vi "rio_veloster9.vi"() -> ()   [LabVIEW 2015]
uses:
  <vilib>/rvi/interface/nirviOpenFPGA/nirviOpenFPGA.xnode
  <vilib>/rvi/interface/nirviMethod/nirviMethod.xnode
  G_rio.vi
  <vilib>/rvi/interface/nirviReadWriteControl/nirviReadWriteControl.xnode
  <vilib>/Utility/error.llb/Error Cluster From Error Code.vi
  <vilib>/rvi/interface/Simulation/niFpgaSimulationCallBeginRW.vi
  <vilib>/rvi/errors/niLvFpgaAdjustHostInterfaceError.vi
  <vilib>/xnet/xnet.llb/XNET Frame Type CAN.ctl
  <vilib>/xnet/xnet.llb/XNET Frame CAN.ctl
  <vilib>/rvi/errors/niLvFpgaMergeErrorWithErrorCode.vi
  <resource>/objmgr/xnet.rc
  NiFpgaLv.dll
  <vilib>/FPGAPlugInAG/Dynamic/niLvFpga_ReadFifo_Dynamic.vi
  <vilib>/Instr/_visa.llb/VISA Configure Serial Port (Instr).vi
  <vilib>/Analysis/Matrix/NI_Matrix.lvlib
  <vilib>/Analysis/Matrix/Numeric/Multiply/Multiply - RM,RM.vi
  <vilib>/Analysis/Matrix/Numeric/Add/Add - RM,RM.vi
  <vilib>/Analysis/NI_AALBase.lvlib
  <vilib>/Analysis/Matrix/Numeric/Subtract/Subtract - RM,RM.vi
  <vilib>/Analysis/Matrix/Numeric/Conversions/Array To Matrix - RA.vi
  <vilib>/xnet/xnet.llb/XNET Create Session (Frame Input Stream).vi
  <vilib>/xnet/xnet.llb/XNET Create Session (Frame Output Stream).vi
  <vilib>/Analysis/Matrix/Numeric/Conversions/Array To Matrix - RA2.vi
  <vilib>/Analysis/baseanly.llb/Real Inverse Matrix.vi
  <vilib>/Analysis/Matrix/Numeric/Multiply/Multiply - R,RM.vi
  <vilib>/Analysis/Matrix/Numeric/Conversions/Matrix To Array - RM.vi
  <vilib>/xnet/xnet.llb/XNET Write (Frame CAN).vi
  <vilib>/xnet/xnet.llb/XNET Read (Frame CAN).vi
  <vilib>/FPGAPlugInAG/Dynamic/niLvFpga_Abort_Dynamic.vi
  <vilib>/FPGAPlugInAG/Dynamic/niLvFpga_Run_Dynamic.vi
  FPGA Bitfiles/autonomous_FPGATarget2_fpga4_FZHAM7r+pqE.lvbitx
  fpga/fpga4.vi
  <vilib>/FPGAPlugInAG/cRIO-9113/niLvFpga_Open_cRIO-9113.vi
  <vilib>/rvi/interface/common/dynamic/niFpgaDynamicAddResources.vi
panel:
  out "battery voltage 2":dbl
  out "FPGA VI Reference Out":refnum<k20>
  in  "Ref steer manual 2":dbl(knob) min=-20.48 max=20.46 step=0.01 scale=-20.48..20.46
  in  "steer2":bool
  in  "steer limit":dbl=100.0
  in  "buzz":bool
  out "hcount":u64=1
  out "hbias":dbl
  out "vcount":u64=1
  out "vgain":dbl=1.0
  in  "heading gain":dbl=1.414
  in  "pos gain":dbl=4.0
  out "dy":dbl
  out "dx":dbl
  out "initP":dbl
  out "dy_hat":dbl
  out "dx_hat":dbl
  out "dh":dbl
  out "initH":dbl
  out "dh_hat":dbl
  out "Pos_time 10":i32
  out "T PWM":u16
  out "B PWM":u16
  out "solenoid":bool
  out "brk enc":u8
  out "shift lever":dbl
  in  "LCM":bool=TRUE
  out "mobileye":u8[](array[numeric])
  out "timer":u32
  out "Mobileye_time 100":u32
  out "H_GPS":dbl
  out "pos":dbl[](array[numeric])
  out "pos error":dbl
  in  "GPS init":bool=TRUE
  in  "Gear Manual":i32(slide)=1 scale=-1.0..1.0
  out "map":i32=2
  out "P, R, D":i32
  out "heading error":dbl
  out "POS init":bool
  out "VS_CAN":dbl
  in  "brake":bool
  in  "Slide":dbl(slide) min=-50.0 max=50.0 step=50.0 scale=-50.0..50.0
  out "novatel":refnum<visa-resource-name>
  in  "ublox":bool=TRUE
  out "rest":u8[](array[numeric])
  out "GPS_novatel_time":u32
  out "GPS_Ublox_time 100":u32
  out "Con_time 10":i32
  out "CAN_time 10":u32
  out "gps2":refnum<visa-resource-name>
  out "gps1":refnum<visa-resource-name>
  out "Heading":dbl
  out "ecef ref":dbl[](array[numeric])
  out "h_gps":dbl
  out "pos_gps":dbl[](array[numeric]) format="%#_19f"
  out "get heading":bool
  out "get position":bool
  out "dt":dbl
  out "rt":dbl
  out "CAN Comm Enabled":bool
  in  "SPAS Enable":bool=TRUE
  in  "file write":bool
  out "data write":refnum<file>
  out "file rw error":errorcluster
  out "car can error":errorcluster
  out "CAN write":refnum<k21>
  out "CAN read":refnum<k21>
  out "Ref steer":dbl=1.0
  in  "Steer input":bool=TRUE
  in  "Ref steer manual":dbl(knob) scale=-550.0..550.0
  out "Ref vel":dbl=1.0
  in  "Ref vel manual":dbl
  in  "Velocity input":bool
  out "Auto":bool
  out "Run":bool
  out "E - STOP":bool
  out "Throttle Enable":bool=TRUE
  # "P"
  # "R"
  # "D"
  # "Ref steer manual"
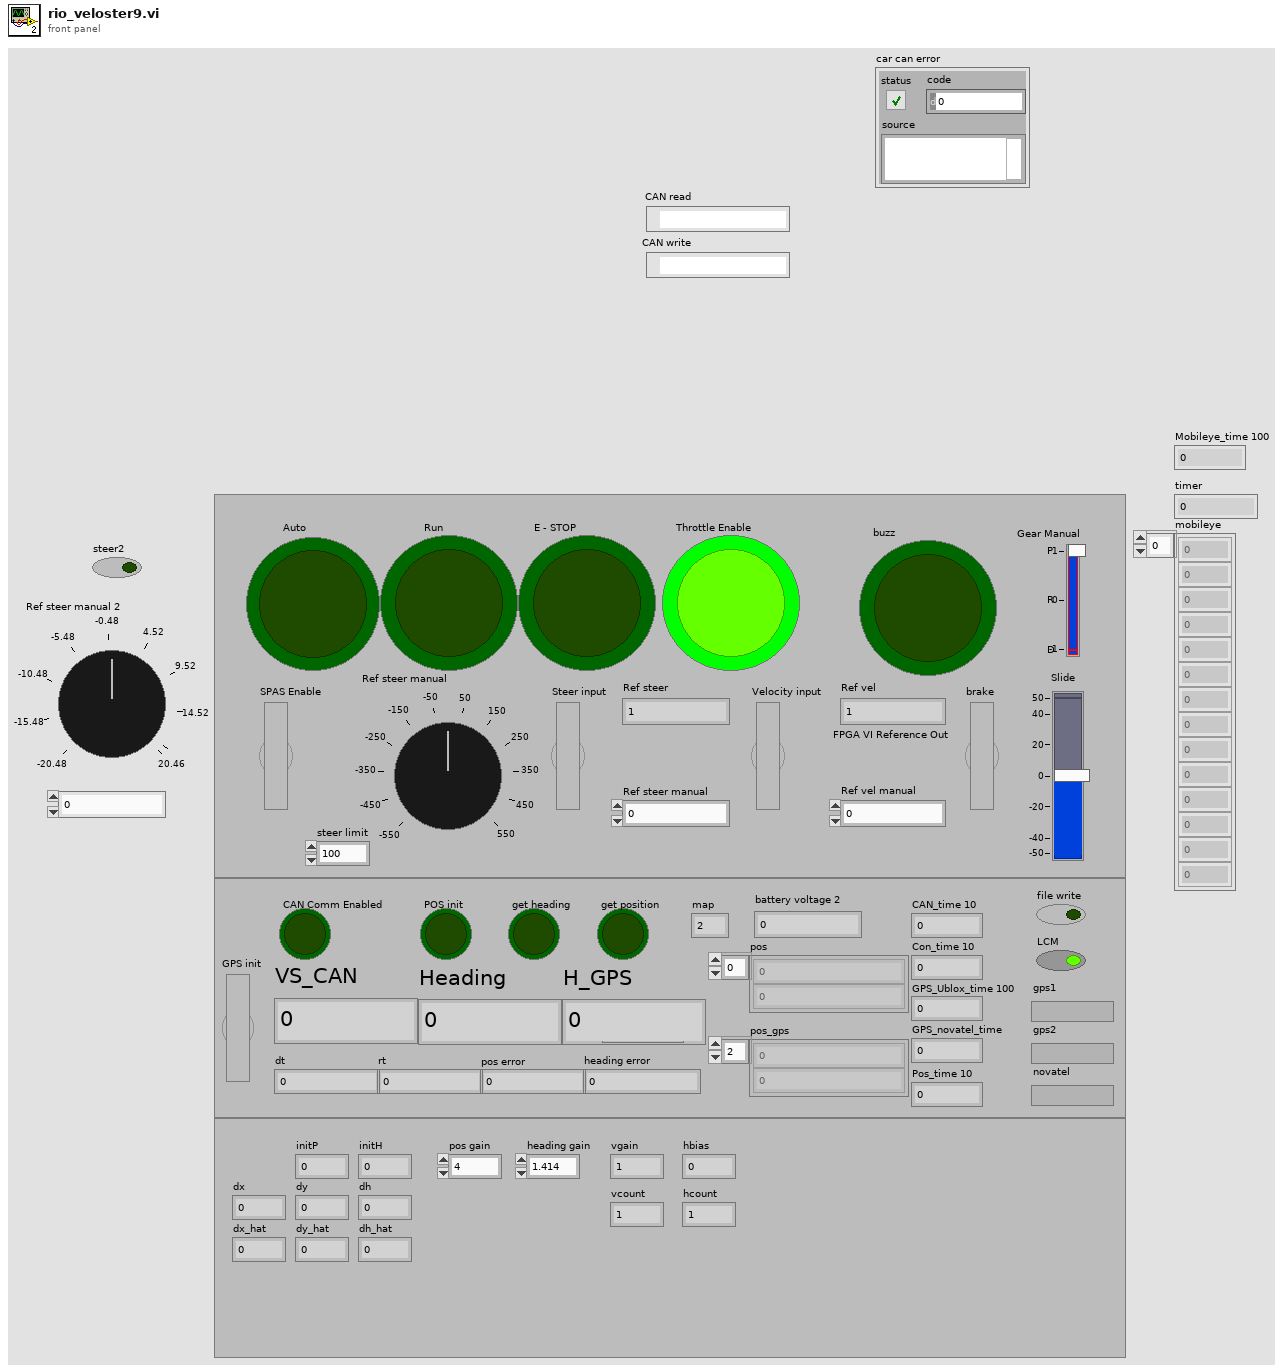
[diagram p1: front panel]
types:
  T1 = enum16{"open", "replace", "create", "open or create", "replace or create", "replace or create with confirmation"}
  T2 = typedef "XNET Frame CAN.ctl" = cluster{"timestamp":timestamp, "payload":u8[], "identifier":u32, "type":T3, "extended?":bool, "echo?":bool}
  T3 = typedef "XNET Frame Type CAN.ctl" = u8
  T4 = cluster{"connection ID":refnum<k16>, "net address":u32, "port":u16}
  T5 = cluster{"hash":i64, "sys time":i64, "mobileye":u8[]}
  T6 = cluster{"hash":i64, "sys time":i64, "time":dbl, "x":dbl, "y":dbl, "h":dbl, "numSV":i32, "postype":i32, "lag":i32, "hordev":dbl, "lat":dbl, "lon":dbl, "hgt":dbl, "map_idx":i32}
  T7 = cluster{"LCC[0]":dbl, "LCC[1]":dbl, "LCC[2]":dbl, "LCC[3]":dbl, "LCC[4]":dbl, "LCC[5]":dbl, "LCC[6]":dbl, "LCC[7]":dbl, "LCC[8]":dbl, "LCC[9]":dbl, "LCC[10]":dbl, "LCC[11]":dbl, "LCC[12]":dbl, "LCC[13]":dbl, "LCC[14]":dbl}
  T8 = cluster{"hash":i64, "sys time":i64, "time":dbl, "speed":dbl, "heading":dbl, "lat":dbl, "lon":dbl}
  T9 = cluster{"vel[0]":dbl, "vel[1]":dbl, "vel[2]":dbl, "vel[3]":dbl, "vel[4]":dbl, "vel[5]":dbl, "vel[6]":dbl}
  T10 = cluster{"output[0]":dbl, "output[1]":dbl, "output[2]":dbl, "output[3]":dbl, "output[4]":dbl, "output[5]":dbl, "output[6]":dbl, "output[7]":dbl, "output[8]":dbl, "output[9]":dbl, "output[10]":dbl, "output[11]":dbl, "output[12]":dbl, "output[13]":dbl, "output[14]":dbl}
  T11 = cluster{"output[0]":dbl, "output[1]":dbl, "output[2]":dbl, "output[3]":dbl, "output[4]":dbl, "output[5]":dbl, "output[6]":dbl}
  T12 = cluster{"hash":i64, "sys time":i64, "time":dbl, "yaw_rate":dbl, "mdps torque":dbl, "mdps str_ang":dbl, "VS_CAN":dbl, "lat_accel":dbl, "mcp":dbl, "accel pedal value":dbl, "tps":dbl, "odometer":dbl, "battery voltage":dbl, "WHL_SPD_RR":dbl, "WHL_SPD_RL":dbl, "WHL_SPD_FR":dbl, "WHL_SPD_FL":dbl}
  T13 = cluster{"hash":i64, "sys time":i64, "ref_vel":dbl, "ref_steer":dbl}
  T14 = cluster{"hash":i64, "sys time":i64, "Auto":bool, "Run":bool, "Solenoid":bool, "T lim":bool, "brk_enc":u8, "B PWM":u16, "T PWM":u16, "ref_vel":dbl, "ref_bkr_enc":dbl, "ref_apv":dbl, "ref_steer":dbl}
  T15 = typedef "NI_Matrix.lvlib/RealMatrix.ctl" = dbl[][]
  T16 = cluster{"hash":i64, "sys time":i64, "dt":dbl, "x":dbl, "y":dbl, "speed":dbl, "heading":dbl, "yaw_rate":dbl}
  T17 = cluster{"Real 2D Array[0]":dbl, "Real 2D Array[1]":dbl, "Real 2D Array[2]":dbl, "Real 2D Array[3]":dbl, "Real 2D Array[4]":dbl}
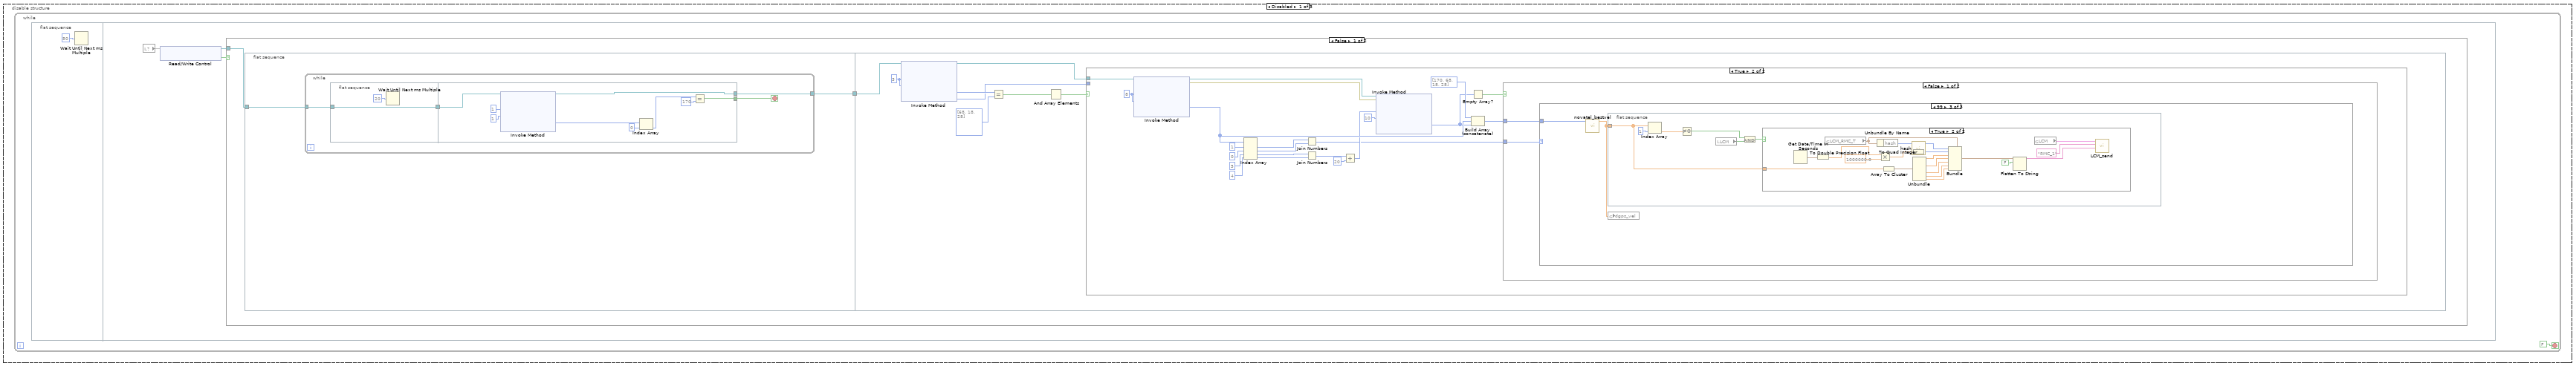
[diagram p5: hidden frame]
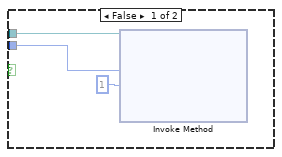
[diagram p6: hidden frame]
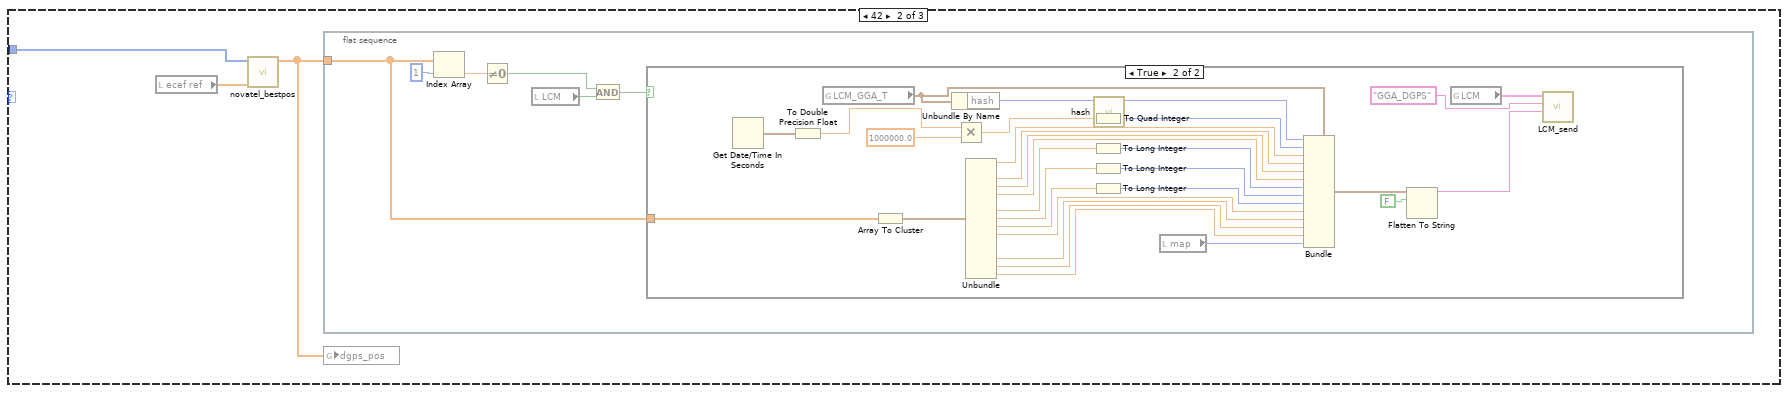
[diagram p8: hidden frame]
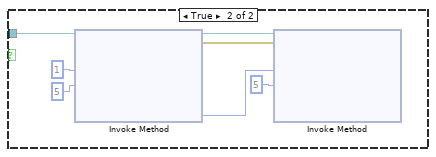
[diagram p12: hidden frame]
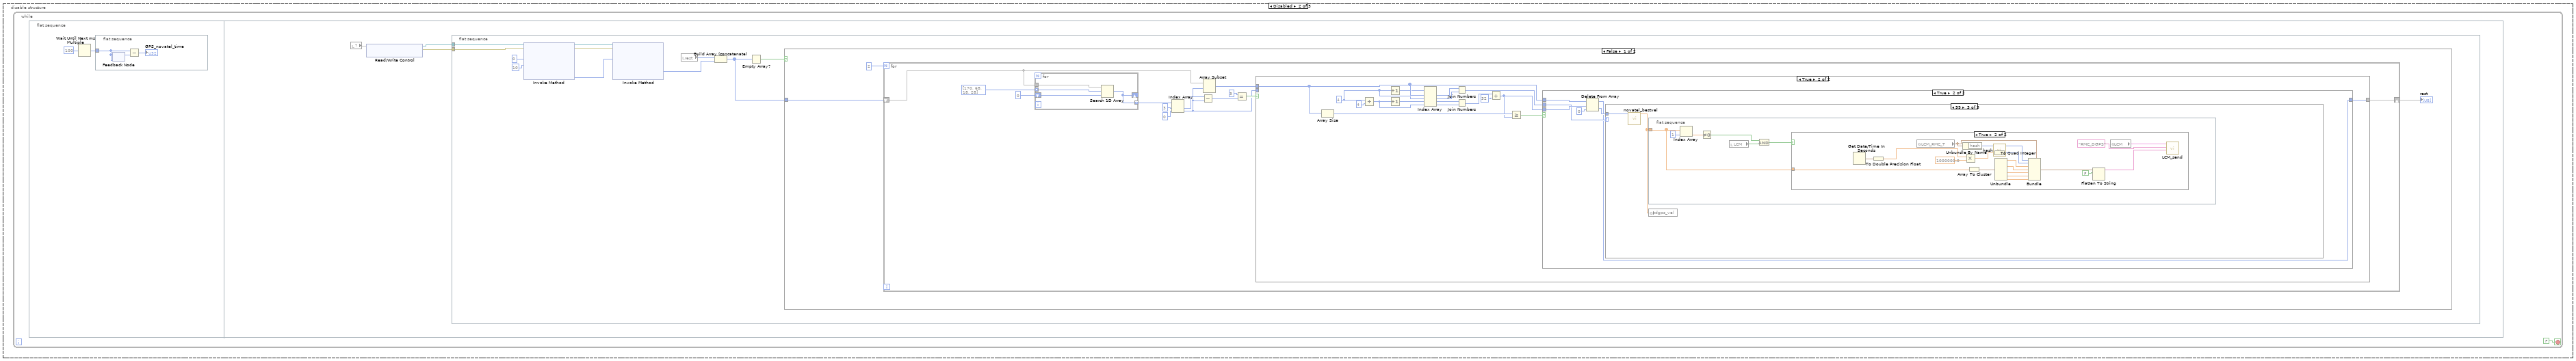
[diagram p13: hidden frame]
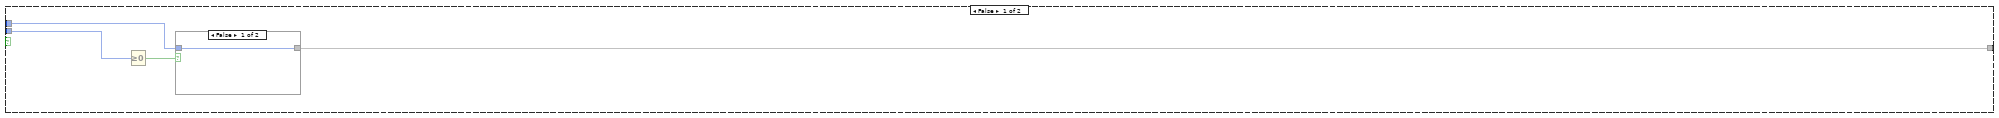
[diagram p14: hidden frame]
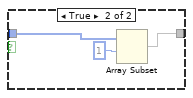
[diagram p15: hidden frame]
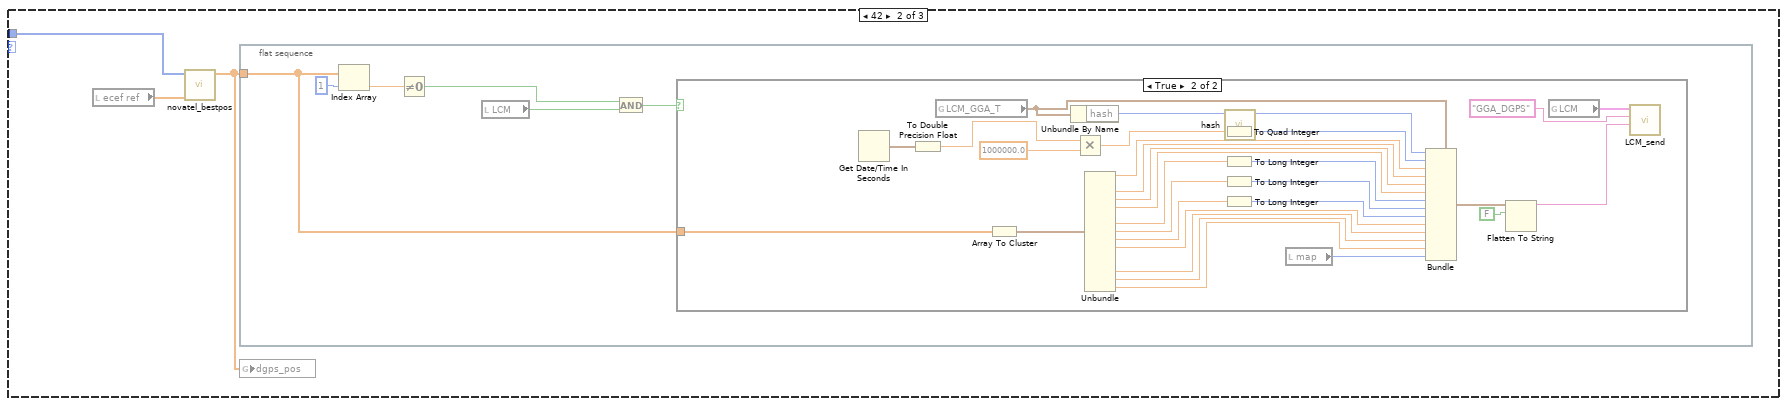
[diagram p18: hidden frame]
diagram:
  n1 = flat-sequence {
    frame #0 {
      n2 = xnode "Open FPGA VI Reference"() -> ("FPGA VI Reference Out"=w6:refnum<k20>, "error out"=w5:errorcluster)  [unwired: 2 in]
      n3 = xnode "Invoke Method"("FPGA VI Reference In"=w6, "error in"=w5) -> ("FPGA VI Reference Out"=w4:refnum<k20>, "error out"=w3:errorcluster)
      n4 = xnode "Invoke Method"("FPGA VI Reference In"=w4, "error in"=w3, "Wait Until Done (F)"=FALSE) -> ("FPGA VI Reference Out"=→"FPGA VI Reference Out":refnum<k20>)  [unwired: 1 out]
    }
    frame #1 {
      n5 = disable-structure shown="Enabled" {
        frame Enabled {
          n6 = call-poly "VISA Configure Serial Port"("VISA resource name"=refnum<visa-resource-name> "ASRL1::INSTR", "timeout (10sec)"=u32 10, "baud rate (9600)"=u32 9600) -> ("VISA resource name out"=→"novatel":refnum<visa-resource-name>)  [unwired: 11 in, 1 out]
          n7 = call-poly "VISA Configure Serial Port"("VISA resource name"=refnum<visa-resource-name> "USB0::0x1546::0x01A6::NI-VISA-1::1::RAW", "timeout (10sec)"=u32 1, "baud rate (9600)"=u32 115200) -> ("VISA resource name out"=→"gps1":refnum<visa-resource-name>)  [unwired: 11 in, 1 out]
          n8 = call-poly "VISA Configure Serial Port"("VISA resource name"=refnum<visa-resource-name> "USB0::0x1546::0x01A6::NI-VISA-0::1::RAW", "timeout (10sec)"=u32 1, "baud rate (9600)"=u32 115200) -> ("VISA resource name out"=→"gps2":refnum<visa-resource-name>)  [unwired: 11 in, 1 out]
        }
        frame Disabled {
        }
      }
      n9 = flat-sequence {
        frame #0 {
          w51 = 2 ("map")
          n10 = call "getecefdcmref.vi"("map"=w51) -> ("XYZ"=→"ecef ref":dbl[])  [unwired: 10 in, 4 out]
          "map" <- w51
        }
        frame #1 {
          w53 = FALSE ("GPS init")
          w54 = 0.0 ("Ref_vel_planner")
          n11 = global write "G_rio.vi" "T lim counter 2"(u16 300 ("T lim counter 2")) -> ()
          n12 = global write "G_rio.vi" "Ref_steer_planner"(w54) -> ()
          n13 = global write "G_rio.vi" "Ref_vel_planner"(w54) -> ()
          n14 = local write "brake"(w53) -> ()
          n15 = local write "rest"(u8[] [] ("rest")) -> ()
          n16 = local write "rest"(u8[] [] ("rest")) -> ()
          n17 = local write "Velocity input"(w53) -> ()
          n18 = local write "GPS init"(w53) -> ()
          "POS init" <- TRUE ("pos linit")
        }
      }
      n19 = flat-sequence {
        frame #0 {
          n20 = property class="XNET System"() -> (error out=w22:errorcluster, "Devices"=w35:refnum<k21>[])  [unwired: 2 in, 1 out]
          n21 = Index Array(array=w35, index=0) -> (element=w20:refnum<k21>)
          n22 = property class="XNET Device"(reference=w20, error in=w22) -> (error out=→"car can error":errorcluster, "Intfs"=w33:refnum<k21>[])  [unwired: 1 out]
          n23 = Index Array(array=w33, index=0) -> (element=w24:refnum<k21>)
          n24 = call-poly <vilib>:"XNET Create Session.vi"("cluster (:memory:)"=refnum<k21> "nixnet_example.CAN_Cluster", "interface"=w24) -> ("session out"=w25:refnum<k21>)  [unwired: 1 in, 12 out]
          n25 = call-poly <vilib>:"XNET Create Session.vi"("cluster (:memory:)"=refnum<k21> "nixnet_example.CAN_Cluster", "interface"=w24) -> ("session out"=w31:refnum<k21>)  [unwired: 1 in, 12 out]
          n26 = property class="XNET Session"(reference=w25, "Intf.BaudRate"=u32 500000 ("Interface:Baud Rate")) -> (reference out=w27:refnum<k21>)  [unwired: 1 in, 1 out]
          n27 = property class="XNET Session"(reference=w31, "Intf.BaudRate"=u32 500000 ("Interface:Baud Rate")) -> (reference out=w29:refnum<k21>)  [unwired: 1 in, 1 out]
          n28 = call <vilib>:"XNET Start.vi"("session in"=w27) -> ("session out"=→"CAN read":refnum<k21>)  [unwired: 1 in, 13 out]
          n29 = call <vilib>:"XNET Start.vi"("session in"=w29) -> ("session out"=→"CAN write":refnum<k21>)  [unwired: 1 in, 13 out]
        }
      }
      n30 = case shown="True" "file write" {
        frame False {
        }
        frame True {
          n31 = Open/Create/Replace File(file path (use dialog)=path "c:/datasave", operation (0:open)=T1."replace or create", access (0:read/write)=enum16{"read/write", "read-only", "write-only"}."write-only") -> (refnum out=→"data write":refnum<file>, cancelled=w61:bool, error out=→"file rw error":errorcluster)  [unwired: 3 in]
          n32 = Not(x=w61) -> (.not. x?=w60:bool)
          n33 = local write "file write"(w60) -> ()
        }
      }
      n34 = case shown="True" "LCM" {
        frame False {
        }
        frame True {
          n35 = flat-sequence {
            frame #0 {
              w15 = u16 7667 ("port")
              n36 = Decrement(x=w15) -> (x-1=w14:u16)
              n37 = UDP Open(11:w14) -> (port=w17:refnum<k16>)  [unwired: 4 in, 2 out]
              n38 = global read "G_rio.vi" "LCM"() -> (w19:T4)
              n39 = Bundle By Name(cluster=w19, "port"=w15, "connection ID"=w17, "net address"=u32 4294967295) -> (w18:T4)
              n40 = global write "G_rio.vi" "LCM"(w18) -> ()
            }
          }
          n41 = flat-sequence {
            frame #0 {
              w9 = u16 7668 ("port")
              n42 = global read "G_rio.vi" "LCM PC"() -> (w13:T4)
              n43 = UDP Open(11:w9) -> (port=w11:refnum<k16>)  [unwired: 4 in, 2 out]
              n44 = Bundle By Name(cluster=w13, "port"=w9, "connection ID"=w11, "net address"=u32 0) -> (w12:T4)
              n45 = global write "G_rio.vi" "LCM PC"(w12) -> ()
            }
          }
        }
      }
    }
    frame #2 {
      (unwired) FALSE
      n46 = disable-structure shown="Enabled" {
        frame Enabled {
          n47 = while {
            stop <- FALSE stop-if-true
            n48 = flat-sequence {
              frame #0 {
                n49 = Wait Until Next ms Multiple(millisecond multiple=u32 100) -> (millisecond timer value=w1290:u32)
                n50 = flat-sequence {
                  tunnel: w1290 -> [w1292]
                  frame #0 {
                    n51 = feedback #1(w1292) -> (w1293:u32)
                    n52 = feedback-in #1(w1292) -> ()
                    n53 = Subtract(x=w1292, y=w1293) -> (x-y=→"Mobileye_time 100":u32)
                  }
                }
              }
              frame #1 {
                n54 = local read "FPGA VI Reference Out"() -> (w1339:refnum<k20>)
                n55 = xnode "Read/Write Control"("FPGA VI Reference In"=w1339) -> ("m 700"=w1299:u8[], "m 760"=w1335:u8[], "m 710"=w1324:u8[], "m 711"=w1320:u8[], "m 720"=w1318:u8[], "m 721"=w1317:u8[], "m 722"=w1316:u8[], "m 723"=w1315:u8[], "m 724"=w1314:u8[], "m 725"=w1313:u8[], "m 726"=w1312:u8[], "m 727"=w1311:u8[], "m 728"=w1310:u8[], "m 729"=w1309:u8[])  [unwired: 1 in, 2 out]
                n56 = Build Array(w1318, w1317, w1316, w1315, w1314, w1313, w1312, w1311, w1310, w1309) -> (w1308:u8[][])
                n57 = Index Array(array=w1299, index #1=4 ("index"), index #4=8 ("index"), index #5=11 ("index")) -> (element #1=w1332:u8, element #2=w1331:u8, element #3=w1330:u8, element #4=w1329:u8, element #5=w1328:u8)  [unwired: 2 in]
                n58 = Array Subset(array=w1320, index=6, length=6) -> (w1319:u8[])
                n59 = Array Subset(array=w1299, index=0, length=4) -> (w1296:u8[])
                n60 = Array Subset(array=w1335, index=4, length=3) -> (w1327:u8[])
                n61 = Array Subset(array=w1324, index=5, length=7) -> (w1323:u8[])
                n62 = Index Array(array=w1296, index #1=0 ("index")) -> (element #1=w1305:u8, element #2=w1304:u8, element #3=w1303:u8, element #4=w1302:u8)  [unwired: 3 in]
                n63 = Build Array (concatenate)(w1296, w1332, w1331, w1330, w1329, w1328, w1327, w1323, w1319) -> (w1307:u8[])
                n64 = Join Numbers(hi=w1305, lo=w1304) -> ((hi.lo)=w1301:u16)
                n65 = Join Numbers(hi=w1303, lo=w1302) -> ((hi.lo)=w1300:u16)
                n66 = for {
                  tunnel: w1308 -> [w1341] mode=indexing
                  shift-right: [w1344] -> w1294
                  shift-left: w1307 -> [w1345]
                  n67 = Array Subset(array=w1341, index=4, length=8) -> (w1340:u8[])
                  n68 = disable-structure shown="Enabled" {
                    disable-tunnel: [w1348 TRUE ("lsb carry out")] -> w1346
                    disable-tunnel: w1340 -> [w1347 _]
                    frame Disabled {
                      n69 = Index Array(array=w1347, index=0) -> (element=w1350:u8)
                      n70 = Rotate Right With Carry(2:w1350, 3:FALSE ("carry")) -> (1:w1348:bool)  [unwired: 1 out]
                    }
                    frame Enabled {
                    }
                  }
                  n71 = case shown="True" w1346 {
                    tunnel: w1345 -> [w1353 w1356]
                    tunnel: [w1353 w1355] -> w1344
                    tunnel: w1340 -> [_ w1354]
                    frame False {
                    }
                    frame True {
                      n72 = Build Array (concatenate)(w1356, w1354) -> (w1355:u8[])
                    }
                  }
                }
                "mobileye" <- w1294
                n73 = Join Numbers(hi=w1301, lo=w1300) -> ((hi.lo)=→"timer":u32)
              }
              frame #2 {
                n74 = local read "LCM"() -> (w1357:bool)
                n75 = case shown="True" w1357 {
                  frame False {
                    n76 = local read "mobileye"() -> (w1358:u8[])
                    n77 = shared-variable "veloster\\sharedvari.lvlib\\mobileye"(w1358) -> ()  [unwired: 1 in, 1 out]
                  }
                  frame True {
                    n78 = Get Date/Time In Seconds() -> (seconds since 1Jan1904=w1363:timestamp)
                    n79 = To Double Precision Float(number=w1363) -> (double precision float=w1362:dbl)
                    n80 = global read "G_rio.vi" "LCM_EYE_RAW_T"() -> (w1372:T5)
                    n81 = Unbundle By Name(w1372) -> ("hash"=w1371:i64)
                    n82 = Multiply(x=w1362, y=1000000.0) -> (x*y=w1360:dbl)
                    n83 = local read "mobileye"() -> (w1364:u8[])
                    n84 = call "hash.vi"("input"=w1371) -> ("output"=w1370:i64)  [unwired: 10 in]
                    n85 = To Quad Integer(1:w1360) -> (0:w1359:i64)
                    n86 = Bundle By Name(cluster=w1372, "hash"=w1370, "sys time"=w1359, "mobileye"=w1364) -> (w1369:T5)
                    n87 = Flatten To String(anything=w1369, prepend array or string size? (T)=FALSE) -> (data string=w1367:string)  [unwired: 2 in, 2 out]
                    n88 = global read "G_rio.vi" "LCM"() -> (w1368:T4)
                    n89 = call "LCM_send.vi"("DATA"=w1367, "ID"="EYE_RAW_T", "LCM"=w1368) -> ()  [unwired: 6 in, 3 out]
                  }
                }
              }
            }
          }
        }
        frame Disabled {
        }
      }
      n90 = disable-structure shown="Enabled" {
        frame Disabled {
          n91 = while {
            stop <- FALSE stop-if-true
            n92 = flat-sequence {
              frame #0 {
                n93 = Wait Until Next ms Multiple(millisecond multiple=u32 50) -> ()  [unwired: 1 out]
              }
              frame #1 {
                n94 = local read item#-1() -> (w79)
                n95 = xnode "Read/Write Control"("FPGA VI Reference In"=w79) -> ("FPGA VI Reference Out"=w77:refnum<k20>, "Connection error GPS 1"=w78:bool)  [unwired: 1 in, 1 out]
                n96 = case shown="False" w78 {
                  tunnel: w77 -> [w81 w201]
                  frame False {
                    n97 = flat-sequence {
                      tunnel: w81 -> [w83]
                      tunnel: [w82] -> w80
                      tunnel: w80 -> [w102]
                      frame #0 {
                        n98 = while {
                          tunnel: w83 -> [w87]
                          tunnel: [w85] -> w82
                          stop <- w86 stop-if-true
                          n99 = flat-sequence {
                            tunnel: w87 -> [w89]
                            tunnel: [w89] -> w84
                            tunnel: [w92] -> w86
                            tunnel: [w91] -> w85
                            tunnel: w84 -> [w98]
                            frame #0 {
                              n100 = Wait Until Next ms Multiple(millisecond multiple=u32 20) -> ()  [unwired: 1 out]
                            }
                            frame #1 {
                              n101 = xnode "Invoke Method"("FPGA VI Reference In"=w98, "Number of Elements"=u32 1, "Timeout (ms)"=1) -> ("FPGA VI Reference Out"=w91:refnum<k20>, "Data"=w93:u8[])  [unwired: 1 in, 2 out]
                              n102 = Index Array(array=w93, index=0) -> (element=w95:u8)
                              n103 = Equal?(x=w95, y=u8 170) -> (x = y?=w92:bool)
                            }
                          }
                        }
                      }
                      frame #1 {
                        w103 = u32 3 ("Number of Elements")
                        n104 = xnode "Invoke Method"("FPGA VI Reference In"=w102, "Number of Elements"=w103, "Timeout (ms)"=w103) -> ("FPGA VI Reference Out"=w101:refnum<k20>, "Data"=w105:u8[], "Elements Remaining"=w99:u32)  [unwired: 1 in, 1 out]
                        n105 = Equal?(x=w105, y=u8[] [68, 18, 28]) -> (x = y?=w106:bool[])
                        n106 = And Array Elements(Boolean array=w106) -> (logical AND=w100:bool)
                        n107 = case shown="True" w100 {
                          tunnel: w101 -> [w109 w114]
                          tunnel: w99 -> [w108 _]
                          frame False {
                            n108 = xnode "Invoke Method"("FPGA VI Reference In"=w109, "Number of Elements"=w108, "Timeout (ms)"=1) -> ()  [unwired: 1 in, 4 out]
                          }
                          frame True {
                            w110 = u32 8 ("Number of Elements")
                            n109 = xnode "Invoke Method"("FPGA VI Reference In"=w114, "Number of Elements"=w110, "Timeout (ms)"=w110) -> ("FPGA VI Reference Out"=w127:refnum<k20>, "error out"=w128:errorcluster, "Data"=w130:u8[])  [unwired: 1 in, 1 out]
                            n110 = Index Array(array=w130, index #1=1 ("index"), index #2=0 ("index"), index #3=5 ("index"), index #4=4 ("index")) -> (element #1=w117:u8, element #2=w118:u8, element #3=w122:u8, element #4=w123:u8)
                            n111 = Join Numbers(hi=w117, lo=w118) -> ((hi.lo)=w119:u16)
                            n112 = Join Numbers(hi=w122, lo=w123) -> ((hi.lo)=w124:u16)
                            n113 = Add(x=w124, y=u16 20) -> (x+y=w126:u16)
                            n114 = xnode "Invoke Method"("FPGA VI Reference In"=w127, "error in"=w128, "Number of Elements"=w126, "Timeout (ms)"=10) -> ("Data"=w112:u8[])  [unwired: 3 out]
                            n115 = Empty Array?(array=w112) -> (empty?=w111:bool)
                            n116 = Build Array (concatenate)(u8[] [170, 68, 18, 28], w130, w112) -> (w131:u8[])
                            n117 = case shown="False" w111 {
                              tunnel: w131 -> [w133 _]
                              tunnel: w119 -> [w132 _]
                              frame False {
                                n118 = case shown="99" w132 {
                                tunnel: w133 -> [_ w136 w174]
                                frame 0, Default {
                                }
                                frame 42 {
                                n119 = local read "ecef ref"() -> (w135:dbl[])
                                n120 = call "novatel_bestpos.vi"("ecef ref"=w135, "gps_data"=w136) -> ("LCC"=w134:dbl[])  [unwired: 9 in]
                                n121 = flat-sequence {
                                tunnel: w134 -> [w139]
                                frame #0 {
                                n122 = Index Array(array=w139, index=1) -> (element=w142:dbl)
                                n123 = Not Equal To 0?(x=w142) -> (x != 0?=w138:bool)
                                n124 = local read "LCM"() -> (w141:bool)
                                n125 = And(x=w138, y=w141) -> (x .and. y?=w137:bool)
                                n126 = case shown="True" w137 {
                                tunnel: w139 -> [_ w162]
                                frame False {
                                }
                                frame True {
                                n127 = Get Date/Time In Seconds() -> (seconds since 1Jan1904=w147:timestamp)
                                n128 = To Double Precision Float(number=w147) -> (double precision float=w146:dbl)
                                n129 = global read "G_rio.vi" "LCM_GGA_T"() -> (w171:T6)
                                n130 = Array To Cluster(array=w162) -> (cluster=w170:T7)
                                n131 = Unbundle By Name(w171) -> ("hash"=w167:i64)
                                n132 = Multiply(x=w146, y=1000000.0) -> (x*y=w144:dbl)
                                n133 = Unbundle(w170) -> ("LCC[0]"=w172:dbl, "LCC[2]"=w161:dbl, "LCC[3]"=w160:dbl, "LCC[4]"=w159:dbl, "LCC[6]"=w158:dbl, "LCC[7]"=w156:dbl, "LCC[8]"=w154:dbl, "LCC[9]"=w152:dbl, "LCC[12]"=w151:dbl, "LCC[13]"=w150:dbl, "LCC[14]"=w149:dbl)  [unwired: 4 out]
                                n134 = To Quad Integer(1:w144) -> (0:w143:i64)
                                n135 = To Long Integer(number=w158) -> (32bit integer=w157:i32)
                                n136 = To Long Integer(number=w156) -> (32bit integer=w155:i32)
                                n137 = To Long Integer(number=w154) -> (32bit integer=w153:i32)
                                n138 = call "hash.vi"("input"=w167) -> ("output"=w166:i64)  [unwired: 10 in]
                                n139 = local read "map"() -> (w148:i32)
                                n140 = Bundle(cluster=w171, "hash"=w166, "sys time"=w143, "time"=w172, "x"=w161, "y"=w160, "h"=w159, "numSV"=w157, "postype"=w155, "lag"=w153, "hordev"=w152, "lat"=w151, "lon"=w150, "hgt"=w149, "map_idx"=w148) -> (w168:T6)
                                n141 = Flatten To String(anything=w168, prepend array or string size? (T)=FALSE) -> (data string=w164:string)  [unwired: 2 in, 2 out]
                                n142 = global read "G_rio.vi" "LCM"() -> (w163:T4)
                                n143 = call "LCM_send.vi"("DATA"=w164, "ID"="GGA_DGPS", "LCM"=w163) -> ()  [unwired: 6 in, 3 out]
                                }
                                }
                                }
                                }
                                n144 = global write "G_rio.vi" "dgps_pos"(w134) -> ()
                                }
                                frame 99 {
                                n145 = call "novatel_bestvel.vi"("gps_data"=w174) -> ("vel"=w173:dbl[])  [unwired: 10 in]
                                n146 = flat-sequence {
                                tunnel: w173 -> [w176]
                                frame #0 {
                                n147 = Index Array(array=w176, index=1) -> (element=w179:dbl)
                                n148 = Not Equal To 0?(x=w179) -> (x != 0?=w180:bool)
                                n149 = local read "LCM"() -> (w178:bool)
                                n150 = And(x=w180, y=w178) -> (x .and. y?=w175:bool)
                                n151 = case shown="True" w175 {
                                tunnel: w176 -> [_ w199]
                                frame False {
                                }
                                frame True {
                                n152 = Get Date/Time In Seconds() -> (seconds since 1Jan1904=w185:timestamp)
                                n153 = To Double Precision Float(number=w185) -> (double precision float=w184:dbl)
                                n154 = global read "G_rio.vi" "LCM_RMC_T"() -> (w200:T8)
                                n155 = Unbundle By Name(w200) -> ("hash"=w196:i64)
                                n156 = Multiply(x=w184, y=1000000.0) -> (x*y=w182:dbl)
                                n157 = Array To Cluster(array=w199) -> (cluster=w198:T9)
                                n158 = call "hash.vi"("input"=w196) -> ("output"=w195:i64)  [unwired: 10 in]
                                n159 = To Quad Integer(1:w182) -> (0:w181:i64)
                                n160 = Unbundle(w198) -> ("vel[0]"=w190:dbl, "vel[2]"=w189:dbl, "vel[4]"=w188:dbl, "vel[5]"=w187:dbl, "vel[6]"=w186:dbl)  [unwired: 2 out]
                                n161 = Bundle(cluster=w200, "hash"=w195, "sys time"=w181, "time"=w190, "speed"=w189, "heading"=w188, "lat"=w187, "lon"=w186) -> (w191:T8)
                                n162 = Flatten To String(anything=w191, prepend array or string size? (T)=FALSE) -> (data string=w193:string)  [unwired: 2 in, 2 out]
                                n163 = global read "G_rio.vi" "LCM"() -> (w192:T4)
                                n164 = call "LCM_send.vi"("DATA"=w193, "ID"="RMC_1", "LCM"=w192) -> ()  [unwired: 6 in, 3 out]
                                }
                                }
                                }
                                }
                                n165 = global write "G_rio.vi" "dgps_vel"(w173) -> ()
                                }
                                }
                              }
                              frame True {
                              }
                            }
                          }
                        }
                      }
                    }
                  }
                  frame True {
                    n166 = xnode "Invoke Method"("FPGA VI Reference In"=w201, "Number of Elements"=u32 1, "Timeout (ms)"=5) -> ("FPGA VI Reference Out"=w205:refnum<k20>, "error out"=w206:errorcluster, "Elements Remaining"=w207:u32)  [unwired: 1 in, 1 out]
                    n167 = xnode "Invoke Method"("FPGA VI Reference In"=w205, "error in"=w206, "Number of Elements"=w207, "Timeout (ms)"=5) -> ()  [unwired: 4 out]
                  }
                }
              }
            }
          }
        }
        frame Disabled {
          n168 = while {
            stop <- FALSE stop-if-true
            n169 = flat-sequence {
              frame #0 {
                n170 = Wait Until Next ms Multiple(millisecond multiple=u32 100) -> (millisecond timer value=w209:u32)
                n171 = flat-sequence {
                  tunnel: w209 -> [w212]
                  frame #0 {
                    n172 = feedback #2(w212) -> (w213:u32)
                    n173 = feedback-in #2(w212) -> ()
                    n174 = Subtract(x=w212, y=w213) -> (x-y=→"GPS_novatel_time":u32)
                  }
                }
              }
              frame #1 {
                n175 = local read item#-1() -> (w216)
                n176 = xnode "Read/Write Control"("FPGA VI Reference In"=w216) -> ("FPGA VI Reference Out"=w215:refnum<k20>, "error out"=w214:errorcluster)  [unwired: 1 in, 1 out]
                n177 = flat-sequence {
                  tunnel: w215 -> [w227]
                  tunnel: w214 -> [w226]
                  frame #0 {
                    n178 = xnode "Invoke Method"("FPGA VI Reference In"=w227, "error in"=w226, "Number of Elements"=u32 0, "Timeout (ms)"=10) -> ("FPGA VI Reference Out"=w225:refnum<k20>, "error out"=w224:errorcluster, "Elements Remaining"=w223:u32)  [unwired: 1 out]
                    n179 = xnode "Invoke Method"("FPGA VI Reference In"=w225, "error in"=w224, "Number of Elements"=w223) -> ("Data"=w217:u8[])  [unwired: 1 in, 3 out]
                    n180 = local read "rest"() -> (w219:u8[])
                    n181 = Build Array (concatenate)(w219, w217) -> (w218:u8[])
                    n182 = Empty Array?(array=w218) -> (empty?=w220:bool)
                    n183 = case shown="False" w220 {
                      tunnel: w218 -> [w230 _]
                      frame False {
                        n184 = for {
                          N: 2 -> [_]
                          shift-right: [w234] -> w228
                          shift-left: w230 -> [w232]
                          n185 = for {
                            tunnel: w232 -> [w345]
                            tunnel: u8[] [170, 68, 18, 28] -> [w343] mode=indexing
                            shift-right: [w342] -> _
                            shift-left: 0 ("start index (0)") -> [w344]
                            tunnel: [w342] -> w241 mode=indexing
                            n186 = Search 1D Array(1D array=w345, element=w343, start index (0)=w344) -> (index of element=w342:i32)
                          }
                          n187 = Index Array(array=w241, index #1=3 ("index"), index #2=0 ("index")) -> (element #1=w238:i32, element #2=w231:i32)
                          n188 = Subtract(x=w238, y=w231) -> (x-y=w237:i32)
                          n189 = Array Subset(array=w232, index=w231) -> (w233:u8[])  [unwired: 1 in]
                          n190 = Equal?(x=3, y=w237) -> (x = y?=w235:bool)
                          n191 = case shown="True" w235 {
                            tunnel: w233 -> [w247 w256]
                            tunnel: [w246 w253] -> w234
                            tunnel: w231 -> [w245 _]
                            frame False {
                              n192 = Greater Or Equal To 0?(x=w245) -> (x >= 0?=w244:bool)
                              n193 = case shown="False" w244 {
                                tunnel: w247 -> [w248 w251]
                                tunnel: [w248 w249] -> w246
                                frame False {
                                }
                                frame True {
                                n194 = Array Subset(array=w251, index=1 ("length")) -> (w249:u8[])  [unwired: 1 in]
                                }
                              }
                            }
                            frame True {
                              w252 = 4 ("index")
                              n195 = Array Size(array=w256) -> (size(s)=w258:i32)
                              n196 = Add(x=w252, y=4) -> (x+y=w265:i32)
                              n197 = Increment(x=w252) -> (x+1=w268:i32)
                              n198 = Increment(x=w265) -> (x+1=w266:i32)
                              n199 = Index Array(array=w256, index #1=w268, index #2=w252, index #3=w266, index #4=w265) -> (element #1=w264:u8, element #2=w263:u8, element #3=w262:u8, element #4=w261:u8)
                              n200 = Join Numbers(hi=w264, lo=w263) -> ((hi.lo)=w254:u16)
                              n201 = Join Numbers(hi=w262, lo=w261) -> ((hi.lo)=w260:u16)
                              n202 = Add(x=w260, y=u16 32) -> (x+y=w255:u16)
                              n203 = Greater Or Equal?(x=w258, y=w255) -> (x >= y?=w257:bool)
                              n204 = case shown="True" w257 {
                                tunnel: w256 -> [_ w274]
                                tunnel: w255 -> [_ w273]
                                tunnel: w254 -> [_ w270]
                                tunnel: [_ w269] -> w253
                                frame False {
                                }
                                frame True {
                                n205 = Delete From Array(array=w274, length=w273, index=0) -> (deleted portion=w271:u8[], array with subset deleted=w269:u8[])
                                n206 = case shown="99" w270 {
                                tunnel: w271 -> [_ w277 w315]
                                frame 0, Default {
                                }
                                frame 42 {
                                n207 = local read "ecef ref"() -> (w276:dbl[])
                                n208 = call "novatel_bestpos.vi"("ecef ref"=w276, "gps_data"=w277) -> ("LCC"=w275:dbl[])  [unwired: 9 in]
                                n209 = flat-sequence {
                                tunnel: w275 -> [w280]
                                frame #0 {
                                n210 = Index Array(array=w280, index=1) -> (element=w283:dbl)
                                n211 = Not Equal To 0?(x=w283) -> (x != 0?=w279:bool)
                                n212 = local read "LCM"() -> (w282:bool)
                                n213 = And(x=w279, y=w282) -> (x .and. y?=w278:bool)
                                n214 = case shown="True" w278 {
                                tunnel: w280 -> [_ w303]
                                frame False {
                                }
                                frame True {
                                n215 = Get Date/Time In Seconds() -> (seconds since 1Jan1904=w288:timestamp)
                                n216 = To Double Precision Float(number=w288) -> (double precision float=w287:dbl)
                                n217 = global read "G_rio.vi" "LCM_GGA_T"() -> (w312:T6)
                                n218 = Array To Cluster(array=w303) -> (cluster=w311:T7)
                                n219 = Unbundle By Name(w312) -> ("hash"=w308:i64)
                                n220 = Multiply(x=w287, y=1000000.0) -> (x*y=w285:dbl)
                                n221 = Unbundle(w311) -> ("LCC[0]"=w313:dbl, "LCC[2]"=w302:dbl, "LCC[3]"=w301:dbl, "LCC[4]"=w300:dbl, "LCC[6]"=w299:dbl, "LCC[7]"=w297:dbl, "LCC[8]"=w295:dbl, "LCC[9]"=w293:dbl, "LCC[12]"=w292:dbl, "LCC[13]"=w291:dbl, "LCC[14]"=w290:dbl)  [unwired: 4 out]
                                n222 = To Quad Integer(1:w285) -> (0:w284:i64)
                                n223 = To Long Integer(number=w299) -> (32bit integer=w298:i32)
                                n224 = To Long Integer(number=w297) -> (32bit integer=w296:i32)
                                n225 = To Long Integer(number=w295) -> (32bit integer=w294:i32)
                                n226 = call "hash.vi"("input"=w308) -> ("output"=w307:i64)  [unwired: 10 in]
                                n227 = local read "map"() -> (w289:i32)
                                n228 = Bundle(cluster=w312, "hash"=w307, "sys time"=w284, "time"=w313, "x"=w302, "y"=w301, "h"=w300, "numSV"=w298, "postype"=w296, "lag"=w294, "hordev"=w293, "lat"=w292, "lon"=w291, "hgt"=w290, "map_idx"=w289) -> (w309:T6)
                                n229 = Flatten To String(anything=w309, prepend array or string size? (T)=FALSE) -> (data string=w305:string)  [unwired: 2 in, 2 out]
                                n230 = global read "G_rio.vi" "LCM"() -> (w304:T4)
                                n231 = call "LCM_send.vi"("DATA"=w305, "ID"="GGA_DGPS", "LCM"=w304) -> ()  [unwired: 6 in, 3 out]
                                }
                                }
                                }
                                }
                                n232 = global write "G_rio.vi" "dgps_pos"(w275) -> ()
                                }
                                frame 99 {
                                n233 = call "novatel_bestvel.vi"("gps_data"=w315) -> ("vel"=w314:dbl[])  [unwired: 10 in]
                                n234 = flat-sequence {
                                tunnel: w314 -> [w318]
                                frame #0 {
                                n235 = Index Array(array=w318, index=1) -> (element=w320:dbl)
                                n236 = Not Equal To 0?(x=w320) -> (x != 0?=w321:bool)
                                n237 = local read "LCM"() -> (w316:bool)
                                n238 = And(x=w321, y=w316) -> (x .and. y?=w317:bool)
                                n239 = case shown="True" w317 {
                                tunnel: w318 -> [_ w340]
                                frame False {
                                }
                                frame True {
                                n240 = Get Date/Time In Seconds() -> (seconds since 1Jan1904=w326:timestamp)
                                n241 = To Double Precision Float(number=w326) -> (double precision float=w325:dbl)
                                n242 = global read "G_rio.vi" "LCM_RMC_T"() -> (w341:T8)
                                n243 = Unbundle By Name(w341) -> ("hash"=w337:i64)
                                n244 = Multiply(x=w325, y=1000000.0) -> (x*y=w323:dbl)
                                n245 = Array To Cluster(array=w340) -> (cluster=w339:T9)
                                n246 = To Quad Integer(1:w323) -> (0:w322:i64)
                                n247 = call "hash.vi"("input"=w337) -> ("output"=w336:i64)  [unwired: 10 in]
                                n248 = Unbundle(w339) -> ("vel[0]"=w331:dbl, "vel[2]"=w330:dbl, "vel[4]"=w329:dbl, "vel[5]"=w328:dbl, "vel[6]"=w327:dbl)  [unwired: 2 out]
                                n249 = Bundle(cluster=w341, "hash"=w336, "sys time"=w322, "time"=w331, "speed"=w330, "heading"=w329, "lat"=w328, "lon"=w327) -> (w332:T8)
                                n250 = Flatten To String(anything=w332, prepend array or string size? (T)=FALSE) -> (data string=w334:string)  [unwired: 2 in, 2 out]
                                n251 = global read "G_rio.vi" "LCM"() -> (w333:T4)
                                n252 = call "LCM_send.vi"("DATA"=w334, "ID"="RMC_DGPS", "LCM"=w333) -> ()  [unwired: 6 in, 3 out]
                                }
                                }
                                }
                                }
                                n253 = global write "G_rio.vi" "dgps_vel"(w314) -> ()
                                }
                                }
                                }
                              }
                            }
                          }
                        }
                        "rest" <- w228
                      }
                      frame True {
                      }
                    }
                  }
                }
              }
            }
          }
        }
        frame Enabled {
          n254 = while {
            stop <- FALSE stop-if-true
            n255 = flat-sequence {
              frame #0 {
                n256 = Wait Until Next ms Multiple(millisecond multiple=u32 50) -> (millisecond timer value=w347:u32)
                n257 = flat-sequence {
                  tunnel: w347 -> [w350]
                  frame #0 {
                    n258 = feedback #3(w350) -> (w351:u32)
                    n259 = feedback-in #3(w350) -> ()
                    n260 = Subtract(x=w350, y=w351) -> (x-y=→"GPS_Ublox_time 100":u32)
                  }
                }
              }
              frame #1 {
                n261 = for {
                  N: 5 -> [_]
                  stop <- w426 stop-if-true
                  n262 = local read "gps2"() -> (w425:refnum<visa-resource-name>)
                  n263 = VISA Read(VISA resource name=w425, byte count=u32 100) -> (read buffer=w432:string, error out=w427:errorcluster)  [unwired: 1 in, 2 out]
                  n264 = local read "ecef ref"() -> (w431:dbl[])
                  n265 = Unbundle By Name(w427) -> ("status"=w426:bool)
                  n266 = call "nmea.vi"("ecef ref"=w431, "NMEA"=w432) -> ("output"=w429:dbl[], "type"=w430:u32)  [unwired: 8 in]
                  n267 = case shown="1" w430 {
                    tunnel: w429 -> [_ w433 w474]
                    frame 0, Default {
                    }
                    frame 1 {
                      n268 = global write "G_rio.vi" "gps_pos 2"(w433) -> ()
                      n269 = Index Array(array=w433, index=1) -> (element=w435:dbl)
                      n270 = Not Equal To 0?(x=w435) -> (x != 0?=w434:bool)
                      n271 = local read "LCM"() -> (w436:bool)
                      n272 = And(x=w434, y=w436) -> (x .and. y?=w438:bool)
                      n273 = case shown="True" w438 {
                        tunnel: w433 -> [_ w458]
                        frame False {
                        }
                        frame True {
                          n274 = Get Date/Time In Seconds() -> (seconds since 1Jan1904=w443:timestamp)
                          n275 = To Double Precision Float(number=w443) -> (double precision float=w442:dbl)
                          n276 = global read "G_rio.vi" "LCM_GGA_T"() -> (w467:T6)
                          n277 = Array To Cluster(array=w458) -> (cluster=w466:T10)
                          n278 = Unbundle By Name(w467) -> ("hash"=w463:i64)
                          n279 = Multiply(x=w442, y=1000000.0) -> (x*y=w440:dbl)
                          n280 = Unbundle(w466) -> ("output[0]"=w468:dbl, "output[2]"=w457:dbl, "output[3]"=w456:dbl, "output[4]"=w455:dbl, "output[6]"=w454:dbl, "output[7]"=w452:dbl, "output[8]"=w450:dbl, "output[9]"=w448:dbl, "output[12]"=w447:dbl, "output[13]"=w446:dbl, "output[14]"=w445:dbl)  [unwired: 4 out]
                          n281 = call "hash.vi"("input"=w463) -> ("output"=w462:i64)  [unwired: 10 in]
                          n282 = To Quad Integer(1:w440) -> (0:w439:i64)
                          n283 = To Long Integer(number=w454) -> (32bit integer=w453:i32)
                          n284 = To Long Integer(number=w452) -> (32bit integer=w451:i32)
                          n285 = To Long Integer(number=w450) -> (32bit integer=w449:i32)
                          n286 = local read "map"() -> (w444:i32)
                          n287 = Bundle(cluster=w467, "hash"=w462, "sys time"=w439, "time"=w468, "x"=w457, "y"=w456, "h"=w455, "numSV"=w453, "postype"=w451, "lag"=w449, "hordev"=w448, "lat"=w447, "lon"=w446, "hgt"=w445, "map_idx"=w444) -> (w464:T6)
                          n288 = Flatten To String(anything=w464, prepend array or string size? (T)=FALSE) -> (data string=w460:string)  [unwired: 2 in, 2 out]
                          n289 = global read "G_rio.vi" "LCM"() -> (w459:T4)
                          n290 = call "LCM_send.vi"("DATA"=w460, "ID"="GGA_2", "LCM"=w459) -> ()  [unwired: 6 in, 3 out]
                        }
                      }
                    }
                    frame 2 {
                      n291 = global write "G_rio.vi" "gps_vel 2"(w474) -> ()
                      n292 = Index Array(array=w474, index=1) -> (element=w471:dbl)
                      n293 = Not Equal To 0?(x=w471) -> (x != 0?=w470:bool)
                      n294 = local read "LCM"() -> (w472:bool)
                      n295 = And(x=w470, y=w472) -> (x .and. y?=w469:bool)
                      n296 = case shown="True" w469 {
                        tunnel: w474 -> [_ w485]
                        frame False {
                        }
                        frame True {
                          n297 = Get Date/Time In Seconds() -> (seconds since 1Jan1904=w479:timestamp)
                          n298 = To Double Precision Float(number=w479) -> (double precision float=w478:dbl)
                          n299 = global read "G_rio.vi" "LCM_RMC_T"() -> (w486:T8)
                          n300 = Unbundle By Name(w486) -> ("hash"=w490:i64)
                          n301 = Multiply(x=w478, y=1000000.0) -> (x*y=w476:dbl)
                          n302 = Array To Cluster(array=w485) -> (cluster=w487:T11)
                          n303 = call "hash.vi"("input"=w490) -> ("output"=w491:i64)  [unwired: 10 in]
                          n304 = To Quad Integer(1:w476) -> (0:w475:i64)
                          n305 = Unbundle(w487) -> ("output[0]"=w484:dbl, "output[2]"=w483:dbl, "output[4]"=w482:dbl, "output[5]"=w481:dbl, "output[6]"=w480:dbl)  [unwired: 2 out]
                          n306 = Bundle(cluster=w486, "hash"=w491, "sys time"=w475, "time"=w484, "speed"=w483, "heading"=w482, "lat"=w481, "lon"=w480) -> (w489:T8)
                          n307 = Flatten To String(anything=w489, prepend array or string size? (T)=FALSE) -> (data string=w493:string)  [unwired: 2 in, 2 out]
                          n308 = global read "G_rio.vi" "LCM"() -> (w494:T4)
                          n309 = call "LCM_send.vi"("DATA"=w493, "ID"="RMC_2", "LCM"=w494) -> ()  [unwired: 6 in, 3 out]
                        }
                      }
                    }
                  }
                }
                n310 = for {
                  N: 5 -> [_]
                  stop <- w355 stop-if-true
                  n311 = local read "gps1"() -> (w354:refnum<visa-resource-name>)
                  n312 = VISA Read(VISA resource name=w354, byte count=u32 100) -> (read buffer=w358:string, error out=w356:errorcluster)  [unwired: 1 in, 2 out]
                  n313 = local read "ecef ref"() -> (w359:dbl[])
                  n314 = Unbundle By Name(w356) -> ("status"=w355:bool)
                  n315 = call "nmea.vi"("ecef ref"=w359, "NMEA"=w358) -> ("output"=w361:dbl[], "type"=w360:u32)  [unwired: 8 in]
                  n316 = case shown="2" w360 {
                    tunnel: w361 -> [_ w363 w398]
                    frame 0, Default {
                    }
                    frame 1 {
                      n317 = global write "G_rio.vi" "gps_pos 1"(w363) -> ()
                      n318 = Index Array(array=w363, index=1) -> (element=w366:dbl)
                      n319 = Not Equal To 0?(x=w366) -> (x != 0?=w367:bool)
                      n320 = local read "LCM"() -> (w365:bool)
                      n321 = And(x=w367, y=w365) -> (x .and. y?=w362:bool)
                      n322 = case shown="True" w362 {
                        tunnel: w363 -> [_ w387]
                        frame False {
                        }
                        frame True {
                          n323 = Get Date/Time In Seconds() -> (seconds since 1Jan1904=w372:timestamp)
                          n324 = To Double Precision Float(number=w372) -> (double precision float=w371:dbl)
                          n325 = global read "G_rio.vi" "LCM_GGA_T"() -> (w396:T6)
                          n326 = Array To Cluster(array=w387) -> (cluster=w395:T10)
                          n327 = Unbundle By Name(w396) -> ("hash"=w392:i64)
                          n328 = Multiply(x=w371, y=1000000.0) -> (x*y=w369:dbl)
                          n329 = Unbundle(w395) -> ("output[0]"=w397:dbl, "output[2]"=w386:dbl, "output[3]"=w385:dbl, "output[4]"=w384:dbl, "output[6]"=w383:dbl, "output[7]"=w381:dbl, "output[8]"=w379:dbl, "output[9]"=w377:dbl, "output[12]"=w376:dbl, "output[13]"=w375:dbl, "output[14]"=w374:dbl)  [unwired: 4 out]
                          n330 = call "hash.vi"("input"=w392) -> ("output"=w391:i64)  [unwired: 10 in]
                          n331 = To Quad Integer(1:w369) -> (0:w368:i64)
                          n332 = To Long Integer(number=w383) -> (32bit integer=w382:i32)
                          n333 = To Long Integer(number=w381) -> (32bit integer=w380:i32)
                          n334 = To Long Integer(number=w379) -> (32bit integer=w378:i32)
                          n335 = local read "map"() -> (w373:i32)
                          n336 = Bundle(cluster=w396, "hash"=w391, "sys time"=w368, "time"=w397, "x"=w386, "y"=w385, "h"=w384, "numSV"=w382, "postype"=w380, "lag"=w378, "hordev"=w377, "lat"=w376, "lon"=w375, "hgt"=w374, "map_idx"=w373) -> (w393:T6)
                          n337 = Flatten To String(anything=w393, prepend array or string size? (T)=FALSE) -> (data string=w389:string)  [unwired: 2 in, 2 out]
                          n338 = global read "G_rio.vi" "LCM"() -> (w388:T4)
                          n339 = call "LCM_send.vi"("DATA"=w389, "ID"="GGA_1", "LCM"=w388) -> ()  [unwired: 6 in, 3 out]
                        }
                      }
                    }
                    frame 2 {
                      n340 = flat-sequence {
                        tunnel: w398 -> [w400]
                        frame #0 {
                          n341 = Index Array(array=w400, index=1) -> (element=w403:dbl)
                          n342 = Not Equal To 0?(x=w403) -> (x != 0?=w404:bool)
                          n343 = local read "LCM"() -> (w402:bool)
                          n344 = And(x=w404, y=w402) -> (x .and. y?=w399:bool)
                          n345 = case shown="True" w399 {
                            tunnel: w400 -> [_ w423]
                            frame False {
                            }
                            frame True {
                              n346 = Get Date/Time In Seconds() -> (seconds since 1Jan1904=w409:timestamp)
                              n347 = To Double Precision Float(number=w409) -> (double precision float=w408:dbl)
                              n348 = global read "G_rio.vi" "LCM_RMC_T"() -> (w424:T8)
                              n349 = Unbundle By Name(w424) -> ("hash"=w420:i64)
                              n350 = Multiply(x=w408, y=1000000.0) -> (x*y=w406:dbl)
                              n351 = Array To Cluster(array=w423) -> (cluster=w422:T11)
                              n352 = call "hash.vi"("input"=w420) -> ("output"=w419:i64)  [unwired: 10 in]
                              n353 = To Quad Integer(1:w406) -> (0:w405:i64)
                              n354 = Unbundle(w422) -> ("output[0]"=w414:dbl, "output[2]"=w413:dbl, "output[4]"=w412:dbl, "output[5]"=w411:dbl, "output[6]"=w410:dbl)  [unwired: 2 out]
                              n355 = Bundle(cluster=w424, "hash"=w419, "sys time"=w405, "time"=w414, "speed"=w413, "heading"=w412, "lat"=w411, "lon"=w410) -> (w415:T8)
                              n356 = Flatten To String(anything=w415, prepend array or string size? (T)=FALSE) -> (data string=w417:string)  [unwired: 2 in, 2 out]
                              n357 = global read "G_rio.vi" "LCM"() -> (w416:T4)
                              n358 = call "LCM_send.vi"("DATA"=w417, "ID"="RMC_1", "LCM"=w416) -> ()  [unwired: 6 in, 3 out]
                            }
                          }
                        }
                      }
                      n359 = global write "G_rio.vi" "gps_vel 1"(w398) -> ()
                    }
                  }
                }
              }
            }
          }
        }
      }
      n360 = while {
        stop <- FALSE stop-if-true
        n361 = flat-sequence {
          frame #0 {
            n362 = Wait Until Next ms Multiple(millisecond multiple=u32 10) -> (millisecond timer value=w1808:u32)
            n363 = flat-sequence {
              tunnel: w1808 -> [w1811]
              frame #0 {
                n364 = feedback #4(w1811) -> (w1812:u32)
                n365 = feedback-in #4(w1811) -> ()
                n366 = Subtract(x=w1811, y=w1812) -> (x-y=→"CAN_time 10":u32)
              }
            }
          }
          frame #1 {
            n367 = disable-structure shown="Enabled" {
              disable-tunnel: [w1814 w2075 _] -> w1813
              frame Disabled {
                n368 = local read "CAN read"() -> (w1817:refnum<k21>)
                n369 = call-poly <vilib>:"XNET Read.vi"("session in"=w1817) -> ("data"=w1816:T2[])  [unwired: 3 in, 11 out]
                n370 = for {
                  tunnel: w1816 -> [w1818] mode=indexing
                  n371 = Unbundle By Name(w1818) -> ("timestamp"=w1819:timestamp, "identifier"=w1821:u32, "payload"=w1820:u8[])
                  n372 = case shown="4F0" w1821 {
                    selector: w1821 -> [w1825 _ _ _ _ _ _ _ _]
                    tunnel: w1820 -> [_ w1829 w1903 w1938 w1957 w1998 w2029 w2061 w2068]
                    tunnel: w1819 -> [_ _ w1898 _ _ _ _ _ _]
                    tunnel: w1818 -> [_ w1827 _ _ _ _ _ _ _]
                    frame 0, Default {
                      n373 = local read item#-1() -> (w1826)
                      n374 = Build Array (concatenate)(w1825, w1826) -> (w1824:u32[])
                      n375 = Array Subset(array=w1824, length=20) -> (w1822:u32[])  [unwired: 1 in]
                      n376 = local write item#-1(w1822) -> ()
                    }
                    frame 356 {
                      n377 = case shown="False" "steer2" {
                        tunnel: w1829 -> [_ w1857]
                        tunnel: w1827 -> [_ w1834]
                        frame False {
                        }
                        frame True {
                          w1848 = u16 28672  # 5, 3
                          n378 = Array Subset(array=w1857, index=2, length=5) -> (w1861:u8[])
                          n379 = Index Array(array=w1861, index=4) -> (element=w1864:u8)
                          n380 = Increment(x=w1864) -> (x+1=w1862:u8)
                          n381 = And(x=w1862, y=u8 15) -> (x .and. y?=w1860:u8)
                          n382 = Multiply(x="Ref steer manual 2", y=100.0) -> (x*y=w1853:dbl)
                          n383 = Add(x=w1853, y=2048.0) -> (x+y=w1833:dbl)
                          n384 = Replace Array Subset(array=w1861, new element=w1860, index=4) -> (w1849:u8[])
                          n385 = In Range and Coerce(upper limit=4094.0, x=w1833, lower limit=0.0) -> (coerced(x)=w1830:dbl)  [unwired: 1 out]
                          n386 = To Unsigned Word Integer(number=w1830) -> (unsigned 16bit integer=w1850:u16)
                          n387 = And(x=w1850, y=u16 4095) -> (x .and. y?=w1847:u16)
                          n388 = Add(x=w1848, y=w1847) -> (x+y=w1846:u16)
                          n389 = Split Number(x=w1846) -> (hi(x)=w1844:u8, lo(x)=w1845:u8)
                          n390 = Build Array (concatenate)(w1845, w1844, w1849) -> (w1843:u8[])
                          n391 = for {
                            tunnel: w1843 -> [w1866] mode=indexing
                            shift-right: [w1868] -> w1840
                            shift-left: u8 0 -> [w1867]
                            tunnel: [w1866] -> w1841 mode=indexing
                            n392 = Exclusive Or(1:w1867, 2:w1866) -> (0:w1868:u8)
                          }
                          n393 = Build Array (concatenate)(w1841, w1840) -> (w1837:u8[])
                          n394 = Bundle By Name(cluster=w1834, "payload"=w1837) -> (w1838:T2)
                          n395 = local read "CAN write"() -> (w1835:refnum<k21>)
                          n396 = Build Array(w1838) -> (w1839:T2[])
                          n397 = call-poly <vilib>:"XNET Write.vi"("session in"=w1835, "data"=w1839, "timeout (10)"=0.01) -> ()  [unwired: 11 in, 2 out]
                        }
                      }
                    }
                    frame 544 {
                      w1872 = u16 8191
                      w1879 = u16 2047
                      n398 = global write "G_rio.vi" "timestamp"(w1898) -> ()
                      n399 = Index Array(array=w1903, index #1=5 ("index"), index #2=4 ("index"), index #3=1 ("index"), index #4=0 ("index"), index #5=7 ("index"), index #6=6 ("index")) -> (element #1=w1895:u8, element #2=w1894:u8, element #3=w1893:u8, element #4=w1892:u8, element #5=w1891:u8, element #6=w1890:u8)
                      n400 = Join Numbers(hi=w1893, lo=w1892) -> ((hi.lo)=w1880:u16)
                      n401 = Join Numbers(hi=w1891, lo=w1890) -> ((hi.lo)=w1871:u16)
                      n402 = And(x=w1895, y=u8 15) -> (x .and. y?=w1888:u8)
                      n403 = Logical Shift(y=i16 -6, x=w1893) -> (x << y=w1882:u8)
                      n404 = Logical Shift(y=i16 -6, x=w1891) -> (x << y=w1875:u8)
                      n405 = Join Numbers(hi=w1888, lo=w1894) -> ((hi.lo)=w1885:u16)
                      n406 = Equal To 0?(x=w1882) -> (x = 0?=w1883:bool)
                      n407 = And(x=w1879, y=w1880) -> (x .and. y?=w1878:u16)
                      n408 = And(x=w1872, y=w1871) -> (x .and. y?=w1870:u16)
                      n409 = Not Equal?(x=w1879, y=w1878) -> (x != y?=w1884:bool)
                      n410 = Not Equal?(x=w1872, y=w1870) -> (x != y?=w1873:bool)
                      n411 = Equal To 0?(x=w1875) -> (x = 0?=w1874:bool)
                      n412 = Not Equal?(x=u16 4095, y=w1885) -> (x != y?=w1886:bool)
                      n413 = case shown="True" w1886 {
                        tunnel: w1885 -> [_ w1926]
                        frame False {
                        }
                        frame True {
                          n414 = global write "G_rio.vi" "mcp"(w1926) -> ()
                          n415 = To Double Precision Float(number=w1926) -> (double precision float=w1928:dbl)
                          n416 = Greater?(x=w1926, y=u16 10) -> (0:w1925:bool)
                          n417 = global write "G_rio.vi" "brake_act_can"(w1925) -> ()
                          n418 = Multiply(x=w1928, y=10.0) -> (x*y=w1923:dbl)
                          n419 = Square Root(x=w1923) -> (sqrt(x)=w1922:dbl)
                          n420 = global write "G_rio.vi" "Brake Encoder mcp"(w1922) -> ()
                        }
                      }
                      n421 = And(x=w1883, y=w1884) -> (x .and. y?=w1877:bool)
                      n422 = And(x=w1874, y=w1873) -> (x .and. y?=w1869:bool)
                      n423 = case shown="True" w1877 {
                        tunnel: w1878 -> [_ w1921]
                        frame False {
                        }
                        frame True {
                          n424 = To Double Precision Float(number=w1921) -> (double precision float=w1920:dbl)
                          n425 = Multiply(x=w1920, y=0.01) -> (x*y=w1918:dbl)
                          n426 = Subtract(x=w1918, y=10.23) -> (x-y=w1916:dbl)
                          n427 = global write "G_rio.vi" "lat_accel"(w1916) -> ()
                        }
                      }
                      n428 = case shown="True" w1869 {
                        tunnel: w1870 -> [_ w1915]
                        frame False {
                        }
                        frame True {
                          n429 = To Double Precision Float(number=w1915) -> (double precision float=w1914:dbl)
                          n430 = Multiply(x=w1914, y=0.01) -> (x*y=w1912:dbl)
                          n431 = Subtract(x=w1912, y=40.95) -> (x-y=w1905:dbl)
                          n432 = Add(x=w1905, y=-0.034) -> (x+y=w1904:dbl)
                          n433 = Multiply(x=w1904, y=1.045) -> (x*y=w1908:dbl)
                          n434 = Add(x=w1908, y=0.0) -> (x+y=w1907:dbl)
                          n435 = global write "G_rio.vi" "yaw_rate"(w1907) -> ()
                        }
                      }
                    }
                    frame 809 {
                      # "10ms"
                      n436 = Index Array(array=w1938, index #1=5 ("index"), index #2=6 ("index"), index #3=4 ("index")) -> (element #1=w1935:u8, element #2=w1932:u8)  [unwired: 1 out]
                      n437 = Not Equal?(x=w1935, y=u8 255 ("x")) -> (x != y?=w1931:bool)
                      n438 = Not Equal?(x=w1932, y=u8 255 ("x")) -> (x != y?=w1930:bool)
                      n439 = case shown="True" w1931 {
                        tunnel: w1935 -> [_ w1950]
                        frame False {
                        }
                        frame True {
                          n440 = Subtract(x=w1950, y=u8 32) -> (x-y=w1948:u8)
                          n441 = To Double Precision Float(number=w1948) -> (double precision float=w1947:dbl)
                          n442 = Multiply(x=w1947, y=100.0) -> (x*y=w1945:dbl)
                          n443 = Divide(x=w1945, y=213.0) -> (x/y=w1943:dbl)
                          n444 = global write "G_rio.vi" "tps"(w1943) -> ()
                        }
                      }
                      n445 = case shown="True" w1930 {
                        tunnel: w1932 -> [_ w1942]
                        frame False {
                        }
                        frame True {
                          n446 = To Double Precision Float(number=w1942) -> (double precision float=w1941:dbl)
                          n447 = Multiply(x=w1941, y=0.3906) -> (x*y=w1940:dbl)
                          n448 = global write "G_rio.vi" "accel pedal value"(w1940) -> ()
                        }
                      }
                    }
                    frame 914 {
                      # "20ms"
                      n449 = Index Array(array=w1957, index #1=7 ("index"), index #2=2 ("index"), index #3=1 ("index"), index #4=4 ("index"), index #5=3 ("index")) -> (element #1=w1951:u8, element #2=w1963:u8, element #3=w1962:u8, element #4=w1959:u8, element #5=w1958:u8)
                      n450 = Array Subset(array=w1957, index=0, length=7) -> (w1954:u8[])
                      n451 = Add Array Elements(numeric array=w1954) -> (sum=w1952:u8)
                      n452 = Equal?(x=w1952, y=w1951) -> (x = y?=w1953:bool)
                      n453 = case shown="True" w1953 {
                        tunnel: w1963 -> [_ w1977]
                        tunnel: w1962 -> [_ w1976]
                        tunnel: w1959 -> [_ w1973]
                        tunnel: w1958 -> [_ w1972]
                        frame False {
                        }
                        frame True {
                          w1968 = u16 4095 ("y")
                          n454 = Join Numbers(hi=w1977, lo=w1976) -> ((hi.lo)=w1969:u16)
                          n455 = Join Numbers(hi=w1973, lo=w1972) -> ((hi.lo)=w1974:u16)
                          n456 = And(x=w1968, y=w1969) -> (x .and. y?=w1967:u16)
                          n457 = Not Equal?(x=w1974, y=u16 32767 ("x")) -> (x != y?=w1970:bool)
                          n458 = Not Equal?(x=w1968, y=w1967) -> (x != y?=w1971:bool)
                          n459 = case shown="True" w1971 {
                            tunnel: w1967 -> [_ w1989]
                            frame False {
                            }
                            frame True {
                              n460 = To Double Precision Float(number=w1989) -> (double precision float=w1988:dbl)
                              n461 = Subtract(x=w1988, y=2048.0) -> (x-y=w1987:dbl)
                              n462 = Multiply(x=w1987, y=0.01) -> (x*y=w1990:dbl)
                              n463 = global write "G_rio.vi" "mdps torque"(w1990) -> ()
                            }
                          }
                          n464 = case shown="True" w1970 {
                            tunnel: w1974 -> [_ w1984]
                            frame False {
                            }
                            frame True {
                              n465 = To Double Precision Float(number=w1984) -> (double precision float=w1981:dbl)
                              n466 = Subtract(x=w1981, y=65536.0) -> (x-y=w1982:dbl)
                              n467 = Greater?(x=w1981, y=32767.0 ("x")) -> (0:w1985:bool)
                              n468 = Select(t=w1982, s=w1985, f=w1981) -> (s? t:f=w1980:dbl)
                              n469 = Multiply(x=w1980, y=0.1) -> (x*y=w1978:dbl)
                              n470 = global write "G_rio.vi" "mdps str_ang"(w1978) -> ()
                            }
                          }
                        }
                      }
                    }
                    frame 1087 {
                      w1995 = u8 15 ("y")
                      # "10ms"
                      n471 = Index Array(array=w1998, index=1) -> (element=w1996:u8)
                      n472 = And(x=w1996, y=w1995) -> (x .and. y?=w1994:u8)
                      n473 = Not Equal?(x=w1994, y=w1995) -> (x != y?=w1993:bool)
                      n474 = case shown="True" w1993 {
                        tunnel: w1994 -> [_ w1999]
                        frame False {
                        }
                        frame True {
                          n475 = global write "G_rio.vi" "gear selector disp"(w1999) -> ()
                        }
                      }
                    }
                    frame 1200 {
                      w2003 = u16 16383 ("x")
                      w2016 = u16 16383 ("x")
                      # "20ms"
                      n476 = Index Array(array=w2029, index #1=1 ("index"), index #2=0 ("index"), index #3=3 ("index"), index #4=2 ("index"), index #5=5 ("index"), index #6=4 ("index"), index #7=7 ("index"), index #8=6 ("index")) -> (element #1=w2008:u8, element #2=w2007:u8, element #3=w2006:u8, element #4=w2005:u8, element #5=w2026:u8, element #6=w2025:u8, element #7=w2021:u8, element #8=w2020:u8)
                      n477 = Join Numbers(hi=w2008, lo=w2007) -> ((hi.lo)=w2004:u16)
                      n478 = Join Numbers(hi=w2006, lo=w2005) -> ((hi.lo)=w2002:u16)
                      n479 = Join Numbers(hi=w2026, lo=w2025) -> ((hi.lo)=w2024:u16)
                      n480 = Join Numbers(hi=w2021, lo=w2020) -> ((hi.lo)=w2017:u16)
                      n481 = And(x=w2004, y=w2003) -> (x .and. y?=w2001:u16)
                      n482 = And(x=w2003, y=w2002) -> (x .and. y?=w2000:u16)
                      n483 = And(x=w2024, y=w2016) -> (x .and. y?=w2015:u16)
                      n484 = And(x=w2016, y=w2017) -> (x .and. y?=w2014:u16)
                      n485 = Not Equal?(x=w2015, y=w2016) -> (x != y?=w2019:bool)
                      n486 = Not Equal?(x=w2016, y=w2014) -> (x != y?=w2018:bool)
                      n487 = And(x=w2019, y=w2018) -> (x .and. y?=w2013:bool)
                      n488 = case shown="True" w2013 {
                        tunnel: w2015 -> [_ w2048]
                        tunnel: w2014 -> [_ w2047]
                        tunnel: w2001 -> [_ w2040]
                        tunnel: w2000 -> [_ w2039]
                        frame False {
                        }
                        frame True {
                          w2035 = 0.03125 ("y")
                          w2046 = 0.03125 ("y")
                          n489 = To Double Precision Float(number=w2040) -> (double precision float=w2037:dbl)
                          n490 = To Double Precision Float(number=w2039) -> (double precision float=w2034:dbl)
                          n491 = To Double Precision Float(number=w2048) -> (double precision float=w2038:dbl)
                          n492 = To Double Precision Float(number=w2047) -> (double precision float=w2031:dbl)
                          n493 = Multiply(x=w2037, y=w2035) -> (x*y=w2036:dbl)
                          n494 = Multiply(x=w2035, y=w2034) -> (x*y=w2033:dbl)
                          n495 = Multiply(x=w2038, y=w2046) -> (x*y=w2032:dbl)
                          n496 = Multiply(x=w2046, y=w2031) -> (x*y=w2030:dbl)
                          n497 = global write "G_rio.vi" "WHL_SPD_FL"(w2036) -> ()
                          n498 = global write "G_rio.vi" "WHL_SPD_FR"(w2033) -> ()
                          n499 = global write "G_rio.vi" "WHL_SPD_RL"(w2032) -> ()
                          n500 = global write "G_rio.vi" "WHL_SPD_RR"(w2030) -> ()
                          n501 = Add(x=w2032, y=w2030) -> (x+y=w2045:dbl)
                          n502 = Multiply(x=w2045, y=0.5) -> (x*y=w2042:dbl)
                          n503 = Multiply(x=w2042, y=1.028) -> (x*y=w2041:dbl)
                          n504 = global write "G_rio.vi" "vs_esc"(w2041) -> ()
                        }
                      }
                    }
                    frame 1264 {
                      # "20 ms"
                      n505 = Index Array(array=w2061, index #1=7 ("index"), index #2=6 ("index"), index #3=5 ("index")) -> (element #1=w2055:u8, element #2=w2057:u8, element #3=w2056:u8)
                      n506 = Join Numbers(hi=w2057, lo=w2056) -> ((hi.lo)=w2052:u16)
                      n507 = Join Numbers(hi=u8 0, lo=w2055) -> ((hi.lo)=w2053:u16)
                      n508 = Join Numbers(hi=w2053, lo=w2052) -> ((hi.lo)=w2050:u32)
                      n509 = Not Equal?(x=u32 16777215, y=w2050) -> (x != y?=w2049:bool)
                      n510 = case shown="True" w2049 {
                        tunnel: w2050 -> [_ w2063]
                        frame False {
                        }
                        frame True {
                          n511 = To Double Precision Float(number=w2063) -> (double precision float=w2062:dbl)
                          n512 = global write "G_rio.vi" "odometer"(w2062) -> ()
                        }
                      }
                    }
                    frame 1349 {
                      # "10 ms"
                      n513 = Index Array(array=w2068, index=3) -> (element=w2066:u8)
                      n514 = Not Equal?(x=w2066, y=u8 255 ("x")) -> (x != y?=w2064:bool)
                      n515 = case shown="True" w2064 {
                        tunnel: w2066 -> [_ w2074]
                        frame False {
                        }
                        frame True {
                          n516 = To Double Precision Float(number=w2074) -> (double precision float=w2073:dbl)
                          n517 = Multiply(x=26.0, y=w2073) -> (x*y=w2071:dbl)
                          n518 = Divide(x=w2071, y=256.0) -> (x/y=w2069:dbl)
                          n519 = global write "G_rio.vi" "battery voltage"(w2069) -> ()
                        }
                      }
                    }
                  }
                }
                n520 = Empty Array?(array=w1816) -> (empty?=w1815:bool)
                n521 = Not(x=w1815) -> (.not. x?=w1814:bool)
              }
              frame Enabled {
                n522 = for {
                  tunnel: u32[] [356, 544, 809, 914, 1087, 1200, 1264, 1349] -> [w2079] mode=indexing
                  tunnel: [w2078] -> w2076 mode=indexing
                  n523 = case shown="220" w2079 {
                    tunnel: [_ w2080 w2156 w2195 w2254 w2278 w2344 w2376] -> w2078
                    frame 0, Default {
                    }
                    frame 544 {
                      n524 = flat-sequence {
                        tunnel: [w2084] -> w2080
                        tunnel: [w2083] -> w2081
                        frame #0 {
                          n525 = local read "FPGA VI Reference Out"() -> (w2089:refnum<k20>)
                          n526 = xnode "Read/Write Control"("FPGA VI Reference In"=w2089) -> ("can 220"=w2088:u8[])  [unwired: 1 in, 2 out]
                          n527 = Index Array(array=w2088, index #1=0 ("index")) -> (element #1=w2095:u8, element #2=w2094:u8, element #3=w2093:u8, element #4=w2092:u8)  [unwired: 3 in]
                          n528 = Join Numbers(hi=w2095, lo=w2094) -> ((hi.lo)=w2091:u16)
                          n529 = Join Numbers(hi=w2093, lo=w2092) -> ((hi.lo)=w2090:u16)
                          n530 = Join Numbers(hi=w2091, lo=w2090) -> ((hi.lo)=w2082:u32)
                          n531 = Array Subset(array=w2088, index=4) -> (w2083:u8[])  [unwired: 1 in]
                          n532 = global write "G_rio.vi" "time"(w2082) -> ()
                          n533 = feedback #5(u32 0) -> (w2085:u32)
                          n534 = feedback-in #5(w2082) -> ()
                          n535 = Not Equal?(x=w2082, y=w2085) -> (x != y?=w2084:bool)
                        }
                      }
                      n536 = case shown="True" w2080 {
                        tunnel: w2081 -> [_ w2130]
                        frame False {
                        }
                        frame True {
                          w2100 = u16 8191
                          w2107 = u16 2047
                          n537 = Index Array(array=w2130, index #1=5 ("index"), index #2=4 ("index"), index #3=1 ("index"), index #4=0 ("index"), index #5=7 ("index"), index #6=6 ("index")) -> (element #1=w2123:u8, element #2=w2122:u8, element #3=w2121:u8, element #4=w2120:u8, element #5=w2119:u8, element #6=w2118:u8)
                          n538 = Join Numbers(hi=w2121, lo=w2120) -> ((hi.lo)=w2108:u16)
                          n539 = Join Numbers(hi=w2119, lo=w2118) -> ((hi.lo)=w2099:u16)
                          n540 = And(x=w2123, y=u8 15) -> (x .and. y?=w2116:u8)
                          n541 = Logical Shift(y=i16 -6, x=w2121) -> (x << y=w2110:u8)
                          n542 = Logical Shift(y=i16 -6, x=w2119) -> (x << y=w2103:u8)
                          n543 = Equal To 0?(x=w2110) -> (x = 0?=w2111:bool)
                          n544 = Join Numbers(hi=w2116, lo=w2122) -> ((hi.lo)=w2113:u16)
                          n545 = And(x=w2107, y=w2108) -> (x .and. y?=w2106:u16)
                          n546 = And(x=w2100, y=w2099) -> (x .and. y?=w2098:u16)
                          n547 = Not Equal?(x=w2107, y=w2106) -> (x != y?=w2112:bool)
                          n548 = Not Equal?(x=w2100, y=w2098) -> (x != y?=w2101:bool)
                          n549 = Equal To 0?(x=w2103) -> (x = 0?=w2102:bool)
                          n550 = Not Equal?(x=u16 4095, y=w2113) -> (x != y?=w2114:bool)
                          n551 = case shown="True" w2114 {
                            tunnel: w2113 -> [_ w2153]
                            frame False {
                            }
                            frame True {
                              n552 = global write "G_rio.vi" "mcp"(w2153) -> ()
                              n553 = To Double Precision Float(number=w2153) -> (double precision float=w2155:dbl)
                              n554 = Greater?(x=w2153, y=u16 10) -> (0:w2152:bool)
                              n555 = global write "G_rio.vi" "brake_act_can"(w2152) -> ()
                              n556 = Multiply(x=w2155, y=10.0) -> (x*y=w2150:dbl)
                              n557 = Square Root(x=w2150) -> (sqrt(x)=w2149:dbl)
                              n558 = global write "G_rio.vi" "Brake Encoder mcp"(w2149) -> ()
                            }
                          }
                          n559 = And(x=w2111, y=w2112) -> (x .and. y?=w2105:bool)
                          n560 = And(x=w2102, y=w2101) -> (x .and. y?=w2097:bool)
                          n561 = case shown="True" w2105 {
                            tunnel: w2106 -> [_ w2148]
                            frame False {
                            }
                            frame True {
                              n562 = To Double Precision Float(number=w2148) -> (double precision float=w2147:dbl)
                              n563 = Multiply(x=w2147, y=0.01) -> (x*y=w2145:dbl)
                              n564 = Subtract(x=w2145, y=10.23) -> (x-y=w2143:dbl)
                              n565 = global write "G_rio.vi" "lat_accel"(w2143) -> ()
                            }
                          }
                          n566 = case shown="True" w2097 {
                            tunnel: w2098 -> [_ w2142]
                            frame False {
                            }
                            frame True {
                              n567 = To Double Precision Float(number=w2142) -> (double precision float=w2141:dbl)
                              n568 = Multiply(x=w2141, y=0.01) -> (x*y=w2139:dbl)
                              n569 = Subtract(x=w2139, y=40.95) -> (x-y=w2132:dbl)
                              n570 = Add(x=w2132, y=-0.034) -> (x+y=w2131:dbl)
                              n571 = Multiply(x=w2131, y=1.045) -> (x*y=w2135:dbl)
                              n572 = Add(x=w2135, y=0.0) -> (x+y=w2134:dbl)
                              n573 = global write "G_rio.vi" "yaw_rate"(w2134) -> ()
                            }
                          }
                        }
                      }
                    }
                    frame 809 {
                      n574 = flat-sequence {
                        tunnel: [w2159] -> w2156
                        tunnel: [w2158] -> w2157
                        frame #0 {
                          n575 = local read "FPGA VI Reference Out"() -> (w2165:refnum<k20>)
                          n576 = xnode "Read/Write Control"("FPGA VI Reference In"=w2165) -> ("can 329"=w2164:u8[])  [unwired: 1 in, 2 out]
                          n577 = Index Array(array=w2164, index #1=0 ("index")) -> (element #1=w2171:u8, element #2=w2170:u8, element #3=w2169:u8, element #4=w2168:u8)  [unwired: 3 in]
                          n578 = Join Numbers(hi=w2171, lo=w2170) -> ((hi.lo)=w2167:u16)
                          n579 = Join Numbers(hi=w2169, lo=w2168) -> ((hi.lo)=w2166:u16)
                          n580 = Join Numbers(hi=w2167, lo=w2166) -> ((hi.lo)=w2160:u32)
                          n581 = Array Subset(array=w2164, index=4) -> (w2158:u8[])  [unwired: 1 in]
                          n582 = feedback #6(u32 0) -> (w2161:u32)
                          n583 = feedback-in #6(w2160) -> ()
                          n584 = Not Equal?(x=w2160, y=w2161) -> (x != y?=w2159:bool)
                        }
                      }
                      n585 = case shown="True" w2156 {
                        tunnel: w2157 -> [_ w2182]
                        frame False {
                        }
                        frame True {
                          # "10ms"
                          n586 = Index Array(array=w2182, index #1=5 ("index"), index #2=6 ("index"), index #3=4 ("index")) -> (element #1=w2179:u8, element #2=w2176:u8)  [unwired: 1 out]
                          n587 = Not Equal?(x=w2179, y=u8 255 ("x")) -> (x != y?=w2175:bool)
                          n588 = Not Equal?(x=w2176, y=u8 255 ("x")) -> (x != y?=w2174:bool)
                          n589 = case shown="True" w2175 {
                            tunnel: w2179 -> [_ w2194]
                            frame False {
                            }
                            frame True {
                              n590 = Subtract(x=w2194, y=u8 32) -> (x-y=w2192:u8)
                              n591 = To Double Precision Float(number=w2192) -> (double precision float=w2191:dbl)
                              n592 = Multiply(x=w2191, y=100.0) -> (x*y=w2189:dbl)
                              n593 = Divide(x=w2189, y=213.0) -> (x/y=w2187:dbl)
                              n594 = global write "G_rio.vi" "tps"(w2187) -> ()
                            }
                          }
                          n595 = case shown="True" w2174 {
                            tunnel: w2176 -> [_ w2186]
                            frame False {
                            }
                            frame True {
                              n596 = To Double Precision Float(number=w2186) -> (double precision float=w2185:dbl)
                              n597 = Multiply(x=w2185, y=0.3906) -> (x*y=w2184:dbl)
                              n598 = global write "G_rio.vi" "accel pedal value"(w2184) -> ()
                            }
                          }
                        }
                      }
                    }
                    frame 914 {
                      n599 = flat-sequence {
                        tunnel: [w2198] -> w2195
                        tunnel: [w2197] -> w2196
                        frame #0 {
                          n600 = local read "FPGA VI Reference Out"() -> (w2204:refnum<k20>)
                          n601 = xnode "Read/Write Control"("FPGA VI Reference In"=w2204) -> ("can 392"=w2203:u8[])  [unwired: 1 in, 2 out]
                          n602 = Index Array(array=w2203, index #1=0 ("index")) -> (element #1=w2210:u8, element #2=w2209:u8, element #3=w2208:u8, element #4=w2207:u8)  [unwired: 3 in]
                          n603 = Join Numbers(hi=w2210, lo=w2209) -> ((hi.lo)=w2206:u16)
                          n604 = Join Numbers(hi=w2208, lo=w2207) -> ((hi.lo)=w2205:u16)
                          n605 = Join Numbers(hi=w2206, lo=w2205) -> ((hi.lo)=w2199:u32)
                          n606 = Array Subset(array=w2203, index=4) -> (w2197:u8[])  [unwired: 1 in]
                          n607 = feedback #7(u32 0) -> (w2200:u32)
                          n608 = feedback-in #7(w2199) -> ()
                          n609 = Not Equal?(x=w2199, y=w2200) -> (x != y?=w2198:bool)
                        }
                      }
                      n610 = case shown="True" w2195 {
                        tunnel: w2196 -> [_ w2218]
                        frame False {
                        }
                        frame True {
                          # "20ms"
                          n611 = Array Subset(array=w2218, index=0, length=7) -> (w2215:u8[])
                          n612 = Index Array(array=w2218, index #1=7 ("index"), index #2=2 ("index"), index #3=1 ("index"), index #4=4 ("index"), index #5=3 ("index")) -> (element #1=w2212:u8, element #2=w2224:u8, element #3=w2223:u8, element #4=w2220:u8, element #5=w2219:u8)
                          n613 = Add Array Elements(numeric array=w2215) -> (sum=w2213:u8)
                          n614 = Equal?(x=w2213, y=w2212) -> (x = y?=w2214:bool)
                          n615 = case shown="True" w2214 {
                            tunnel: w2224 -> [_ w2238]
                            tunnel: w2223 -> [_ w2237]
                            tunnel: w2220 -> [_ w2234]
                            tunnel: w2219 -> [_ w2233]
                            frame False {
                            }
                            frame True {
                              w2229 = u16 4095 ("y")
                              n616 = Join Numbers(hi=w2238, lo=w2237) -> ((hi.lo)=w2230:u16)
                              n617 = Join Numbers(hi=w2234, lo=w2233) -> ((hi.lo)=w2235:u16)
                              n618 = And(x=w2229, y=w2230) -> (x .and. y?=w2228:u16)
                              n619 = Not Equal?(x=w2235, y=u16 32767 ("x")) -> (x != y?=w2231:bool)
                              n620 = Not Equal?(x=w2229, y=w2228) -> (x != y?=w2232:bool)
                              n621 = case shown="True" w2232 {
                                tunnel: w2228 -> [_ w2250]
                                frame False {
                                }
                                frame True {
                                n622 = To Double Precision Float(number=w2250) -> (double precision float=w2249:dbl)
                                n623 = Subtract(x=w2249, y=2048.0) -> (x-y=w2248:dbl)
                                n624 = Multiply(x=w2248, y=0.01) -> (x*y=w2251:dbl)
                                n625 = global write "G_rio.vi" "mdps torque"(w2251) -> ()
                                }
                              }
                              n626 = case shown="True" w2231 {
                                tunnel: w2235 -> [_ w2245]
                                frame False {
                                }
                                frame True {
                                n627 = To Double Precision Float(number=w2245) -> (double precision float=w2242:dbl)
                                n628 = Subtract(x=w2242, y=65536.0) -> (x-y=w2243:dbl)
                                n629 = Greater?(x=w2242, y=32767.0 ("x")) -> (0:w2246:bool)
                                n630 = Select(t=w2243, s=w2246, f=w2242) -> (s? t:f=w2241:dbl)
                                n631 = Multiply(x=w2241, y=0.1) -> (x*y=w2239:dbl)
                                n632 = global write "G_rio.vi" "mdps str_ang"(w2239) -> ()
                                }
                              }
                            }
                          }
                        }
                      }
                    }
                    frame 1087 {
                      n633 = flat-sequence {
                        tunnel: [w2257] -> w2254
                        tunnel: [w2256] -> w2255
                        frame #0 {
                          n634 = local read "FPGA VI Reference Out"() -> (w2263:refnum<k20>)
                          n635 = xnode "Read/Write Control"("FPGA VI Reference In"=w2263) -> ("can 43F"=w2262:u8[])  [unwired: 1 in, 2 out]
                          n636 = Index Array(array=w2262, index #1=0 ("index")) -> (element #1=w2269:u8, element #2=w2268:u8, element #3=w2267:u8, element #4=w2266:u8)  [unwired: 3 in]
                          n637 = Join Numbers(hi=w2269, lo=w2268) -> ((hi.lo)=w2265:u16)
                          n638 = Join Numbers(hi=w2267, lo=w2266) -> ((hi.lo)=w2264:u16)
                          n639 = Join Numbers(hi=w2265, lo=w2264) -> ((hi.lo)=w2258:u32)
                          n640 = Array Subset(array=w2262, index=4) -> (w2256:u8[])  [unwired: 1 in]
                          n641 = feedback #8(u32 0) -> (w2259:u32)
                          n642 = feedback-in #8(w2258) -> ()
                          n643 = Not Equal?(x=w2258, y=w2259) -> (x != y?=w2257:bool)
                        }
                      }
                      n644 = case shown="True" w2254 {
                        tunnel: w2255 -> [_ w2276]
                        frame False {
                        }
                        frame True {
                          w2273 = u8 15 ("y")
                          # "10ms"
                          n645 = Index Array(array=w2276, index=1) -> (element=w2274:u8)
                          n646 = And(x=w2274, y=w2273) -> (x .and. y?=w2272:u8)
                          n647 = Not Equal?(x=w2272, y=w2273) -> (x != y?=w2271:bool)
                          n648 = case shown="True" w2271 {
                            tunnel: w2272 -> [_ w2277]
                            frame False {
                            }
                            frame True {
                              n649 = global write "G_rio.vi" "gear selector disp"(w2277) -> ()
                            }
                          }
                        }
                      }
                    }
                    frame 1200 {
                      n650 = flat-sequence {
                        tunnel: [w2281] -> w2278
                        tunnel: [w2280] -> w2279
                        frame #0 {
                          n651 = local read "FPGA VI Reference Out"() -> (w2287:refnum<k20>)
                          n652 = xnode "Read/Write Control"("FPGA VI Reference In"=w2287) -> ("can 4B0"=w2286:u8[])  [unwired: 1 in, 2 out]
                          n653 = Index Array(array=w2286, index #1=0 ("index")) -> (element #1=w2293:u8, element #2=w2292:u8, element #3=w2291:u8, element #4=w2290:u8)  [unwired: 3 in]
                          n654 = Join Numbers(hi=w2293, lo=w2292) -> ((hi.lo)=w2289:u16)
                          n655 = Join Numbers(hi=w2291, lo=w2290) -> ((hi.lo)=w2288:u16)
                          n656 = Join Numbers(hi=w2289, lo=w2288) -> ((hi.lo)=w2282:u32)
                          n657 = Array Subset(array=w2286, index=4) -> (w2280:u8[])  [unwired: 1 in]
                          n658 = feedback #9(u32 0) -> (w2283:u32)
                          n659 = feedback-in #9(w2282) -> ()
                          n660 = Not Equal?(x=w2282, y=w2283) -> (x != y?=w2281:bool)
                        }
                      }
                      n661 = case shown="True" w2278 {
                        tunnel: w2279 -> [_ w2324]
                        frame False {
                        }
                        frame True {
                          w2298 = u16 16383 ("x")
                          w2311 = u16 16383 ("x")
                          # "20ms"
                          n662 = Index Array(array=w2324, index #1=1 ("index"), index #2=0 ("index"), index #3=3 ("index"), index #4=2 ("index"), index #5=5 ("index"), index #6=4 ("index"), index #7=7 ("index"), index #8=6 ("index")) -> (element #1=w2303:u8, element #2=w2302:u8, element #3=w2301:u8, element #4=w2300:u8, element #5=w2321:u8, element #6=w2320:u8, element #7=w2316:u8, element #8=w2315:u8)
                          n663 = Join Numbers(hi=w2303, lo=w2302) -> ((hi.lo)=w2299:u16)
                          n664 = Join Numbers(hi=w2301, lo=w2300) -> ((hi.lo)=w2297:u16)
                          n665 = Join Numbers(hi=w2321, lo=w2320) -> ((hi.lo)=w2319:u16)
                          n666 = Join Numbers(hi=w2316, lo=w2315) -> ((hi.lo)=w2312:u16)
                          n667 = And(x=w2299, y=w2298) -> (x .and. y?=w2296:u16)
                          n668 = And(x=w2298, y=w2297) -> (x .and. y?=w2295:u16)
                          n669 = And(x=w2319, y=w2311) -> (x .and. y?=w2310:u16)
                          n670 = And(x=w2311, y=w2312) -> (x .and. y?=w2309:u16)
                          n671 = Not Equal?(x=w2310, y=w2311) -> (x != y?=w2314:bool)
                          n672 = Not Equal?(x=w2311, y=w2309) -> (x != y?=w2313:bool)
                          n673 = And(x=w2314, y=w2313) -> (x .and. y?=w2308:bool)
                          n674 = case shown="True" w2308 {
                            tunnel: w2310 -> [_ w2343]
                            tunnel: w2309 -> [_ w2342]
                            tunnel: w2296 -> [_ w2335]
                            tunnel: w2295 -> [_ w2334]
                            frame False {
                            }
                            frame True {
                              w2330 = 0.03125 ("y")
                              w2341 = 0.03125 ("y")
                              n675 = To Double Precision Float(number=w2335) -> (double precision float=w2332:dbl)
                              n676 = To Double Precision Float(number=w2334) -> (double precision float=w2329:dbl)
                              n677 = To Double Precision Float(number=w2343) -> (double precision float=w2333:dbl)
                              n678 = To Double Precision Float(number=w2342) -> (double precision float=w2326:dbl)
                              n679 = Multiply(x=w2332, y=w2330) -> (x*y=w2331:dbl)
                              n680 = Multiply(x=w2330, y=w2329) -> (x*y=w2328:dbl)
                              n681 = Multiply(x=w2333, y=w2341) -> (x*y=w2327:dbl)
                              n682 = Multiply(x=w2341, y=w2326) -> (x*y=w2325:dbl)
                              n683 = global write "G_rio.vi" "WHL_SPD_FL"(w2331) -> ()
                              n684 = global write "G_rio.vi" "WHL_SPD_FR"(w2328) -> ()
                              n685 = global write "G_rio.vi" "WHL_SPD_RL"(w2327) -> ()
                              n686 = global write "G_rio.vi" "WHL_SPD_RR"(w2325) -> ()
                              n687 = Add(x=w2327, y=w2325) -> (x+y=w2340:dbl)
                              n688 = Multiply(x=w2340, y=0.5) -> (x*y=w2337:dbl)
                              n689 = Multiply(x=w2337, y=1.028) -> (x*y=w2336:dbl)
                              n690 = global write "G_rio.vi" "vs_esc"(w2336) -> ()
                            }
                          }
                        }
                      }
                    }
                    frame 1264 {
                      n691 = flat-sequence {
                        tunnel: [w2347] -> w2344
                        tunnel: [w2346] -> w2345
                        frame #0 {
                          n692 = local read "FPGA VI Reference Out"() -> (w2353:refnum<k20>)
                          n693 = xnode "Read/Write Control"("FPGA VI Reference In"=w2353) -> ("can 4F0"=w2352:u8[])  [unwired: 1 in, 2 out]
                          n694 = Index Array(array=w2352, index #1=0 ("index")) -> (element #1=w2359:u8, element #2=w2358:u8, element #3=w2357:u8, element #4=w2356:u8)  [unwired: 3 in]
                          n695 = Join Numbers(hi=w2359, lo=w2358) -> ((hi.lo)=w2355:u16)
                          n696 = Join Numbers(hi=w2357, lo=w2356) -> ((hi.lo)=w2354:u16)
                          n697 = Join Numbers(hi=w2355, lo=w2354) -> ((hi.lo)=w2348:u32)
                          n698 = Array Subset(array=w2352, index=4) -> (w2346:u8[])  [unwired: 1 in]
                          n699 = feedback #10(u32 0) -> (w2349:u32)
                          n700 = feedback-in #10(w2348) -> ()
                          n701 = Not Equal?(x=w2348, y=w2349) -> (x != y?=w2347:bool)
                        }
                      }
                      n702 = case shown="True" w2344 {
                        tunnel: w2345 -> [_ w2373]
                        frame False {
                        }
                        frame True {
                          # "20 ms"
                          n703 = Index Array(array=w2373, index #1=7 ("index"), index #2=6 ("index"), index #3=5 ("index")) -> (element #1=w2367:u8, element #2=w2369:u8, element #3=w2368:u8)
                          n704 = Join Numbers(hi=w2369, lo=w2368) -> ((hi.lo)=w2364:u16)
                          n705 = Join Numbers(hi=u8 0, lo=w2367) -> ((hi.lo)=w2365:u16)
                          n706 = Join Numbers(hi=w2365, lo=w2364) -> ((hi.lo)=w2362:u32)
                          n707 = Not Equal?(x=u32 16777215, y=w2362) -> (x != y?=w2361:bool)
                          n708 = case shown="True" w2361 {
                            tunnel: w2362 -> [_ w2375]
                            frame False {
                            }
                            frame True {
                              n709 = To Double Precision Float(number=w2375) -> (double precision float=w2374:dbl)
                              n710 = global write "G_rio.vi" "odometer"(w2374) -> ()
                            }
                          }
                        }
                      }
                    }
                    frame 1349 {
                      n711 = flat-sequence {
                        tunnel: [w2379] -> w2376
                        tunnel: [w2378] -> w2377
                        frame #0 {
                          n712 = local read "FPGA VI Reference Out"() -> (w2385:refnum<k20>)
                          n713 = xnode "Read/Write Control"("FPGA VI Reference In"=w2385) -> ("can 545"=w2384:u8[])  [unwired: 1 in, 2 out]
                          n714 = Index Array(array=w2384, index #1=0 ("index")) -> (element #1=w2391:u8, element #2=w2390:u8, element #3=w2389:u8, element #4=w2388:u8)  [unwired: 3 in]
                          n715 = Join Numbers(hi=w2391, lo=w2390) -> ((hi.lo)=w2387:u16)
                          n716 = Join Numbers(hi=w2389, lo=w2388) -> ((hi.lo)=w2386:u16)
                          n717 = Join Numbers(hi=w2387, lo=w2386) -> ((hi.lo)=w2380:u32)
                          n718 = Array Subset(array=w2384, index=4) -> (w2378:u8[])  [unwired: 1 in]
                          n719 = feedback #11(u32 0) -> (w2381:u32)
                          n720 = feedback-in #11(w2380) -> ()
                          n721 = Not Equal?(x=w2380, y=w2381) -> (x != y?=w2379:bool)
                        }
                      }
                      n722 = case shown="True" w2376 {
                        tunnel: w2377 -> [_ w2393]
                        frame False {
                        }
                        frame True {
                          n723 = Index Array(array=w2393, index=3) -> (element=w2395:u8)
                          n724 = Not Equal?(x=w2395, y=u8 255 ("x")) -> (x != y?=w2397:bool)
                          n725 = case shown="True" w2397 {
                            tunnel: w2395 -> [_ w2403]
                            frame False {
                            }
                            frame True {
                              n726 = To Double Precision Float(number=w2403) -> (double precision float=w2402:dbl)
                              n727 = Multiply(x=26.0, y=w2402) -> (x*y=w2400:dbl)
                              n728 = Divide(x=w2400, y=256.0) -> (x/y=w2398:dbl)
                              "battery voltage 2" <- w2398
                              n729 = global write "G_rio.vi" "battery voltage"(w2398) -> ()
                            }
                          }
                        }
                      }
                    }
                  }
                }
                n730 = Or Array Elements(Boolean array=w2076) -> (logical OR=w2075:bool)
              }
              frame Disabled {
              }
            }
            "CAN Comm Enabled" <- w1813
          }
          frame #2 {
            n731 = global read "G_rio.vi" "vs_esc"() -> (w2404:dbl)
            n732 = global read "G_rio.vi" "gear selector disp"() -> (w2408:i8)
            n733 = Negate(x=w2404) -> (-x=w2406:dbl)
            n734 = Equal?(x=w2408, y=u8 7) -> (x = y?=w2407:bool)
            n735 = Select(t=w2406, s=w2407, f=w2404) -> (s? t:f=w2405:dbl)
            "VS_CAN" <- w2405
            n736 = global write "G_rio.vi" "VS_CAN"(w2405) -> ()
          }
          frame #3 {
            n737 = local read "CAN Comm Enabled"() -> (w2411:bool)
            n738 = local read "LCM"() -> (w2412:bool)
            n739 = And(x=w2412, y=w2411) -> (x .and. y?=w2410:bool)
            n740 = case shown="True" w2410 {
              frame False {
              }
              frame True {
                n741 = Get Date/Time In Seconds() -> (seconds since 1Jan1904=w2421:timestamp)
                n742 = global read "G_rio.vi" "time"() -> (w2440:u32)
                n743 = global read "G_rio.vi" "accel pedal value"() -> (w2428:dbl)
                n744 = global read "G_rio.vi" "battery voltage"() -> (w2427:dbl)
                n745 = To Double Precision Float(number=w2421) -> (double precision float=w2420:dbl)
                n746 = global read "G_rio.vi" "mdps str_ang"() -> (w2432:dbl)
                n747 = global read "G_rio.vi" "WHL_SPD_RR"() -> (w2416:dbl)
                n748 = global read "G_rio.vi" "WHL_SPD_RL"() -> (w2415:dbl)
                n749 = global read "G_rio.vi" "WHL_SPD_FR"() -> (w2414:dbl)
                n750 = global read "G_rio.vi" "WHL_SPD_FL"() -> (w2413:dbl)
                n751 = global read "G_rio.vi" "LCM_CAN_T"() -> (w2438:T12)
                n752 = global read "G_rio.vi" "mdps torque"() -> (w2433:dbl)
                n753 = global read "G_rio.vi" "mcp"() -> (w2439:u16)
                n754 = Unbundle By Name(w2438) -> ("hash"=w2437:i64)
                n755 = Multiply(x=w2420, y=1000000.0) -> (x*y=w2418:dbl)
                n756 = global read "G_rio.vi" "odometer"() -> (w2425:dbl)
                n757 = global read "G_rio.vi" "yaw_rate"() -> (w2434:dbl)
                n758 = global read "G_rio.vi" "lat_accel"() -> (w2431:dbl)
                n759 = global read "G_rio.vi" "VS_CAN"() -> (w2426:dbl)
                n760 = To Double Precision Float(number=w2440) -> (double precision float=w2435:dbl)
                n761 = To Quad Integer(1:w2418) -> (0:w2417:i64)
                n762 = call "hash.vi"("input"=w2437) -> ("output"=w2436:i64)  [unwired: 10 in]
                n763 = To Double Precision Float(number=w2439) -> (double precision float=w2430:dbl)
                n764 = global read "G_rio.vi" "tps"() -> (w2429:dbl)
                n765 = Bundle By Name(cluster=w2438, "hash"=w2436, "sys time"=w2417, "time"=w2435, "yaw_rate"=w2434, "mdps torque"=w2433, "mdps str_ang"=w2432, "VS_CAN"=w2426, "lat_accel"=w2431, "mcp"=w2430, "accel pedal value"=w2428, "tps"=w2429, "odometer"=w2425, "battery voltage"=w2427, "WHL_SPD_RR"=w2416, "WHL_SPD_RL"=w2415, "WHL_SPD_FR"=w2414, "WHL_SPD_FL"=w2413) -> (w2424:T12)
                n766 = Flatten To String(anything=w2424, prepend array or string size? (T)=FALSE) -> (data string=w2423:string)  [unwired: 2 in, 2 out]
                n767 = disable-structure shown="Enabled" {
                  disable-tunnel: w2423 -> [w2442 _]
                  frame Enabled {
                    n768 = global read "G_rio.vi" "LCM"() -> (w2443:T4)
                    n769 = call "LCM_send.vi"("DATA"=w2442, "ID"="CAN_T", "LCM"=w2443) -> ()  [unwired: 6 in, 3 out]
                  }
                  frame Disabled {
                  }
                }
              }
            }
          }
        }
      }
      n770 = while {
        stop <- FALSE stop-if-true
        n771 = flat-sequence {
          frame #0 {
            n772 = Wait Until Next ms Multiple(millisecond multiple=u32 10) -> (millisecond timer value=w1374:u32)
            n773 = flat-sequence {
              tunnel: w1374 -> [w1378]
              frame #0 {
                n774 = feedback #12(w1378) -> (w1379:u32)
                n775 = feedback-in #12(w1378) -> ()
                n776 = Subtract(x=w1378, y=w1379) -> (x-y=w1377:u32)
                n777 = To Long Integer(number=w1377) -> (32bit integer=→"Con_time 10":i32)
              }
            }
          }
          frame #1 {
            n778 = flat-sequence {
              frame #0 {
                n779 = local read "LCM"() -> (w1399:bool)
                n780 = case shown="True" w1399 {
                  frame False {
                    n781 = shared-variable "veloster\\sharedvari.lvlib\\vs_des"() -> (w1406:dbl)  [unwired: 1 in, 1 out]
                    n782 = global read "G_rio.vi" "Ref_steer_planner"() -> (w1404:dbl)
                    n783 = global read "G_rio.vi" "Ref_vel_planner"() -> (w1405:dbl)
                    n784 = shared-variable "veloster\\sharedvari.lvlib\\steer_input"() -> (w1403:dbl)  [unwired: 1 in, 1 out]
                    n785 = Not A Number/Path/Refnum?(number/path/refnum=w1406) -> (NaN/Path/Refnum?=w1407:bool)
                    n786 = Select(t=w1405, s=w1407, f=w1406) -> (s? t:f=w1400:dbl)
                    n787 = Not A Number/Path/Refnum?(number/path/refnum=w1403) -> (NaN/Path/Refnum?=w1402:bool)
                    n788 = global write "G_rio.vi" "Ref_vel_planner"(w1400) -> ()
                    n789 = Select(t=w1404, s=w1402, f=w1403) -> (s? t:f=w1401:dbl)
                    n790 = global write "G_rio.vi" "Ref_steer_planner"(w1401) -> ()
                  }
                  frame True {
                    n791 = global read "G_rio.vi" "LCM PC"() -> (w1410:T4)
                    n792 = call "LCM_read.vi"("LCM"=w1410) -> ("data"=w1408:string, "ID"=w1409:string)  [unwired: 7 in, 2 out]
                    n793 = case shown="\"CON_INPUT_T\"" w1409 {
                      tunnel: w1408 -> [_ w1411]
                      frame "False", Default {
                      }
                      frame "CON_INPUT_T" {
                        n794 = global read "G_rio.vi" "CON_INPUT_T"() -> (w1413:T13)
                        n795 = Unflatten From String(type=w1413, binary string=w1411, data includes array or string size? (T)=FALSE) -> (value=w1412:T13, error out=w1414:errorcluster)  [unwired: 2 in, 1 out]
                        n796 = case shown="No Error" w1414 {
                          tunnel: w1412 -> [w1418 _]
                          frame No Error {
                            n797 = Unbundle By Name(w1418) -> ("ref_vel"=w1417:dbl, "ref_steer"=w1416:dbl)
                            n798 = global write "G_rio.vi" "Ref_vel_planner"(w1417) -> ()
                            n799 = global write "G_rio.vi" "Ref_steer_planner"(w1416) -> ()
                          }
                          frame Error {
                          }
                        }
                      }
                    }
                  }
                }
              }
            }
            n800 = global read "G_rio.vi" "Throttle_Enable"() -> (→"Throttle Enable":bool)
            n801 = local read "FPGA VI Reference Out"() -> (w1396:refnum<k20>)
            n802 = xnode "Read/Write Control"("FPGA VI Reference In"=w1396) -> ("Auto"=w1381:bool, "Run"=w1395:bool, "T Lim"=w1397:bool, "brk enc"=w1385:u8)  [unwired: 1 in, 2 out]
            "Auto" <- w1381
            "brk enc" <- w1385
            n803 = global write "G_rio.vi" "Auto"(w1381) -> ()
            n804 = global write "G_rio.vi" "T Lim"(w1397) -> ()
            n805 = To Double Precision Float(number=w1385) -> (double precision float=w1393:dbl)
            n806 = And(x=w1381, y=w1395) -> (x .and. y?=w1382:bool)
            "Run" <- w1382
            n807 = global write "G_rio.vi" "Run"(w1382) -> ()
            n808 = Subtract(x=w1393, y=220.0) -> (x-y=w1391:dbl)
            n809 = Not(x=w1382) -> (.not. x?=w1380:bool)
            n810 = Multiply(x=w1391, y=-100.0) -> (x*y=w1388:dbl)
            n811 = And(x=w1381, y=w1380) -> (x .and. y?=→"E - STOP":bool)
            n812 = Divide(x=w1388, y=175.0) -> (x/y=w1387:dbl)
            n813 = In Range and Coerce(upper limit=100.0, x=w1387, lower limit=0.0) -> (coerced(x)=w1384:dbl)  [unwired: 1 out]
            n814 = global write "G_rio.vi" "brake encoder"(w1384) -> ()
          }
          frame #2 {
            n815 = flat-sequence {
              frame #0 {
                n816 = global read "G_rio.vi" "Ref_vel_planner"() -> (w1462:dbl)
                n817 = Select(t=w1462, s="Velocity input", f="Ref vel manual") -> (s? t:f=w1465:dbl)
                n818 = To Long Integer(number=w1465) -> (32bit integer=w1464:i32)
                n819 = Sign(1:w1464) -> (0:w1463:i32)
                "P, R, D" <- w1463
                n820 = case shown="1" w1463 {
                  tunnel: [w1469 _ w1476] -> w1466
                  tunnel: w1465 -> [w1471 _ w1475]
                  frame -1 {
                    n821 = global read "G_rio.vi" "gear selector disp"() -> (w1474:i8)
                    n822 = Equal?(x=w1474, y=u8 7) -> (x = y?=w1472:bool)
                    n823 = Select(t=w1471, s=w1472, f=0.0) -> (s? t:f=w1469:dbl)
                  }
                  frame 0, Default {
                  }
                  frame 1 {
                    n824 = global read "G_rio.vi" "gear selector disp"() -> (w1477:i8)
                    n825 = case shown="4, 5" w1477 {
                      tunnel: [_ w1478] -> w1476
                      tunnel: w1475 -> [_ w1478]
                      frame 0, Default {
                      }
                      frame 4, 5 {
                      }
                    }
                  }
                }
                "Ref vel" <- w1466
              }
            }
            n826 = feedback #13(FALSE ("Steer input")) -> (w1420:bool)
            n827 = case shown="True" w1420 {
              frame False {
              }
              frame True {
                n828 = flat-sequence {
                  frame #0 {
                    n829 = global read "G_rio.vi" "Ref_steer_planner"() -> (w1425:dbl)
                    n830 = global read "G_rio.vi" "mdps str_ang"() -> (w1428:dbl)
                    n831 = global read "G_rio.vi" "mdps str_ang"() -> (w1427:dbl)
                    n832 = Add(x=w1428, y="steer limit") -> (x+y=w1430:dbl)
                    n833 = Subtract(x=w1427, y="steer limit") -> (x-y=w1429:dbl)
                    n834 = Negate(x="Ref steer manual") -> (-x=w1423:dbl)
                    n835 = Select(t=w1425, s="Steer input", f=w1423) -> (s? t:f=w1426:dbl)
                    n836 = In Range and Coerce(upper limit=w1430, x=w1426, lower limit=w1429) -> (coerced(x)=→"Ref steer":dbl)  [unwired: 1 out]
                  }
                  frame #1 {
                    n837 = local read "Ref steer"() -> (w1436:dbl)
                    n838 = feedback #14(u8 0 ("Con steer alivecnt")) -> (w1433:u8)
                    n839 = Increment(x=w1433) -> (x+1=w1434:u8)
                    n840 = feedback-in #14(w1434) -> ()
                    n841 = global read "G_rio.vi" "Auto"() -> (w1456:bool)
                    n842 = Multiply(x=w1436, y=10.0) -> (x*y=w1449:dbl)
                    n843 = And(x=w1456, y="SPAS Enable") -> (x .and. y?=w1458:bool)
                    n844 = Greater Than 0?(x=w1449) -> (x > 0?=w1450:bool)
                    n845 = Add(x=w1449, y=65536.0) -> (x+y=w1447:dbl)
                    n846 = Select(t=w1449, s=w1450, f=w1447) -> (s? t:f=w1446:dbl)
                    n847 = To Unsigned Word Integer(number=w1446) -> (unsigned 16bit integer=w1445:u16)
                    n848 = Split Number(x=w1445) -> (hi(x)=w1444:u8, lo(x)=w1443:u8)
                    n849 = Build Array(u8 0 ("Con steer status"), w1443, w1444, u8 0 ("element"), w1433, u8 0 ("element"), u8 0 ("element")) -> (w1438:u8[])
                    n850 = Add Array Elements(numeric array=w1438) -> (sum=w1439:u8)
                    n851 = Build Array (concatenate)(w1438, w1439) -> (w1452:u8[])
                    n852 = Bundle By Name(cluster=T2 {"timestamp"=timestamp(0 s since 1904-01-01), "payload"=[0], "identifier"=912, "type"=0, "extended?"=FALSE, "echo?"=FALSE} ("CAN frame"), "payload"=w1452) -> (w1454:T2)
                    n853 = Build Array(w1454) -> (w1455:T2[])
                    n854 = case shown="True" w1458 {
                      tunnel: w1455 -> [_ w1460]
                      frame False {
                      }
                      frame True {
                        n855 = local read "CAN write"() -> (w1459:refnum<k21>)
                        n856 = call-poly <vilib>:"XNET Write.vi"("session in"=w1459, "data"=w1460, "timeout (10)"=0.01) -> ()  [unwired: 11 in, 2 out]
                      }
                    }
                  }
                }
              }
            }
            n857 = Not(x=w1420) -> (.not. x?=w1419:bool)
            n858 = feedback-in #13(w1419) -> ()
          }
          frame #3 {
            n859 = flat-sequence {
              frame #0 {
                n860 = global read "G_rio.vi" "Brake Encoder mcp"() -> (w1539)
                n861 = global read "G_rio.vi" "brake_act_can"() -> (w1538:bool)
                n862 = global read "G_rio.vi" "VS_CAN"() -> (w1540:dbl)
                n863 = local read "Ref vel"() -> (w1537:dbl)
                n864 = call "B_control.vi"("Ref vel"=w1537, "VS_CAN"=w1540, 4:w1539, 5:w1538) -> ("Ref Brk Enc"=w1541:dbl)  [unwired: 15 in]
                n865 = global write "G_rio.vi" "Ref Brk Enc"(w1541) -> ()
              }
            }
            n866 = flat-sequence {
              frame #0 {
                n867 = global read "G_rio.vi" "accel pedal value"() -> (w1535:dbl)
                n868 = global read "G_rio.vi" "VS_CAN"() -> (w1533:dbl)
                n869 = local read "Ref vel"() -> (w1532:dbl)
                n870 = call "T_control.vi"("Ref vel"=w1532, "VS_CAN"=w1533, 4:w1535, "pid gain"=dbl[] [3.0, 0.0, 0.10000000000000003] ("pid gain 1")) -> ("Ref APS"=w1536:dbl)  [unwired: 15 in]
                n871 = global write "G_rio.vi" "Ref APS"(w1536) -> ()
              }
            }
            n872 = global read "G_rio.vi" "Auto"() -> (w1479:bool)
            n873 = case shown="False" w1479 {
              tunnel: [w1481 w1515] -> w1480
              frame False {
                n874 = global read "G_rio.vi" "VS_CAN"() -> (w1485:dbl)
                n875 = Absolute Value(x=w1485) -> (abs(x)=w1484:dbl)
                n876 = Less?(x=w1484, y=0.05) -> (x < y?=w1482:bool)
                n877 = case shown="True" w1482 {
                  tunnel: [_ w1488] -> w1481
                  frame False {
                  }
                  frame True {
                    n878 = Sign(1:"Gear Manual") -> (0:w1489:i32)
                    n879 = To Long Integer(number=w1489) -> (32bit integer=w1487:i32)
                    n880 = case shown="0" w1487 {
                      tunnel: [w1496 w1500 w1504] -> w1488
                      frame 0 {
                        n881 = global read "G_rio.vi" "gear selector disp"() -> (w1494:i8)
                        n882 = Equal To 0?(x=w1494) -> (x = 0?=w1493:bool)
                        n883 = Equal?(x=u8 7 ("y"), y=w1494) -> (x = y?=w1498:bool)
                        n884 = Select(t=-1.0, s=w1493, f=1.0) -> (s? t:f=w1492:dbl)
                        n885 = Select(t=0.0, s=w1498, f=w1492) -> (s? t:f=w1496:dbl)
                      }
                      frame 1, Default {
                        n886 = global read "G_rio.vi" "gear selector disp"() -> (w1503:i8)
                        n887 = Equal To 0?(x=w1503) -> (x = 0?=w1502:bool)
                        n888 = Select(t=0.0, s=w1502, f=1.0 ("t")) -> (s? t:f=w1500:dbl)
                      }
                      frame -1 {
                        n889 = global read "G_rio.vi" "gear selector disp"() -> (w1505:i8)
                        n890 = case shown="3..5, Default" w1505 {
                          tunnel: [-1.0 1.0 0.0] -> w1504
                          frame 0, 6, 7 {
                          }
                          frame 1, 2 {
                          }
                          frame 3..5, Default {
                          }
                        }
                      }
                    }
                  }
                }
              }
              frame True {
                n891 = global read "G_rio.vi" "VS_CAN"() -> (w1512:dbl)
                n892 = Absolute Value(x=w1512) -> (abs(x)=w1511:dbl)
                n893 = Less?(x=w1511, y=0.05) -> (x < y?=w1509:bool)
                n894 = global read "G_rio.vi" "Run"() -> (w1514:bool)
                n895 = And(x=w1509, y=w1514) -> (x .and. y?=w1513:bool)
                n896 = case shown="True" w1513 {
                  tunnel: [_ w1517] -> w1515
                  frame False {
                  }
                  frame True {
                    n897 = local read "P, R, D"() -> (w1516:i32)
                    n898 = case shown="-1" w1516 {
                      tunnel: [w1518 w1523 w1527] -> w1517
                      frame -1 {
                        n899 = global read "G_rio.vi" "gear selector disp"() -> (w1519:i8)
                        n900 = case shown="0" w1519 {
                          tunnel: [-1.0 ("t") 1.0 ("t") _ _] -> w1518
                          frame 0 {
                          }
                          frame 1, Default {
                          }
                          frame 4, 8 {
                          }
                          frame 7 {
                          }
                        }
                      }
                      frame 0, Default {
                        n901 = global read "G_rio.vi" "gear selector disp"() -> (w1526:i8)
                        n902 = Equal To 0?(x=w1526) -> (x = 0?=w1525:bool)
                        n903 = Select(t=0.0, s=w1525, f=1.0 ("t")) -> (s? t:f=w1523:dbl)
                      }
                      frame 1 {
                        n904 = global read "G_rio.vi" "gear selector disp"() -> (w1528:i8)
                        n905 = case shown="1, 2" w1528 {
                          tunnel: [-1.0 1.0 0.0] -> w1527
                          frame 0, 6, 7 {
                          }
                          frame 1, 2 {
                          }
                          frame 3..5, Default {
                          }
                        }
                      }
                    }
                  }
                }
              }
            }
            "shift lever" <- w1480
          }
          frame #4 {
            n906 = flat-sequence {
              tunnel: [w1549] -> w1544
              tunnel: [w1548] -> w1543
              tunnel: [w1545] -> w1542
              tunnel: w1544 -> [w1770]
              tunnel: w1543 -> [w1772]
              tunnel: w1542 -> [w1771]
              frame #0 {
                n907 = global read "G_rio.vi" "Auto"() -> (w1547:bool)
                n908 = flat-sequence {
                  tunnel: [w1561] -> w1550
                  frame #0 {
                    n909 = global read "G_rio.vi" "accel pedal value"() -> (w1553:dbl)
                    n910 = global read "G_rio.vi" "Throttle_Enable"() -> (w1558:bool)
                    n911 = global read "G_rio.vi" "brake_act_can"() -> (w1554:bool)
                    n912 = Equal To 0?(x=w1553) -> (x = 0?=w1552:bool)
                    n913 = case shown="True" w1552 {
                      tunnel: [TRUE w1564] -> w1555
                      frame False {
                        n914 = global write "G_rio.vi" "T lim counter 2"(u16 300 ("T lim counter 2")) -> ()
                      }
                      frame True {
                        n915 = global read "G_rio.vi" "T lim counter 2"() -> (w1566:u16)
                        n916 = Decrement(x=w1566) -> (x-1=w1567:u16)
                        n917 = Max & Min(x=u16 0, y=w1567) -> (max(x,y)=w1565:u16)  [unwired: 1 out]
                        n918 = global write "G_rio.vi" "T lim counter 2"(w1565) -> ()
                        n919 = Not Equal To 0?(x=w1565) -> (x != 0?=w1564:bool)
                      }
                    }
                    n920 = Not(x=w1554) -> (.not. x?=w1559:bool)
                    n921 = local read "Ref vel"() -> (w1551:dbl)
                    n922 = Not Equal To 0?(x=w1551) -> (x != 0?=w1560:bool)
                    n923 = global read "G_rio.vi" "Auto"() -> (w1556:bool)
                    n924 = global read "G_rio.vi" "Run"() -> (w1557:bool)
                    n925 = Compound Arithmetic op=AND(w1556, w1557, w1560, w1559, w1558, w1555) -> (w1561:bool)
                  }
                }
                n926 = case shown="True" w1547 {
                  tunnel: [w1597 w1606] -> w1546
                  frame False {
                    n927 = global read "G_rio.vi" "Brake Encoder mcp"() -> (w1594)
                    n928 = global read "G_rio.vi" "brake encoder"() -> (w1593:dbl)
                    n929 = Not Equal To 0?(x=w1593) -> (x != 0?=w1596:bool)
                    n930 = Subtract(x=0.0, y=w1594) -> (x-y=w1598:dbl)
                    n931 = Select(t=w1598, s=w1596, f=0.0) -> (s? t:f=w1597:dbl)
                  }
                  frame True {
                    n932 = global read "G_rio.vi" "Run"() -> (w1609:bool)
                    n933 = global read "G_rio.vi" "Brake Encoder mcp"() -> (w1608)
                    n934 = case shown="True" w1609 {
                      tunnel: [w1610 w1612] -> w1604
                      frame False {
                        n935 = global read "G_rio.vi" "Ref Brk FULL"() -> (w1610:dbl)
                      }
                      frame True {
                        n936 = local read "Ref vel"() -> (w1611:dbl)
                        n937 = global read "G_rio.vi" "Ref Brk FULL"() -> (w1613:dbl)
                        n938 = global read "G_rio.vi" "Ref Brk Enc"() -> (w1615:dbl)
                        n939 = Equal To 0?(x=w1611) -> (x = 0?=w1616:bool)
                        n940 = Select(t=w1613, s=w1616, f=w1615) -> (s? t:f=w1614:dbl)
                        n941 = Max & Min(x=w1613, y=w1614) -> (min(x,y)=w1612:dbl)  [unwired: 1 out]
                      }
                    }
                    n942 = global read "G_rio.vi" "brake encoder"() -> (w1601:dbl)
                    n943 = Equal To 0?(x=w1601) -> (x = 0?=w1602:bool)
                    n944 = Subtract(x=w1604, y=w1608) -> (x-y=w1605:dbl)
                    n945 = Equal To 0?(x=w1604) -> (x = 0?=w1603:bool)
                    n946 = And(x=w1602, y=w1603) -> (x .and. y?=w1600:bool)
                    n947 = Select(t=0.0, s=w1600, f=w1605) -> (s? t:f=w1606:dbl)
                  }
                }
                n948 = flat-sequence {
                  tunnel: w1546 -> [w1579]
                  tunnel: [w1574] -> w1545
                  frame #0 {
                    n949 = Multiply(x=w1579, y=-0.01) -> (x*y=w1581:dbl)
                    n950 = In Range and Coerce(upper limit=1.0 ("x"), x=w1581, lower limit=-1.0) -> (coerced(x)=w1569:dbl)  [unwired: 1 out]
                    n951 = flat-sequence {
                      tunnel: w1569 -> [w1585]
                      tunnel: [w1591] -> w1570
                      frame #0 {
                        w1584 = 0.2 ("x")
                        n952 = Multiply(x=w1585, y=w1584) -> (x*y=w1589:dbl)
                        n953 = Subtract(x=1.0, y=w1584) -> (x-y=w1587:dbl)
                        n954 = feedback #15(0.0) -> (w1586:dbl)
                        n955 = Multiply(x=w1587, y=w1586) -> (x*y=w1588:dbl)
                        n956 = Add(x=w1589, y=w1588) -> (x+y=w1591:dbl)
                        n957 = feedback-in #15(w1591) -> ()
                      }
                    }
                    n958 = Multiply(x=w1569, y=1.8 ("B P gain")) -> (x*y=w1576:dbl)
                    n959 = call "deadzone.vi"("min"=-15.0, "max"=15.0, "x"=w1570) -> ("dead zone"=w1571:dbl)  [unwired: 8 in]
                    n960 = Multiply(x=w1571, y=0.1 ("B D gain")) -> (x*y=w1575:dbl)
                    n961 = Add(x=w1575, y=w1576) -> (x+y=w1574:dbl)
                  }
                }
                n962 = case shown="True" w1550 {
                  tunnel: [_ TRUE] -> w1549
                  tunnel: [w1617 w1636] -> w1548
                  frame False {
                    n963 = flat-sequence {
                      tunnel: [w1627] -> w1617
                      frame #0 {
                        n964 = global read "G_rio.vi" "T Lim"() -> (w1618:bool)
                        n965 = case shown="True" w1618 {
                          selector: w1618 -> [_ w1625]
                          frame False {
                            n966 = global write "G_rio.vi" "T lim counter"(u16 0 ("T lim counter")) -> ()
                          }
                          frame True {
                            n967 = global write "G_rio.vi" "T lim once"(w1625) -> ()
                            n968 = global write "G_rio.vi" "T lim counter 2"(u16 300 ("T lim counter 2")) -> ()
                            n969 = global read "G_rio.vi" "T lim counter"() -> (w1624:u16)
                            n970 = Increment(x=w1624) -> (x+1=w1623:u16)
                            n971 = Max & Min(x=u16 100, y=w1623) -> (min(x,y)=w1622:u16)  [unwired: 1 out]
                            n972 = global write "G_rio.vi" "T lim counter"(w1622) -> ()
                          }
                        }
                      }
                      frame #1 {
                        n973 = global read "G_rio.vi" "T lim once"() -> (w1626:bool)
                        n974 = case shown="True" w1626 {
                          tunnel: [-1.0 ("t") w1632] -> w1627
                          frame False {
                          }
                          frame True {
                            n975 = global read "G_rio.vi" "T lim counter"() -> (w1631:u16)
                            n976 = Equal?(x=w1631, y=u16 100) -> (x = y?=w1630:bool)
                            n977 = Select(t=0.0, s=w1630, f=-0.15) -> (s? t:f=w1632:dbl)
                          }
                        }
                        n978 = global write "G_rio.vi" "Throttle_Enable"(w1626) -> ()
                      }
                    }
                  }
                  frame True {
                    n979 = disable-structure shown="Enabled" {
                      disable-tunnel: [w1655 w1711] -> w1636
                      frame Enabled {
                        n980 = global read "G_rio.vi" "Ref APS"() -> (w1660:dbl)
                        n981 = global read "G_rio.vi" "accel pedal value"() -> (w1658:dbl)
                        n982 = global read "G_rio.vi" "accel pedal value"() -> (w1647:dbl)
                        n983 = global read "G_rio.vi" "accel pedal value"() -> (w1659:dbl)
                        n984 = Subtract(x=w1660, y=w1659) -> (x-y=w1646:dbl)
                        n985 = Greater?(x=w1658, y=95.0) -> (0:w1649:bool)
                        n986 = flat-sequence {
                          tunnel: w1646 -> [w1681]
                          tunnel: [w1678] -> w1654
                          frame #0 {
                            n987 = feedback #16(0.0) -> (w1686:dbl)
                            n988 = feedback-in #16(w1681) -> ()
                            n989 = Subtract(x=w1681, y=w1686) -> (x-y=w1685:dbl)
                            n990 = Multiply(x=w1681, y=0.01) -> (x*y=w1682:dbl)
                            n991 = feedback #17(0.0) -> (w1677:dbl)
                            n992 = Multiply(x=0.999, y=w1677) -> (x*y=w1676:dbl)
                            n993 = Add(x=w1682, y=w1676) -> (x+y=w1673:dbl)
                            n994 = feedback-in #17(w1673) -> ()
                            n995 = Divide(x=w1685, y=0.01) -> (x/y=w1672:dbl)
                            n996 = Build Array(w1681, w1673, w1672) -> (w1680:dbl[])
                            n997 = Multiply(x=w1680, y=dbl[] [8.0, 0.02, 0.4] ("pid gain 2")) -> (x*y=w1679:dbl[])
                            n998 = Add Array Elements(numeric array=w1679) -> (sum=w1678:dbl)
                          }
                        }
                        n999 = Equal To 0?(x=w1647) -> (x = 0?=w1639:bool)
                        n1000 = Greater Than 0?(x=w1646) -> (x > 0?=w1648:bool)
                        n1001 = Less Than 0?(x=w1646) -> (x < 0?=w1640:bool)
                        n1002 = And(x=w1649, y=w1648) -> (x .and. y?=w1644:bool)
                        n1003 = And(x=w1639, y=w1640) -> (x .and. y?=w1645:bool)
                        n1004 = Or(x=w1644, y=w1645) -> (x .or. y?=w1643:bool)
                        n1005 = Multiply(x=w1654, y=0.01) -> (x*y=w1652:dbl)
                        n1006 = In Range and Coerce(upper limit=1.0 ("x"), x=w1652, lower limit=-1.0) -> (coerced(x)=w1642:dbl)  [unwired: 1 out]
                        n1007 = flat-sequence {
                          tunnel: w1642 -> [w1662]
                          tunnel: [w1668] -> w1641
                          frame #0 {
                            w1661 = 0.5 ("x")
                            n1008 = Multiply(x=w1662, y=w1661) -> (x*y=w1666:dbl)
                            n1009 = Subtract(x=1.0, y=w1661) -> (x-y=w1664:dbl)
                            n1010 = feedback #18(0.0) -> (w1663:dbl)
                            n1011 = Multiply(x=w1664, y=w1663) -> (x*y=w1665:dbl)
                            n1012 = Add(x=w1666, y=w1665) -> (x+y=w1668:dbl)
                            n1013 = feedback-in #18(w1668) -> ()
                          }
                        }
                        n1014 = Select(t=0.0 ("f"), s=w1643, f=w1641) -> (s? t:f=w1655:dbl)
                      }
                      frame Disabled {
                        n1015 = global read "G_rio.vi" "VS_CAN"() -> (w1713:dbl)
                        n1016 = global read "G_rio.vi" "VS_CAN"() -> (w1699:dbl)
                        n1017 = local read "Ref vel"() -> (w1714:dbl)
                        n1018 = Divide(x=dbl[] [-100.0, -3.0, -1.0, 1.0, 3.0, 100.0] ("array_x"), y=3.6) -> (x/y=w1689:dbl[])
                        n1019 = Divide(x=w1699, y=3.6) -> (x/y=w1697:dbl)
                        n1020 = Subtract(x=w1714, y=w1713) -> (x-y=w1692:dbl)
                        n1021 = feedback #19(0.0 ("y")) -> (w1704:dbl)
                        n1022 = feedback-in #19(w1697) -> ()
                        n1023 = Subtract(x=w1697, y=w1704) -> (x-y=w1703:dbl)
                        n1024 = Divide(x=w1692, y=3.6) -> (x/y=w1688:dbl)
                        n1025 = call "lookuptable.vi"("array_y"=dbl[] [-0.5, -0.1, -0.01, 0.01, 0.1, 0.5] ("array_x"), "array_x"=w1689, "x"=w1688) -> ("y"=w1707:dbl)  [unwired: 8 in]
                        n1026 = Multiply(x=100.0, y=w1703) -> (x*y=w1701:dbl)
                        n1027 = Multiply(x=1.0 ("P_gain"), y=w1707) -> (x*y=w1696:dbl)
                        n1028 = Multiply(x=0.0 ("D_gain"), y=w1701) -> (x*y=w1695:dbl)
                        n1029 = Subtract(x=w1696, y=w1695) -> (x-y=w1694:dbl)
                        n1030 = flat-sequence {
                          tunnel: w1694 -> [w1716]
                          tunnel: [w1715] -> w1687
                          frame #0 {
                            n1031 = feedback #20(0.0 ("y")) -> (w1723:dbl)
                            n1032 = Multiply(x=-0.01, y=999.0) -> (x*y=w1722:dbl)
                            n1033 = Multiply(x=0.7 ("Rate"), y=0.01 ("x")) -> (x*y=w1718:dbl)
                            n1034 = Add(x=w1718, y=w1723) -> (x+y=w1725:dbl)
                            n1035 = Add(x=w1723, y=w1722) -> (x+y=w1724:dbl)
                            n1036 = In Range and Coerce(upper limit=w1725, x=w1716, lower limit=w1724) -> (coerced(x)=w1715:dbl)  [unwired: 1 out]
                            n1037 = feedback-in #20(w1715) -> ()
                          }
                        }
                        n1038 = In Range and Coerce(upper limit=1.0, x=w1687, lower limit=-1.0) -> (coerced(x)=w1708:dbl)  [unwired: 1 out]
                        n1039 = flat-sequence {
                          tunnel: w1708 -> [w1728]
                          tunnel: [w1727] -> w1711
                          frame #0 {
                            n1040 = Greater Than 0?(x=w1728) -> (x > 0?=w1736:bool)
                            n1041 = global read "G_rio.vi" "accel pedal value"() -> (w1739:dbl)
                            n1042 = global read "G_rio.vi" "accel pedal value"() -> (w1735:dbl)
                            n1043 = Less Than 0?(x=w1728) -> (x < 0?=w1734:bool)
                            n1044 = Equal To 0?(x=w1735) -> (x = 0?=w1733:bool)
                            n1045 = Greater?(x=w1739, y=95.0) -> (0:w1737:bool)
                            n1046 = And(x=w1737, y=w1736) -> (x .and. y?=w1732:bool)
                            n1047 = And(x=w1734, y=w1733) -> (x .and. y?=w1731:bool)
                            n1048 = Or(x=w1732, y=w1731) -> (x .or. y?=w1730:bool)
                            n1049 = Select(t=0.0, s=w1730, f=w1728) -> (s? t:f=w1727:dbl)
                          }
                        }
                      }
                    }
                    n1050 = global write "G_rio.vi" "T lim counter"(u16 0 ("T lim counter")) -> ()
                    n1051 = global write "G_rio.vi" "T lim once"(FALSE ("T lim once")) -> ()
                  }
                }
              }
              frame #1 {
                n1052 = local read "shift lever"() -> (w1742:dbl)
                n1053 = disable-structure shown="Enabled" {
                  disable-tunnel: [w1773 _] -> w1741
                  frame Enabled {
                    n1054 = global read "G_rio.vi" "Auto"() -> (w1777:bool)
                    n1055 = global read "G_rio.vi" "Run"() -> (w1776:bool)
                    n1056 = Compound Arithmetic op=AND(w1777, w1776) -> (w1775:bool)
                    n1057 = And(x=w1775, y="buzz") -> (x .and. y?=w1773:bool)
                  }
                  frame Disabled {
                  }
                }
                n1058 = local read "FPGA VI Reference Out"() -> (w1751:refnum<k20>)
                n1059 = Multiply(x=w1771, y=600.0 ("B gain")) -> (x*y=w1746:dbl)
                n1060 = Multiply(x=w1772, y=500.0 ("T gain")) -> (x*y=w1768:dbl)
                n1061 = Multiply(x=w1742, y=250.0 ("S gain")) -> (x*y=w1753:dbl)
                n1062 = In Range and Coerce(upper limit=500.0, x=w1768, lower limit=-500.0) -> (coerced(x)=w1744:dbl)  [unwired: 1 out]
                n1063 = Select(t=w1746, s="brake", f="Slide") -> (s? t:f=w1748:dbl)
                n1064 = In Range and Coerce(upper limit=500.0, x=w1753, lower limit=-500.0) -> (coerced(x)=w1756:dbl)  [unwired: 1 out]
                n1065 = Add(x=w1744, y=1500.0) -> (x+y=w1764:dbl)
                n1066 = In Range and Coerce(upper limit=500.0, x=w1748, lower limit=-500.0) -> (coerced(x)=w1750:dbl)  [unwired: 1 out]
                n1067 = Add(x=w1756, y=1500.0) -> (x+y=w1758:dbl)
                n1068 = To Unsigned Word Integer(number=w1764) -> (unsigned 16bit integer=w1740:u16)
                "T PWM" <- w1740
                n1069 = Add(x=w1750, y=1500.0) -> (x+y=w1763:dbl)
                n1070 = To Unsigned Word Integer(number=w1763) -> (unsigned 16bit integer=w1749:u16)
                "B PWM" <- w1749
                n1071 = To Unsigned Word Integer(number=w1758) -> (unsigned 16bit integer=w1743:u16)
                n1072 = xnode "Read/Write Control"("FPGA VI Reference In"=w1751, "Buzz"=w1741, "S Pwm 1"=w1743, "S Pwm 2"=w1743, "B Pwm"=w1749, "T Pwm"=w1740, "Solenoid"=w1770) -> ()  [unwired: 1 in, 2 out]
                "solenoid" <- w1770
              }
              frame #2 {
                n1073 = local read "LCM"() -> (w1778:bool)
                n1074 = case shown="True" w1778 {
                  frame False {
                    n1075 = global read "G_rio.vi" "Auto"() -> (w1779:bool)
                    n1076 = global read "G_rio.vi" "Run"() -> (w1780:bool)
                    n1077 = global read "G_rio.vi" "VS_CAN"() -> (w1782:dbl)
                    n1078 = shared-variable "veloster\\sharedvari.lvlib\\auto"(w1779) -> ()  [unwired: 1 in, 1 out]
                    n1079 = shared-variable "veloster\\sharedvari.lvlib\\run"(w1780) -> ()  [unwired: 1 in, 1 out]
                    n1080 = global read "G_rio.vi" "mdps str_ang"() -> (w1781:dbl)
                    n1081 = shared-variable "veloster\\sharedvari.lvlib\\vs_can"(w1782) -> ()  [unwired: 1 in, 1 out]
                    n1082 = shared-variable "veloster\\sharedvari.lvlib\\steer_output"(w1781) -> ()  [unwired: 1 in, 1 out]
                  }
                  frame True {
                    n1083 = Get Date/Time In Seconds() -> (seconds since 1Jan1904=w1787:timestamp)
                    n1084 = global read "G_rio.vi" "Ref Brk Enc"() -> (w1790:dbl)
                    n1085 = local read "solenoid"() -> (w1795:bool)
                    n1086 = global read "G_rio.vi" "Ref APS"() -> (w1789:dbl)
                    n1087 = local read "Ref steer"() -> (w1788:dbl)
                    n1088 = local read "brk enc"() -> (w1794:u8)
                    n1089 = local read "B PWM"() -> (w1793:u16)
                    n1090 = local read "T PWM"() -> (w1792:u16)
                    n1091 = To Double Precision Float(number=w1787) -> (double precision float=w1786:dbl)
                    n1092 = global read "G_rio.vi" "LCM_CON_T"() -> (w1806:T14)
                    n1093 = Unbundle By Name(w1806) -> ("hash"=w1804:i64)
                    n1094 = Multiply(x=w1786, y=1000000.0) -> (x*y=w1784:dbl)
                    n1095 = To Quad Integer(1:w1784) -> (0:w1783:i64)
                    n1096 = call "hash.vi"("input"=w1804) -> ("output"=w1803:i64)  [unwired: 10 in]
                    n1097 = local read "Ref vel"() -> (w1791:dbl)
                    n1098 = global read "G_rio.vi" "T Lim"() -> (w1796:bool)
                    n1099 = global read "G_rio.vi" "Auto"() -> (w1798:bool)
                    n1100 = global read "G_rio.vi" "Run"() -> (w1797:bool)
                    n1101 = Bundle(cluster=w1806, "hash"=w1803, "sys time"=w1783, "Auto"=w1798, "Run"=w1797, "Solenoid"=w1795, "T lim"=w1796, "brk_enc"=w1794, "B PWM"=w1793, "T PWM"=w1792, "ref_vel"=w1791, "ref_bkr_enc"=w1790, "ref_apv"=w1789, "ref_steer"=w1788) -> (w1799:T14)
                    n1102 = Flatten To String(anything=w1799, prepend array or string size? (T)=FALSE) -> (data string=w1801:string)  [unwired: 2 in, 2 out]
                    n1103 = global read "G_rio.vi" "LCM"() -> (w1800:T4)
                    n1104 = call "LCM_send.vi"("DATA"=w1801, "ID"="CON_T", "LCM"=w1800) -> ()  [unwired: 6 in, 3 out]
                  }
                }
              }
            }
          }
        }
      }
      n1105 = flat-sequence {
        tunnel: [w70] -> w65
        frame #0 {
          w66 = FALSE ("get heading")
          w73 = u64 1
          w72 = 0.0 ("dh_hat")
          w74 = 1.0 ("initH")
          n1106 = local write "GPS init"(w66) -> ()
          n1107 = call "angleconv.vi"("deg"=204.0 ("Real Matrix Element")) -> ("rad"=w67:dbl)  [unwired: 9 in, 1 out]
          n1108 = Replace Array Subset(array=dbl[] [0.0, 0.0, 0.0, 0.0, 0.0] ("pos(i)"), new element=w67, index=3) -> (w70:dbl[])
          "dh_hat" <- w72
          "initH" <- w74
          "dh" <- w72
          "dx_hat" <- w72
          "dy_hat" <- w72
          "initP" <- w74
          "dx" <- w72
          "dy" <- w72
          "vgain" <- w74
          "vcount" <- w73
          "hbias" <- w72
          "hcount" <- w73
          "get heading" <- w66
          "get position" <- w66
          "heading error" <- w72
          "h_gps" <- w72
          "rt" <- w72
          "pos error" <- w72
        }
      }
      n1109 = while {
        shift-right: [w500] -> _
        shift-left: w65 -> [w499]
        stop <- FALSE stop-if-true
        n1110 = flat-sequence {
          tunnel: [w504] -> w496
          tunnel: w499 -> [w504]
          tunnel: w496 -> [w518]
          tunnel: [w519] -> w497
          tunnel: [w517] -> w495
          tunnel: [w1227] -> w500
          tunnel: w497 -> [w1228]
          tunnel: w495 -> [w1227]
          frame #0 {
            n1111 = disable-structure shown="Disabled" {
              disable-tunnel: [_ w507] -> w501
              frame Disabled {
                n1112 = global read "G_rio.vi" "timestamp"() -> (w505)
                n1113 = feedback #21(w505) -> (w506)
                n1114 = feedback-in #21(w505) -> ()
                n1115 = Subtract(x=w505, y=w506) -> ()  [unwired: 1 out]
              }
              frame Enabled {
                n1116 = global read "G_rio.vi" "time"() -> (w509:u32)
                n1117 = feedback #22(w509) -> (w508:u32)
                n1118 = feedback-in #22(w509) -> ()
                n1119 = Subtract(x=w509, y=w508) -> (x-y=w510:u32)
                n1120 = To Double Precision Float(number=w510) -> (double precision float=w511:dbl)
                n1121 = Multiply(x=w511, y=1e-06) -> (x*y=w507:dbl)
              }
            }
            "dt" <- w501
            n1122 = Wait Until Next ms Multiple(millisecond multiple=u32 10) -> (millisecond timer value=w502:u32)
            n1123 = flat-sequence {
              tunnel: w502 -> [w515]
              frame #0 {
                n1124 = feedback #23(w515) -> (w516:u32)
                n1125 = feedback-in #23(w515) -> ()
                n1126 = Subtract(x=w515, y=w516) -> (x-y=w514:u32)
                n1127 = To Long Integer(number=w514) -> (32bit integer=→"Pos_time 10":i32)
              }
            }
          }
          frame #1 {
            n1128 = disable-structure shown="Enabled" {
              disable-tunnel: [w520 w934] -> w519
              disable-tunnel: w518 -> [w521 w956]
              disable-tunnel: [w520 w943] -> w517
              frame Enabled {
                n1129 = flat-sequence {
                  tunnel: w521 -> [w534]
                  tunnel: [w534] -> w522
                  tunnel: [w666] -> w520
                  tunnel: w522 -> [w667]
                  frame #0 {
                    n1130 = case shown="True" "ublox" {
                      tunnel: [w535 w548] -> w525
                      tunnel: [w536 w566] -> w528
                      frame False {
                        n1131 = global read "G_rio.vi" "dgps_vel"() -> (w547:dbl[])
                        n1132 = Index Array(array=w547, index #1=0 ("index"), index #2=1 ("index"), index #3=4 ("index")) -> (element #1=w538:dbl, element #2=w543:dbl, element #3=w540:dbl)
                        n1133 = feedback #24(0.0 ("Real Matrix Element")) -> (w537:dbl)
                        n1134 = feedback-in #24(w538) -> ()
                        n1135 = Not Equal?(x=w538, y=w537) -> (x != y?=w544:bool)
                        n1136 = Not Equal To 0?(x=w543) -> (x != 0?=w542:bool)
                        n1137 = And(x=w544, y=w542) -> (x .and. y?=w535:bool)
                        n1138 = call "angleconv.vi"("deg"=w540) -> ("rad"=w536:dbl)  [unwired: 9 in, 1 out]
                      }
                      frame True {
                        n1139 = global read "G_rio.vi" "gps_vel 1"() -> (w593:dbl[])
                        n1140 = global read "G_rio.vi" "gps_vel 2"() -> (w572:dbl[])
                        n1141 = global read "G_rio.vi" "VS_CAN"() -> (w551:dbl)
                        n1142 = Index Array(array=w593, index #1=0 ("index"), index #2=1 ("index"), index #3=4 ("index"), index #4=2 ("index")) -> (element #1=w584:dbl, element #2=w589:dbl, element #3=w586:dbl, element #4=w556:dbl)
                        n1143 = Index Array(array=w572, index #1=0 ("index"), index #2=1 ("index"), index #3=4 ("index"), index #4=2 ("index")) -> (element #1=w581:dbl, element #2=w576:dbl, element #3=w579:dbl, element #4=w555:dbl)
                        n1144 = Add(x=w556, y=w555) -> (x+y=w554:dbl)
                        n1145 = call "angleconv.vi"("deg"=w586) -> ("rad"=w569:dbl)  [unwired: 9 in, 1 out]
                        n1146 = Not Equal To 0?(x=w576) -> (x != 0?=w577:bool)
                        n1147 = call "angleconv.vi"("deg"=w579) -> ("rad"=w568:dbl)  [unwired: 9 in, 1 out]
                        n1148 = feedback #25(0.0 ("Real Matrix Element")) -> (w583:dbl)
                        n1149 = feedback-in #25(w584) -> ()
                        n1150 = feedback #26(0.0 ("Real Matrix Element")) -> (w582:dbl)
                        n1151 = feedback-in #26(w581) -> ()
                        n1152 = Not Equal?(x=w584, y=w583) -> (x != y?=w590:bool)
                        n1153 = Not Equal?(x=w581, y=w582) -> (x != y?=w575:bool)
                        n1154 = Not Equal To 0?(x=w589) -> (x != 0?=w588:bool)
                        n1155 = Absolute Value(x=w551) -> (abs(x)=w563:dbl)
                        n1156 = Multiply(x=w554, y=0.5) -> (x*y=w564:dbl)
                        n1157 = call "headingweightsum.vi"("a"=0.5, "h1"=w568, "h2"=w569) -> ("a*h2+(1-a)*h1"=w566:dbl)  [unwired: 8 in]
                        n1158 = And(x=w590, y=w588) -> (x .and. y?=w571:bool)
                        n1159 = And(x=w575, y=w577) -> (x .and. y?=w570:bool)
                        n1160 = Divide(x=w564, y=w563) -> (x/y=w565:dbl)
                        n1161 = And(x=w571, y=w570) -> (x .and. y?=w548:bool)
                        n1162 = Decrement(x=w565) -> (x-1=w560:dbl)
                        n1163 = Absolute Value(x=w560) -> (abs(x)=w561:dbl)
                        n1164 = Greater?(x=w551, y=15.0) -> (0:w549:bool)
                        n1165 = Less?(x=w561, y=0.05) -> (x < y?=w553:bool)
                        n1166 = Compound Arithmetic op=AND(w549, w553, w548) -> (w552:bool)
                        n1167 = case shown="True" w552 {
                          tunnel: w565 -> [_ w601]
                          frame False {
                          }
                          frame True {
                            w595 = u64 18446744073709551615
                            n1168 = local read "vcount"() -> (w598:u64)
                            n1169 = local read "vgain"() -> (w603:dbl)
                            n1170 = Increment(x=w598) -> (x+1=w597:u64)
                            n1171 = Multiply(x=w603, y=w598) -> (x*y=w602:dbl)
                            n1172 = Not Equal?(x=w598, y=w595) -> (x != y?=w596:bool)
                            n1173 = Add(x=w601, y=w602) -> (x+y=w600:dbl)
                            n1174 = Select(t=w597, s=w596, f=w595) -> (s? t:f=w594:u64)
                            n1175 = local write "vcount"(w594) -> ()
                            n1176 = Divide(x=w600, y=w594) -> (x/y=w599:dbl)
                            n1177 = local write "vgain"(w599) -> ()
                          }
                        }
                      }
                    }
                    n1178 = case shown="True" "ublox" {
                      tunnel: [w605 w638] -> w524
                      tunnel: [w606 w633] -> w523
                      tunnel: [w604 w622] -> _
                      frame False {
                        n1179 = global read "G_rio.vi" "dgps_pos"() -> (w606:dbl[])
                        n1180 = Index Array(array=w606, index #1=0 ("index"), index #2=1 ("index"), index #3=9 ("index")) -> (element #1=w609:dbl, element #2=w612:dbl, element #3=w615:dbl, element #4=w616:dbl)  [unwired: 1 in]
                        n1181 = Square(x=w615) -> (x^2=w617:dbl)
                        n1182 = Square(x=w616) -> (x^2=w618:dbl)
                        n1183 = feedback #27() -> (w608:dbl)  [unwired: 1 in]
                        n1184 = feedback-in #27(w609) -> ()
                        n1185 = Not Equal?(x=w609, y=w608) -> (x != y?=w610:bool)
                        n1186 = Add(x=w617, y=w618) -> (x+y=w619:dbl)
                        n1187 = Not Equal To 0?(x=w612) -> (x != 0?=w613:bool)
                        n1188 = And(x=w610, y=w613) -> (x .and. y?=w605:bool)
                        n1189 = Square Root(x=w619) -> (sqrt(x)=w604:dbl)
                      }
                      frame True {
                        n1190 = global read "G_rio.vi" "gps_pos 1"() -> (w653:dbl[])
                        n1191 = global read "G_rio.vi" "gps_pos 2"() -> (w640:dbl[])
                        n1192 = Add(x=w653, y=w640) -> (x+y=w655:dbl[])
                        n1193 = Index Array(array=w653, index #1=0 ("index"), index #3=9 ("index"), index #4=7 ("index")) -> (element #1=w652:dbl, element #2=w651:dbl, element #3=w635:dbl, element #4=w630:dbl)  [unwired: 1 in]
                        n1194 = Index Array(array=w640, index #1=0 ("index"), index #3=9 ("index"), index #4=7 ("index")) -> (element #1=w641:dbl, element #2=w642:dbl, element #3=w634:dbl, element #4=w627:dbl)  [unwired: 1 in]
                        n1195 = feedback #28(w652) -> (w650:dbl)
                        n1196 = feedback-in #28(w652) -> ()
                        n1197 = feedback #29(w641) -> (w643:dbl)
                        n1198 = feedback-in #29(w641) -> ()
                        n1199 = Greater?(x=w630, y=10.0) -> (0:w626:bool)
                        n1200 = Greater?(x=w627, y=10.0) -> (0:w625:bool)
                        n1201 = Not Equal?(x=w652, y=w650) -> (x != y?=w649:bool)
                        n1202 = Not Equal?(x=w641, y=w643) -> (x != y?=w644:bool)
                        n1203 = And(x=w626, y=w625) -> (x .and. y?=w624:bool)
                        n1204 = Not Equal To 0?(x=w651) -> (x != 0?=w648:bool)
                        n1205 = Max & Min(x=w635, y=w634) -> (max(x,y)=w622:dbl)  [unwired: 1 out]
                        n1206 = Not Equal To 0?(x=w642) -> (x != 0?=w645:bool)
                        n1207 = And(x=w649, y=w648) -> (x .and. y?=w623:bool)
                        n1208 = And(x=w644, y=w645) -> (x .and. y?=w639:bool)
                        n1209 = Less?(x=w622, y=1.0) -> (x < y?=w620:bool)
                        n1210 = disable-structure shown="Enabled" {
                          disable-tunnel: w639 -> [w660 w661]
                          disable-tunnel: [w659 w662] -> w638
                          disable-tunnel: w624 -> [w658 _]
                          disable-tunnel: w623 -> [w657 w663]
                          disable-tunnel: w620 -> [w656 _]
                          frame Disabled {
                            n1211 = Compound Arithmetic op=AND(w656, w657, w660, w658) -> (w659:bool)
                          }
                          frame Enabled {
                            n1212 = And(x=w663, y=w661) -> (x .and. y?=w662:bool)
                          }
                        }
                        n1213 = Multiply(x=w655, y=0.5) -> (x*y=w633:dbl[])
                      }
                    }
                    n1214 = global read "G_rio.vi" "VS_CAN"() -> (w529:dbl)
                    n1215 = Greater Or Equal To 0?(x=w529) -> (x >= 0?=w530:bool)
                    n1216 = Select(t=0.0, s=w530, f=3.141592653589793) -> (s? t:f=w527:dbl)
                    n1217 = local write "pos_gps"(w523) -> ()
                    n1218 = local write "get position"(w524) -> ()
                    n1219 = local write "get heading"(w525) -> ()
                    n1220 = call "headingoperater.vi"("h1"=w527, "h2"=w528) -> ("h2-h1"=w526:dbl)  [unwired: 8 in, 1 out]
                    n1221 = local write "h_gps"(w526) -> ()
                  }
                  frame #1 {
                    n1222 = local read "dt"() -> (w665:dbl)
                    n1223 = Greater Than 0?(x=w665) -> (x > 0?=w664:bool)
                    n1224 = case shown="True" w664 {
                      tunnel: w667 -> [w668 w671]
                      tunnel: [w668 w670] -> w666
                      frame False {
                      }
                      frame True {
                        n1225 = flat-sequence {
                          tunnel: w671 -> [w705]
                          tunnel: [w683] -> w669
                          tunnel: [w733] -> w670
                          tunnel: w669 -> [w732]
                          frame #0 {
                            n1226 = Index Array(array=w705, index #1=0 ("index"), index #2=3 ("index"), index #3=1 ("index"), index #4=3 ("index")) -> (element #1=w699:dbl, element #2=w697:dbl, element #3=w693:dbl, element #4=w688:dbl)
                            n1227 = global read "G_rio.vi" "VS_CAN"() -> (w677:dbl)
                            n1228 = global read "G_rio.vi" "VS_CAN"() -> (w673:dbl)
                            n1229 = local read "vgain"() -> (w678:dbl)
                            n1230 = Equal To 0?(x=w673) -> (x = 0?=w674:bool)
                            n1231 = case shown="True" w674 {
                              tunnel: [w706 _] -> w672
                              frame False {
                                n1232 = global read "G_rio.vi" "yaw_rate"() -> (w709:dbl)
                                n1233 = local read "hbias"() -> (w710:dbl)
                                n1234 = Subtract(x=w709, y=w710) -> (x-y=w707:dbl)
                                n1235 = Negate(x=w707) -> (-x=w708:dbl)
                                n1236 = call "angleconv.vi"("deg"=w708) -> ("rad"=w706:dbl)  [unwired: 9 in, 1 out]
                              }
                              frame True {
                                w714 = u64 18446744073709551615
                                n1237 = local read "hcount"() -> (w717:u64)
                                n1238 = local read "hbias"() -> (w720:dbl)
                                n1239 = Increment(x=w717) -> (x+1=w716:u64)
                                n1240 = global read "G_rio.vi" "yaw_rate"() -> (w711:dbl)
                                n1241 = Not Equal?(x=w717, y=w714) -> (x != y?=w715:bool)
                                n1242 = Multiply(x=w720, y=w717) -> (x*y=w719:dbl)
                                n1243 = Add(x=w711, y=w719) -> (x+y=w718:dbl)
                                n1244 = Select(t=w716, s=w715, f=w714) -> (s? t:f=w713:u64)
                                n1245 = local write "hcount"(w713) -> ()
                                n1246 = Divide(x=w718, y=w713) -> (x/y=w712:dbl)
                                n1247 = local write "hbias"(w712) -> ()
                              }
                            }
                            n1248 = Multiply(x=w677, y=w678) -> (x*y=w676:dbl)
                            n1249 = Cosine(x=w697) -> (cos(x)=w703:dbl)
                            n1250 = Sine(x=w697) -> (sin(x)=w696:dbl)
                            n1251 = Divide(x=w676, y=3.6) -> (x/y=w675:dbl)
                            n1252 = local read "dt"() -> (w702:dbl)
                            n1253 = Multiply(x=w675, y=w702) -> (x*y=w698:dbl)
                            n1254 = Multiply(x=w703, y=w698) -> (x*y=w700:dbl)
                            n1255 = Multiply(x=w698, y=w696) -> (x*y=w695:dbl)
                            n1256 = Add(x=w699, y=w700) -> (x+y=w692:dbl)
                            n1257 = Add(x=w695, y=w693) -> (x+y=w691:dbl)
                            n1258 = local read "dt"() -> (w686:dbl)
                            n1259 = Multiply(x=w686, y=w672) -> (x*y=w679:dbl)
                            n1260 = local write "rt"(w679) -> ()
                            n1261 = call "headingoperater.vi"("h1"=w679, "h2"=w688) -> ("h2+h1"=w687:dbl)  [unwired: 8 in, 1 out]
                            n1262 = Build Array(w692, w691, w675, w687, w672) -> (w683:dbl[])
                            n1263 = Index Array(array=w683, index=3) -> (element=w682:dbl)
                            n1264 = local read "h_gps"() -> (w681:dbl)
                            n1265 = call "headingoperater.vi"("h1"=w682, "h2"=w681) -> ("h2-h1"=w685:dbl)  [unwired: 8 in, 1 out]
                            n1266 = Absolute Value(x=w685) -> (abs(x)=w680:dbl)
                            n1267 = local write "heading error"(w680) -> ()
                          }
                          frame #1 {
                            n1268 = local read "get heading"() -> (w740:bool)
                            n1269 = local read "get position"() -> (w739:bool)
                            n1270 = global read "G_rio.vi" "VS_CAN"() -> (w738:dbl)
                            n1271 = local read "POS init"() -> (w725:bool)
                            n1272 = local read "heading error"() -> (w728:dbl)
                            n1273 = case shown="False" w725 {
                              tunnel: w740 -> [w743 w750]
                              tunnel: w739 -> [w747 w749]
                              tunnel: [w741 w748] -> w735
                              frame False {
                                n1274 = local read "heading error"() -> (w744:dbl)
                                n1275 = Less?(x=w744, y=0.05) -> (x < y?=w745:bool)
                                n1276 = And(x=w743, y=w745) -> (x .and. y?=w742:bool)
                                n1277 = Or(x=w742, y=w747) -> (x .or. y?=w741:bool)
                              }
                              frame True {
                                n1278 = disable-structure shown="Enabled" {
                                disable-tunnel: w750 -> [w753 w755]
                                disable-tunnel: w749 -> [w752 w754]
                                disable-tunnel: [w751 w756] -> w748
                                frame Disabled {
                                n1279 = And(x=w753, y=w752) -> (x .and. y?=w751:bool)
                                }
                                frame Enabled {
                                n1280 = Or(x=w755, y=w754) -> (x .or. y?=w756:bool)
                                }
                                }
                              }
                            }
                            n1281 = local read "POS init"() -> (w726:bool)
                            n1282 = Less?(x=w728, y=1.0) -> (x < y?=w727:bool)
                            n1283 = Or(x=w727, y=w726) -> (x .or. y?=w729:bool)
                            n1284 = Absolute Value(x=w738) -> (abs(x)=w737:dbl)
                            n1285 = Greater?(x=w737, y=5.0) -> (0:w734:bool)
                            n1286 = And(x=w735, y=w734) -> (x .and. y?=w730:bool)
                            n1287 = And(x=w730, y=w729) -> (x .and. y?=w723:bool)
                            n1288 = Select(t=FALSE, s="GPS init", f=w723) -> (s? t:f=w722:bool)
                            n1289 = case shown="True" w722 {
                              tunnel: [w760 w789] -> w733
                              tunnel: w732 -> [w761 w792]
                              frame False {
                                n1290 = global read "G_rio.vi" "VS_CAN"() -> (w764:dbl)
                                n1291 = local read "POS init"() -> (w763:bool)
                                n1292 = Equal To 0?(x=w764) -> (x = 0?=w762:bool)
                                n1293 = local read "GPS init"() -> (w757:bool)
                                n1294 = And(x=w763, y=w762) -> (x .and. y?=w759:bool)
                                n1295 = Or(x=w759, y=w757) -> (x .or. y?=w758:bool)
                                n1296 = case shown="False" w758 {
                                tunnel: w761 -> [w765 w766]
                                tunnel: [w765 w768] -> w760
                                tunnel: w757 -> [_ w767]
                                frame False {
                                }
                                frame True {
                                n1297 = case shown="False" w767 {
                                tunnel: [w779 w788] -> w768
                                tunnel: w766 -> [w774 w782]
                                frame True {
                                n1298 = Index Array(array=w774, index #1=2 ("index")) -> (element #2=w769:dbl, element #3=w772:dbl)  [unwired: 2 in, 1 out]
                                n1299 = local write "GPS init"(FALSE ("GPS init")) -> ()
                                n1300 = local read "pos_gps"() -> (w775:dbl[])
                                n1301 = Index Array(array=w775, index #1=2 ("index")) -> (element #1=w777:dbl, element #2=w776:dbl)  [unwired: 1 in]
                                n1302 = local read "h_gps"() -> (w770:dbl)
                                n1303 = Build Array(w777, w776, w769, w770, w772) -> (w779:dbl[])
                                }
                                frame False {
                                w781 = 0.0 ("element")
                                n1304 = Index Array(array=w782, index=3) -> (element=w780:dbl)
                                n1305 = local read "pos_gps"() -> (w784:dbl[])
                                n1306 = Index Array(array=w784, index #1=2 ("index")) -> (element #1=w786:dbl, element #2=w785:dbl)  [unwired: 1 in]
                                n1307 = Build Array(w786, w785, w781, w780, w781) -> (w788:dbl[])
                                }
                                }
                                }
                                }
                              }
                              frame True {
                                n1308 = flat-sequence {
                                tunnel: w792 -> [w793]
                                tunnel: [w793] -> w791
                                tunnel: w791 -> [w834]
                                tunnel: [w834] -> w790
                                tunnel: w790 -> [w861]
                                tunnel: [w865] -> w789
                                frame #0 {
                                w802 = 0.0 ("element")
                                w806 = 0.0 ("element")
                                w808 = 0.0 ("element")
                                w810 = 0.0 ("element")
                                w812 = 0.0 ("element")
                                n1309 = Index Array(array=w793, index #1=3 ("index"), index #2=2 ("index"), index #3=3 ("index"), index #4=2 ("index")) -> (element #1=w822:dbl, element #2=w824:dbl, element #3=w827:dbl, element #4=w816:dbl)
                                n1310 = Negate(x=w824) -> (-x=w823:dbl)
                                n1311 = Sine & Cosine(0:w827) -> (1:w819:dbl, 2:w817:dbl)
                                n1312 = Multiply(x=w823, y=w819) -> (x*y=w820:dbl)
                                n1313 = Multiply(x=w817, y=w816) -> (x*y=w815:dbl)
                                n1314 = Cosine(x=w822) -> (cos(x)=w821:dbl)
                                n1315 = Build Array(w812, w812, w821, w820, 0.0 ("element")) -> (w814:dbl[])
                                n1316 = Build Array(w810, w810, w819, w815, 0.0 ("element")) -> (w813:dbl[])
                                n1317 = Build Array(w808, w808, w808, w808, w808) -> (w807:dbl[])
                                n1318 = Build Array(w806, w806, w806, w806, 1.0 ("element")) -> (w804:dbl[])
                                n1319 = Build Array(w802, w802, w802, w802, w802) -> (w803:dbl[])
                                n1320 = Build Array(w814, w813, w807, w804, w803) -> (w800:dbl[][])
                                n1321 = call-poly <vilib>:"Array To Matrix.vi"("Real 2D Array"=w800) -> ("Real Matrix"=w798:T15)
                                n1322 = global read "G_rio.vi" "P"() -> (w801:T15)
                                n1323 = Transpose Matrix(1:w798) -> (0:w797:T15)
                                n1324 = call-poly <vilib>:"Multiply.vi"("Real Matrix B"=w801, "Real Matrix A"=w798) -> ("A * B"=w799:T15)
                                n1325 = call-poly <vilib>:"Multiply.vi"("Real Matrix B"=w797, "Real Matrix A"=w799) -> ("A * B"=w796:T15)
                                n1326 = global read "G_rio.vi" "Q"() -> (w795:T15)
                                n1327 = call-poly <vilib>:"Add.vi"("Real Matrix B"=w795, "Real Matrix A"=w796) -> ("A + B"=w794:T15)
                                n1328 = global write "G_rio.vi" "Pp"(w794) -> ()
                                }
                                frame #1 {
                                n1329 = global read "G_rio.vi" "Pp"() -> (w859:T15)
                                n1330 = global read "G_rio.vi" "H"() -> (w858:T15)
                                n1331 = Array Subset(array=w834, index=0, length=2) -> (w841:dbl[])
                                n1332 = global read "G_rio.vi" "H"() -> (w853:T15)
                                n1333 = local read "pos_gps"() -> (w837:dbl[])
                                n1334 = call-poly <vilib>:"Multiply.vi"("Real Matrix B"=w859, "Real Matrix A"=w858) -> ("A * B"=w857:T15)
                                n1335 = Transpose Matrix(1:w858) -> (0:w856:T15)
                                n1336 = global read "G_rio.vi" "Pp"() -> (w852:T15)
                                n1337 = Transpose Matrix(1:w853) -> (0:w851:T15)
                                n1338 = local read "heading error"() -> (w846:dbl)
                                n1339 = call-poly <vilib>:"Multiply.vi"("Real Matrix B"=w851, "Real Matrix A"=w852) -> ("A * B"=w850:T15)
                                n1340 = call-poly <vilib>:"Multiply.vi"("Real Matrix B"=w856, "Real Matrix A"=w857) -> ("A * B"=w855:T15)
                                n1341 = Array Subset(array=w837, index=2, length=2) -> (w840:dbl[])
                                n1342 = global read "G_rio.vi" "R"() -> (w854:T15)
                                n1343 = Subtract(x=w840, y=w841) -> (x-y=w842:dbl[])
                                n1344 = call-poly <vilib>:"Add.vi"("Real Matrix B"=w854, "Real Matrix A"=w855) -> ("A + B"=w849:T15)
                                n1345 = Square(x=w842) -> (x^2=w843:dbl[])
                                n1346 = Add Array Elements(numeric array=w843) -> (sum=w844:dbl)
                                n1347 = call-poly <vilib>:"Inverse Matrix.vi"("Input Matrix"=w849) -> ("Inverse Matrix"=w848:T15)  [unwired: 1 in, 1 out]
                                n1348 = call-poly <vilib>:"Multiply.vi"("Real Matrix B"=w848, "Real Matrix A"=w850) -> ("A * B"=w847:T15)
                                n1349 = Square Root(x=w844) -> (sqrt(x)=w833:dbl)
                                n1350 = Less?(x=w846, y=0.05) -> (x < y?=w831:bool)
                                n1351 = global write "G_rio.vi" "K"(w847) -> ()
                                n1352 = Less?(x=w833, y=2.5) -> (x < y?=w830:bool)
                                n1353 = And(x=w831, y=w830) -> (x .and. y?=w829:bool)
                                n1354 = case shown="True" w829 {
                                frame False {
                                }
                                frame True {
                                n1355 = local write "POS init"(FALSE ("Kalman init")) -> ()
                                }
                                }
                                }
                                frame #2 {
                                n1356 = disable-structure shown="Enabled" {
                                disable-tunnel: [w883 w885] -> w863
                                disable-tunnel: w861 -> [_ w894]
                                frame Disabled {
                                n1357 = local read "get position"() -> (w883:bool)
                                }
                                frame Enabled {
                                n1358 = disable-structure shown="Enabled" {
                                disable-tunnel: [w900 TRUE ("Kalman init")] -> w887
                                frame Disabled {
                                n1359 = local read "POS init"() -> (w900:bool)
                                }
                                frame Enabled {
                                }
                                }
                                n1360 = Array Subset(array=w894, index=0, length=2) -> (w892:dbl[])
                                n1361 = local read "pos_gps"() -> (w897:dbl[])
                                n1362 = Array Subset(array=w897, index=2, length=2) -> (w893:dbl[])
                                n1363 = Subtract(x=w893, y=w892) -> (x-y=w891:dbl[])
                                n1364 = Square(x=w891) -> (x^2=w890:dbl[])
                                n1365 = Add Array Elements(numeric array=w890) -> (sum=w889:dbl)
                                n1366 = Square Root(x=w889) -> (sqrt(x)=w884:dbl)
                                n1367 = local write "pos error"(w884) -> ()
                                n1368 = Less?(x=w884, y=3.0) -> (x < y?=w886:bool)
                                n1369 = Or(x=w887, y=w886) -> (x .or. y?=w885:bool)
                                }
                                }
                                n1370 = disable-structure shown="Enabled" {
                                disable-tunnel: [w877 w878] -> w864
                                frame Disabled {
                                n1371 = local read "get heading"() -> (w877:bool)
                                }
                                frame Enabled {
                                n1372 = local read "POS init"() -> (w879:bool)
                                n1373 = local read "heading error"() -> (w881:dbl)
                                n1374 = Less?(x=w881, y=0.1) -> (x < y?=w880:bool)
                                n1375 = Or(x=w880, y=w879) -> (x .or. y?=w878:bool)
                                }
                                }
                                n1376 = Index Array(array=w861, index=3) -> (element=w868:dbl)
                                n1377 = global read "G_rio.vi" "K"() -> (w876:T15)
                                n1378 = global read "G_rio.vi" "H"() -> (w875:T15)
                                n1379 = global read "G_rio.vi" "Pp"() -> (w873:T15)
                                n1380 = call-poly <vilib>:"Multiply.vi"("Real Matrix B"=w875, "Real Matrix A"=w876) -> ("A * B"=w874:T15)
                                n1381 = call-poly <vilib>:"Multiply.vi"("Real Matrix B"=w873, "Real Matrix A"=w874) -> ("A * B"=w872:T15)
                                n1382 = global read "G_rio.vi" "Pp"() -> (w871:T15)
                                n1383 = call-poly <vilib>:"Subtract.vi"("Real Matrix B"=w872, "Real Matrix A"=w871) -> ("A - B"=w870:T15)
                                n1384 = global write "G_rio.vi" "P"(w870) -> ()
                                n1385 = case shown="True" w864 {
                                tunnel: w868 -> [w926 w933]
                                tunnel: [w926 w928] -> w862
                                frame False {
                                }
                                frame True {
                                n1386 = global read "G_rio.vi" "K"() -> (w932:T15)
                                n1387 = Index Array(array=w932, index (row)=3, index (col)=2 ("disabled index (col)")) -> (element=w929:dbl)
                                n1388 = local read "h_gps"() -> (w927:dbl)
                                n1389 = call "headingweightsum2.vi"("a"=w929, "h2"=w927, "h1"=w933) -> ("a*h2+(1-a)*h1"=w928:dbl)  [unwired: 8 in]
                                }
                                }
                                n1390 = case shown="True" w863 {
                                tunnel: w861 -> [w902 w914]
                                tunnel: [w902 w913] -> w867
                                tunnel: w862 -> [_ w903]
                                frame False {
                                }
                                frame True {
                                n1391 = disable-structure shown="Enabled" {
                                disable-tunnel: [w924 w925] -> w904
                                disable-tunnel: w903 -> [_ w925]
                                frame Disabled {
                                n1392 = local read "h_gps"() -> (w924:dbl)
                                }
                                frame Enabled {
                                }
                                }
                                n1393 = call-poly <vilib>:"Array To Matrix.vi"("Real 1D Array"=w914) -> ("Real Matrix (Column Vector)"=w918:T15)
                                n1394 = local read "pos_gps"() -> (w908:dbl[])
                                n1395 = global read "G_rio.vi" "H"() -> (w923:T15)
                                n1396 = call-poly <vilib>:"Multiply.vi"("Real Matrix B"=w918, "Real Matrix A"=w923) -> ("A * B"=w922:T15)
                                n1397 = Array Subset(array=w908, index=2, length=2) -> (w909:dbl[])
                                n1398 = Build Array (concatenate)(w909, w904) -> (w905:dbl[])
                                n1399 = call-poly <vilib>:"Array To Matrix.vi"("Real 1D Array"=w905) -> ("Real Matrix (Column Vector)"=w921:T15)
                                n1400 = call-poly <vilib>:"Subtract.vi"("Real Matrix B"=w922, "Real Matrix A"=w921) -> ("A - B"=w919:T15)
                                n1401 = global read "G_rio.vi" "K"() -> (w920:T15)
                                n1402 = call-poly <vilib>:"Multiply.vi"("Real Matrix B"=w919, "Real Matrix A"=w920) -> ("A * B"=w912:T15)
                                n1403 = call-poly <vilib>:"Multiply.vi"("Real Matrix A"=w912, "Real Scalar c"=0.25) -> ("c * A"=w910:T15)
                                n1404 = call-poly <vilib>:"Add.vi"("Real Matrix B"=w918, "Real Matrix A"=w910) -> ("A + B"=w917:T15)
                                n1405 = call-poly <vilib>:"Matrix To Array.vi"("Real Matrix"=w917) -> ("Real 2D Array"=w916:dbl[][])
                                n1406 = Index Array(array=w916, index (col)=0 ("disabled index (col)")) -> (element=w913:dbl[])  [unwired: 1 in]
                                }
                                }
                                n1407 = Replace Array Subset(array=w867, new element=w862, index=3) -> (w865:dbl[])
                                }
                                }
                              }
                            }
                          }
                        }
                      }
                    }
                  }
                }
              }
              frame Disabled {
                n1408 = flat-sequence {
                  tunnel: [w963] -> w955
                  tunnel: w956 -> [w964]
                  tunnel: w955 -> [w990]
                  tunnel: [w989] -> w954
                  tunnel: [w988] -> w952
                  tunnel: [w987] -> w951
                  tunnel: w954 -> [w1085]
                  tunnel: [w1085] -> w953
                  tunnel: w952 -> [w1077]
                  tunnel: w951 -> [w1076]
                  tunnel: w953 -> [w1098]
                  tunnel: [w1097] -> w950
                  tunnel: w950 -> [w1123]
                  tunnel: [w1123] -> w949
                  tunnel: [w1122] -> w948
                  tunnel: [w1121] -> w947
                  tunnel: [w1120] -> w946
                  tunnel: [w1119] -> w945
                  tunnel: [w1118] -> w944
                  tunnel: [w1226] -> w943
                  tunnel: w949 -> [w1226]
                  tunnel: w948 -> [w1219]
                  tunnel: w947 -> [w1220]
                  tunnel: w946 -> [w1213]
                  tunnel: w945 -> [w1212]
                  tunnel: w944 -> [w1209]
                  frame #0 {
                    n1409 = Index Array(array=w964, index=3) -> (element=w969:dbl)
                    n1410 = global read "G_rio.vi" "VS_CAN"() -> (w960:dbl)
                    n1411 = Equal To 0?(x=w960) -> (x = 0?=w959:bool)
                    n1412 = case shown="False" w959 {
                      tunnel: [w971 _] -> w958
                      frame False {
                        n1413 = global read "G_rio.vi" "yaw_rate"() -> (w974:dbl)
                        n1414 = local read "hbias"() -> (w975:dbl)
                        n1415 = Subtract(x=w974, y=w975) -> (x-y=w972:dbl)
                        n1416 = Negate(x=w972) -> (-x=w973:dbl)
                        n1417 = call "angleconv.vi"("deg"=w973) -> ("rad"=w971:dbl)  [unwired: 9 in, 1 out]
                      }
                      frame True {
                        w979 = u64 18446744073709551615
                        n1418 = local read "hcount"() -> (w982:u64)
                        n1419 = Increment(x=w982) -> (x+1=w981:u64)
                        n1420 = local read "hbias"() -> (w985:dbl)
                        n1421 = global read "G_rio.vi" "yaw_rate"() -> (w976:dbl)
                        n1422 = Not Equal?(x=w982, y=w979) -> (x != y?=w980:bool)
                        n1423 = Multiply(x=w985, y=w982) -> (x*y=w984:dbl)
                        n1424 = Add(x=w976, y=w984) -> (x+y=w983:dbl)
                        n1425 = Select(t=w981, s=w980, f=w979) -> (s? t:f=w978:u64)
                        n1426 = local write "hcount"(w978) -> ()
                        n1427 = Divide(x=w983, y=w978) -> (x/y=w977:dbl)
                        n1428 = local write "hbias"(w977) -> ()
                      }
                    }
                    n1429 = local read "dh_hat"() -> (w962:dbl)
                    n1430 = Subtract(x=w958, y=w962) -> (x-y=w968:dbl)
                    n1431 = local read "dt"() -> (w967:dbl)
                    n1432 = Multiply(x=w968, y=w967) -> (x*y=w957:dbl)
                    n1433 = local write "rt"(w957) -> ()
                    n1434 = call "headingoperater.vi"("h1"=w957, "h2"=w969) -> ("h2+h1"=w966:dbl)  [unwired: 8 in, 1 out]
                    n1435 = Replace Array Subset(array=w964, new element #1=w966, index #1=3 ("index"), new element #2=w958, index #2=4 ("index")) -> (w963:dbl[])
                  }
                  frame #1 {
                    n1436 = global read "G_rio.vi" "gps_vel 1"() -> (w1017:dbl[])
                    n1437 = global read "G_rio.vi" "gps_vel 2"() -> (w1006:dbl[])
                    n1438 = global read "G_rio.vi" "VS_CAN"() -> (w994:dbl)
                    n1439 = Index Array(array=w1017, index #1=1 ("index"), index #2=0 ("index"), index #3=0 ("index")) -> (element #1=w1012:dbl, element #2=w1001:dbl, element #3=w995:dbl)
                    n1440 = Index Array(array=w1006, index #1=0 ("index"), index #2=1 ("index"), index #3=0 ("index")) -> (element #1=w997:dbl, element #2=w1011:dbl, element #3=w1000:dbl)
                    n1441 = Equal?(x=w995, y=w997) -> (x = y?=w999:bool)
                    n1442 = Absolute Value(x=w994) -> (abs(x)=w993:dbl)
                    n1443 = Not Equal To 0?(x=w1011) -> (x != 0?=w1003:bool)
                    n1444 = feedback-in #30(w1001) -> ()
                    n1445 = feedback #30(0.0 ("Real Matrix Element")) -> (w1014:dbl)
                    n1446 = feedback #31(0.0 ("Real Matrix Element")) -> (w1009:dbl)
                    n1447 = feedback-in #31(w1000) -> ()
                    n1448 = Greater?(x=w1001, y=w1014) -> (0:w1004:bool)
                    n1449 = Greater?(x=w1000, y=w1009) -> (0:w1002:bool)
                    n1450 = Not Equal To 0?(x=w1012) -> (x != 0?=w1005:bool)
                    n1451 = Greater?(x=w993, y=5.0) -> (0:w991:bool)
                    n1452 = Compound Arithmetic op=AND(w991, w1005, w1004, w999, w1003, w1002) -> (w986:bool)
                    n1453 = local write "get heading"(w986) -> ()
                    n1454 = case shown="True" w986 {
                      tunnel: w990 -> [w1024 w1050]
                      tunnel: [w1025 w1042] -> w988
                      tunnel: [w1024 w1050] -> w989
                      tunnel: [w1023 w1047] -> w987
                      frame False {
                        n1455 = local read "initH"() -> (w1021:dbl)
                        n1456 = Multiply(x=0.9875 ("value"), y=w1021) -> (x*y=w1020:dbl)
                        n1457 = Add(x=0.011 ("value"), y=w1020) -> (x+y=w1018:dbl)
                        n1458 = local read "dh"() -> (w1023:dbl)
                        n1459 = Compound Arithmetic op=MULTIPLY(w1018, w1023) -> (w1025:dbl)
                      }
                      frame True {
                        w1049 = 0.001745329251994  # 0.1deg
                        n1460 = Index Array(array=w1050, index=3) -> (element=w1052:dbl)
                        n1461 = global read "G_rio.vi" "gps_vel 1"() -> (w1064:dbl[])
                        n1462 = global read "G_rio.vi" "gps_vel 2"() -> (w1062:dbl[])
                        n1463 = global read "G_rio.vi" "VS_CAN"() -> (w1031:dbl)
                        n1464 = global read "G_rio.vi" "VS_CAN"() -> (w1056:dbl)
                        n1465 = Greater Or Equal To 0?(x=w1056) -> (x >= 0?=w1057:bool)
                        n1466 = Index Array(array=w1064, index #1=4 ("index"), index #2=2 ("index")) -> (element #1=w1046:dbl, element #2=w1039:dbl)
                        n1467 = Index Array(array=w1062, index #1=4 ("index"), index #2=2 ("index")) -> (element #1=w1044:dbl, element #2=w1038:dbl)
                        n1468 = Add(x=w1039, y=w1038) -> (x+y=w1037:dbl)
                        n1469 = call "angleconv.vi"("deg"=w1046) -> ("rad"=w1045:dbl)  [unwired: 9 in, 1 out]
                        n1470 = call "angleconv.vi"("deg"=w1044) -> ("rad"=w1043:dbl)  [unwired: 9 in, 1 out]
                        n1471 = Select(t=0.0, s=w1057, f=3.141592653589793) -> (s? t:f=w1054:dbl)
                        n1472 = Absolute Value(x=w1031) -> (abs(x)=w1030:dbl)
                        n1473 = Multiply(x=w1037, y=0.5) -> (x*y=w1029:dbl)
                        n1474 = call "headingweightsum.vi"("a"=0.5, "h1"=w1043, "h2"=w1045) -> ("a*h2+(1-a)*h1"=w1055:dbl)  [unwired: 8 in]
                        n1475 = Divide(x=w1029, y=w1030) -> (x/y=w1028:dbl)
                        n1476 = Decrement(x=w1028) -> (x-1=w1035:dbl)
                        n1477 = call "headingoperater.vi"("h1"=w1054, "h2"=w1055) -> ("h2-h1"=w1027:dbl)  [unwired: 8 in, 1 out]
                        n1478 = local write "h_gps"(w1027) -> ()
                        n1479 = Absolute Value(x=w1035) -> (abs(x)=w1034:dbl)
                        n1480 = call "headingoperater.vi"("h1"=w1027, "h2"=w1052) -> ("h2-h1"=w1042:dbl)  [unwired: 8 in, 1 out]
                        n1481 = Less?(x=w1034, y=0.05) -> (x < y?=w1032:bool)
                        n1482 = case shown="True" w1032 {
                          tunnel: w1028 -> [_ w1072]
                          frame False {
                          }
                          frame True {
                            w1066 = u64 18446744073709551615
                            n1483 = local read "vcount"() -> (w1069:u64)
                            n1484 = local read "vgain"() -> (w1074:dbl)
                            n1485 = Increment(x=w1069) -> (x+1=w1068:u64)
                            n1486 = Multiply(x=w1074, y=w1069) -> (x*y=w1073:dbl)
                            n1487 = Not Equal?(x=w1069, y=w1066) -> (x != y?=w1067:bool)
                            n1488 = Add(x=w1072, y=w1073) -> (x+y=w1071:dbl)
                            n1489 = Select(t=w1068, s=w1067, f=w1066) -> (s? t:f=w1065:u64)
                            n1490 = local write "vcount"(w1065) -> ()
                            n1491 = Divide(x=w1071, y=w1065) -> (x/y=w1070:dbl)
                            n1492 = local write "vgain"(w1070) -> ()
                          }
                        }
                        n1493 = Absolute Value(x=w1042) -> (abs(x)=w1048:dbl)
                        n1494 = call "angleconv.vi"("rad"=w1042) -> ("deg"=w1026:dbl)  [unwired: 9 in, 1 out]
                        n1495 = local write "heading error"(w1026) -> ()
                        n1496 = Greater?(x=w1049, y=w1048) -> (0:w1051:bool)
                        n1497 = case shown="True" w1051 {
                          frame False {
                          }
                          frame True {
                            n1498 = local write "initH"(0.0 ("initH")) -> ()
                          }
                        }
                        n1499 = local read "dh"() -> (w1047:dbl)
                      }
                    }
                  }
                  frame #2 {
                    n1500 = local write "dh"(w1077) -> ()
                    n1501 = Multiply(x=w1077, y="heading gain") -> (x*y=w1084:dbl)
                    n1502 = Negate(x="heading gain") -> (-x=w1081:dbl)
                    n1503 = Multiply(x=w1081, y=w1076) -> (x*y=w1083:dbl)
                    n1504 = feedback #32(0.0) -> (w1078:dbl)
                    n1505 = Compound Arithmetic op=ADD(w1084, w1083, w1078) -> (w1080:dbl)
                    n1506 = feedback-in #32(w1080) -> ()
                    n1507 = local write "dh_hat"(w1080) -> ()
                  }
                  frame #3 {
                    n1508 = Index Array(array=w1098, index #1=1 ("index"), index #2=3 ("index"), index #3=0 ("index")) -> (element #1=w1102:dbl, element #2=w1114:dbl, element #3=w1100:dbl)
                    n1509 = global read "G_rio.vi" "VS_CAN"() -> (w1087:dbl)
                    n1510 = local read "vgain"() -> (w1088:dbl)
                    n1511 = call "headingoperater.vi"("h1"=w1114, "h2"=1.5707963267948966) -> ("h2-h1"=w1113:dbl)  [unwired: 8 in, 1 out]
                    n1512 = Multiply(x=w1087, y=w1088) -> (x*y=w1086:dbl)
                    n1513 = Sine & Cosine(0:w1113) -> (1:w1110:dbl, 2:w1111:dbl)
                    n1514 = Divide(x=w1086, y=3.6) -> (x/y=w1091:dbl)
                    n1515 = Multiply(x=w1110, y=w1091) -> (x*y=w1108:dbl)
                    n1516 = Multiply(x=w1091, y=w1111) -> (x*y=w1109:dbl)
                    n1517 = local read "dy_hat"() -> (w1090:dbl)
                    n1518 = local read "dx_hat"() -> (w1089:dbl)
                    n1519 = Subtract(x=w1108, y=w1090) -> (x-y=w1107:dbl)
                    n1520 = Subtract(x=w1109, y=w1089) -> (x-y=w1105:dbl)
                    n1521 = local read "dt"() -> (w1106:dbl)
                    n1522 = Multiply(x=w1107, y=w1106) -> (x*y=w1103:dbl)
                    n1523 = Multiply(x=w1106, y=w1105) -> (x*y=w1101:dbl)
                    n1524 = Add(x=w1102, y=w1103) -> (x+y=w1095:dbl)
                    n1525 = Add(x=w1101, y=w1100) -> (x+y=w1093:dbl)
                    n1526 = Replace Array Subset(array=w1098, new element #1=w1095, index #1=1 ("index"), new element #2=w1093, index #2=0 ("index"), new element #3=w1091, index #3=2 ("index")) -> (w1097:dbl[])
                  }
                  frame #4 {
                    n1527 = global read "G_rio.vi" "gps_pos 1"() -> (w1150:dbl[])
                    n1528 = global read "G_rio.vi" "gps_pos 2"() -> (w1139:dbl[])
                    n1529 = global read "G_rio.vi" "VS_CAN"() -> (w1127:dbl)
                    n1530 = Index Array(array=w1150, index #1=1 ("index"), index #2=0 ("index"), index #3=0 ("index")) -> (element #1=w1145:dbl, element #2=w1134:dbl, element #3=w1128:dbl)
                    n1531 = Index Array(array=w1139, index #1=0 ("index"), index #2=1 ("index"), index #3=0 ("index")) -> (element #1=w1130:dbl, element #2=w1144:dbl, element #3=w1133:dbl)
                    n1532 = Equal?(x=w1128, y=w1130) -> (x = y?=w1132:bool)
                    n1533 = Absolute Value(x=w1127) -> (abs(x)=w1126:dbl)
                    n1534 = Not Equal To 0?(x=w1144) -> (x != 0?=w1136:bool)
                    n1535 = feedback #33(0.0 ("Real Matrix Element")) -> (w1147:dbl)
                    n1536 = feedback-in #33(w1134) -> ()
                    n1537 = feedback #34(0.0 ("Real Matrix Element")) -> (w1142:dbl)
                    n1538 = feedback-in #34(w1133) -> ()
                    n1539 = Greater?(x=w1134, y=w1147) -> (0:w1137:bool)
                    n1540 = Greater?(x=w1133, y=w1142) -> (0:w1135:bool)
                    n1541 = Not Equal To 0?(x=w1145) -> (x != 0?=w1138:bool)
                    n1542 = Greater?(x=w1126, y=5.0) -> (0:w1124:bool)
                    n1543 = Compound Arithmetic op=AND(w1124, w1138, w1137, w1132, w1136, w1135) -> (w1117:bool)
                    n1544 = local write "get position"(w1117) -> ()
                    n1545 = case shown="True" w1117 {
                      tunnel: w1123 -> [_ w1203]
                      tunnel: [w1166 w1184] -> w1122
                      tunnel: [w1167 w1185] -> w1120
                      tunnel: [1.0 w1175] -> w1118
                      tunnel: [w1162 w1187] -> w1121
                      tunnel: [w1161 w1186] -> w1119
                      frame False {
                        n1546 = local read "initP"() -> (w1157:dbl)
                        n1547 = local read "initP"() -> (w1160:dbl)
                        n1548 = Multiply(x=0.9 ("value"), y=w1157) -> (x*y=w1156:dbl)
                        n1549 = Multiply(x=w1160, y=0.9) -> (x*y=w1153:dbl)
                        n1550 = Add(x=w1156, y=0.01 ("value")) -> (x+y=w1154:dbl)
                        n1551 = Add(x=w1153, y=0.01 ("value")) -> (x+y=w1151:dbl)
                        n1552 = local read "dy"() -> (w1165:dbl)
                        n1553 = local read "dx"() -> (w1163:dbl)
                        n1554 = Compound Arithmetic op=MULTIPLY(w1163, w1151) -> (w1166:dbl)
                        n1555 = Compound Arithmetic op=MULTIPLY(w1154, w1165) -> (w1167:dbl)
                        n1556 = local read "dy"() -> (w1161:dbl)
                        n1557 = local read "dx"() -> (w1162:dbl)
                      }
                      frame True {
                        n1558 = global read "G_rio.vi" "gps_pos 1"() -> (w1192:dbl[])
                        n1559 = global read "G_rio.vi" "gps_pos 2"() -> (w1191:dbl[])
                        n1560 = Add(x=w1192, y=w1191) -> (x+y=w1202:dbl[])
                        n1561 = Index Array(array=w1203, index #1=0 ("index"), index #2=1 ("index")) -> (element #1=w1193:dbl, element #2=w1195:dbl)
                        n1562 = Multiply(x=w1202, y=0.5) -> (x*y=w1169:dbl[])
                        "pos_gps" <- w1169
                        n1563 = Index Array(array=w1169, index #1=3 ("index"), index #2=2 ("index"), index #3=9 ("index")) -> (element #1=w1198:dbl, element #2=w1197:dbl, element #3=w1171:dbl)
                        n1564 = local read "initP"() -> (w1177:dbl)
                        n1565 = Subtract(x=w1193, y=w1198) -> (x-y=w1184:dbl)
                        n1566 = Subtract(x=w1195, y=w1197) -> (x-y=w1185:dbl)
                        n1567 = Divide(x=0.9, y=w1171) -> (x/y=w1189:dbl)
                        n1568 = Square(x=w1184) -> (x^2=w1180:dbl)
                        n1569 = Square(x=w1185) -> (x^2=w1179:dbl)
                        n1570 = Not Equal To 0?(x=w1177) -> (x != 0?=w1178:bool)
                        n1571 = Max & Min(x=w1189, y=1.0) -> (min(x,y)=w1176:dbl)  [unwired: 1 out]
                        n1572 = Select(t=w1177, s=w1178, f=w1176) -> (s? t:f=w1175:dbl)
                        n1573 = local read "initH"() -> (w1182:dbl)
                        n1574 = Add(x=w1180, y=w1179) -> (x+y=w1170:dbl)
                        n1575 = Equal To 0?(x=w1182) -> (x = 0?=w1174:bool)
                        n1576 = Square Root(x=w1170) -> (sqrt(x)=w1168:dbl)
                        n1577 = Less?(x=w1170, y=1.0) -> (x < y?=w1173:bool)
                        n1578 = local write "pos error"(w1168) -> ()
                        n1579 = And(x=w1174, y=w1173) -> (x .and. y?=w1181:bool)
                        n1580 = case shown="True" w1181 {
                          frame False {
                          }
                          frame True {
                            n1581 = local write "initP"(0.0 ("initP")) -> ()
                            n1582 = local write "POS init"(FALSE ("Kalman init")) -> ()
                          }
                        }
                        n1583 = local read "dy"() -> (w1186:dbl)
                        n1584 = local read "dx"() -> (w1187:dbl)
                      }
                    }
                  }
                  frame #5 {
                    n1585 = local write "dy"(w1213) -> ()
                    n1586 = local write "dx"(w1219) -> ()
                    n1587 = Multiply(x=w1213, y="pos gain") -> (x*y=w1216:dbl)
                    n1588 = Multiply(x=w1219, y="pos gain") -> (x*y=w1223:dbl)
                    n1589 = Negate(x="pos gain") -> (-x=w1217:dbl)
                    n1590 = Negate(x="pos gain") -> (-x=w1222:dbl)
                    n1591 = Multiply(x=w1217, y=w1212) -> (x*y=w1218:dbl)
                    n1592 = Multiply(x=w1222, y=w1220) -> (x*y=w1221:dbl)
                    n1593 = feedback #35(0.0) -> (w1214:dbl)
                    n1594 = Compound Arithmetic op=ADD(w1216, w1218, w1214) -> (w1211:dbl)
                    n1595 = feedback-in #35(w1211) -> ()
                    n1596 = feedback #36(0.0) -> (w1225:dbl)
                    n1597 = Compound Arithmetic op=ADD(w1223, w1221, w1225) -> (w1208:dbl)
                    n1598 = feedback-in #36(w1208) -> ()
                    n1599 = Multiply(x=w1211, y=w1209) -> (x*y=w1210:dbl)
                    n1600 = Multiply(x=w1209, y=w1208) -> (x*y=w1207:dbl)
                    n1601 = local write "dy_hat"(w1210) -> ()
                    n1602 = local write "dx_hat"(w1207) -> ()
                  }
                }
                n1603 = Index Array(array=w943, index #1=1 ("index"), index #2=0 ("index"), index #3=2 ("index")) -> (element #1=w939:dbl, element #2=w938:dbl, element #3=w937:dbl, element #4=w936:dbl, element #5=w935:dbl)  [unwired: 2 in]
                n1604 = Build Array(w939, w938, w937, w936, w935) -> (w934:dbl[])
              }
            }
          }
          frame #2 {
            n1605 = flat-sequence {
              tunnel: w1228 -> [w1235]
              frame #0 {
                n1606 = local read "h_gps"() -> (w1236:dbl)
                n1607 = local read "dt"() -> (w1232:dbl)
                n1608 = Array Subset(array=w1235, index=0, length=2) -> (w1243:dbl[])
                "pos" <- w1243
                n1609 = Index Array(array=w1235, index=3) -> (element=w1240:dbl)
                n1610 = Greater Than 0?(x=w1232) -> (x > 0?=w1230:bool)
                n1611 = call "angleconv.vi"("rad"=w1240) -> ("deg"=→"Heading":dbl)  [unwired: 9 in, 1 out]
                n1612 = Greater?(x=1.0, y=w1232) -> (0:w1234:bool)
                n1613 = call "headingoperater.vi"("h1"=0.0, "h2"=w1236) -> ("h2+h1"=w1237:dbl)  [unwired: 8 in, 1 out]
                n1614 = local read "LCM"() -> (w1231:bool)
                n1615 = call "angleconv.vi"("rad"=w1237) -> ("deg"=→"H_GPS":dbl)  [unwired: 9 in, 1 out]
                n1616 = Compound Arithmetic op=AND(w1234, w1230, w1231) -> (w1229:bool)
                n1617 = case shown="True" w1229 {
                  tunnel: w1243 -> [w1253 _]
                  tunnel: w1240 -> [w1249 _]
                  tunnel: w1236 -> [w1248 _]
                  tunnel: w1235 -> [_ w1260]
                  frame False {
                    n1618 = global read "G_rio.vi" "VS_CAN"() -> (w1246:dbl)
                    n1619 = local read "pos_gps"() -> (w1252:dbl[])
                    n1620 = Array Subset(array=w1252, index=5, length=10) -> (w1257:dbl[])
                    n1621 = Array Subset(array=w1252, index=12, length=3) -> (w1254:dbl[])
                    n1622 = local read "map"() -> (w1247:i32)
                    n1623 = local read "dt"() -> (w1251:dbl)
                    n1624 = Build Array (concatenate)(w1257, w1254, w1253, w1251, w1247, w1246, w1249, w1248) -> (w1250:dbl[])
                    n1625 = shared-variable "veloster\\sharedvari.lvlib\\RIONAV"(w1250) -> ()  [unwired: 1 in, 1 out]
                  }
                  frame True {
                    n1626 = flat-sequence {
                      tunnel: w1260 -> [w1285]
                      frame #0 {
                        n1627 = Get Date/Time In Seconds() -> (seconds since 1Jan1904=w1276:timestamp)
                        n1628 = local read "file write"() -> (w1266:bool)
                        n1629 = local read "POS init"() -> (w1265:bool)
                        n1630 = To Double Precision Float(number=w1276) -> (double precision float=w1270:dbl)
                        n1631 = global read "G_rio.vi" "LCM_POS_T"() -> (w1284:T16)
                        n1632 = local read "dt"() -> (w1264:dbl)
                        n1633 = Select(t=0.0, s=w1265, f=w1264) -> (s? t:f=w1262:dbl)
                        n1634 = Unbundle By Name(w1284) -> ("hash"=w1281:i64)
                        n1635 = Multiply(x=w1270, y=1000000.0) -> (x*y=w1268:dbl)
                        n1636 = Array To Cluster(array=w1285) -> (cluster=w1283:T17)
                        n1637 = To Quad Integer(1:w1268) -> (0:w1267:i64)
                        n1638 = call "hash.vi"("input"=w1281) -> ("output"=w1280:i64)  [unwired: 10 in]
                        n1639 = Unbundle(w1283) -> ("Real 2D Array[0]"=w1275:dbl, "Real 2D Array[1]"=w1274:dbl, "Real 2D Array[2]"=w1273:dbl, "Real 2D Array[3]"=w1272:dbl, "Real 2D Array[4]"=w1271:dbl)
                        n1640 = Bundle(cluster=w1284, "hash"=w1280, "sys time"=w1267, "dt"=w1262, "x"=w1275, "y"=w1274, "speed"=w1273, "heading"=w1272, "yaw_rate"=w1271) -> (w1261:T16)
                        n1641 = case shown="True" w1266 {
                          tunnel: w1261 -> [_ w1286]
                          frame False {
                          }
                          frame True {
                            n1642 = local read "data write"() -> (w1287:refnum<file>)
                            n1643 = Write to Binary File(file (use dialog)=w1287, data=w1286) -> ()  [unwired: 4 in, 3 out]
                          }
                        }
                        n1644 = Flatten To String(anything=w1261, prepend array or string size? (T)=FALSE) -> (data string=w1278:string)  [unwired: 2 in, 2 out]
                        n1645 = global read "G_rio.vi" "LCM"() -> (w1277:T4)
                        n1646 = call "LCM_send.vi"("DATA"=w1278, "ID"="POS_T", "LCM"=w1277) -> ()  [unwired: 6 in, 3 out]
                      }
                    }
                  }
                }
              }
            }
          }
        }
      }
    }
  }
